vi "TC.vi"() -> ()   [LabVIEW 2013]
uses:
  Lib/Lib.llb/CS mode.ctl
  Lib/Lib.llb/R.ctl
  Lib/Lib.llb/T.ctl
  Lib/Lib.llb/Calibrations.ctl
  Lib/Lib.llb/CS.lvclass
  Lib/Lib.llb/PID Settings.ctl
  Lib/Lib.llb/AVS_exc_n_ranges.ctl
  Lib/Lib.llb/AVS_excitation.ctl
  Lib/Lib.llb/AVS47_range.ctl
  Lib/Lib.llb/Ch descriptions.ctl
  Lib/Lib.llb/Cursor Controls.ctl
  Lib/Lib.llb/DataArray.ctl
  Lib/Lib.llb/Unit.ctl
  Lib/Lib.llb/Control 6.ctl
  Lib/Lib.llb/Control 4.ctl
  Lib/Lib.llb/Control 8.ctl
  Lib/Lib.llb/VI FPO Ref.ctl
  Lib/support/Class ID ENUM.ctl
  Lib/Lib.llb/Type Descriptor Enumeration__ogtk.ctl
  Lib/Lib.llb/Refnum Subtype Enum__ogtk.ctl
  Lib/Lib.llb/Waveform Subtype Enum__ogtk.ctl
  Lib/Lib.llb/LV Data cluster.ctl
  Lib/Lib.llb/Action.ctl
  Write to DSC/TC to DSC/Typedefs/TC-cluster.ctl
  Lib/Lib.llb/TCS.lvclass
  Lib/Lib.llb/QCS.lvclass
  Lib/Lib.llb/CS Emulation.lvclass
  Lib/Lib.llb/PCS.lvclass
  Lib/Lib.llb/Byte Params.ctl
  Lib/Lib.llb/MView.lvlib
panel:
  out "R Array":dbl[](array[numeric])
  out "_SetControl":T1
  out "ControlNames":string[](array[string])
  out "VIRef":T2 {"Array DataType" format="%.0x"; "WaveForm Type" format="%.0x"; "RefNum Type" format="%.0x"; "DataType" format="%.0x"}
  out "VI called?":bool=TRUE
  out "Error code":u8
  out "_zBridgeSetNr":u8 caption="zBridge set nr."
  out "_zBridgeDll":path=path "C:/Users/Sasha/Dropbox/Labview/LC Software/ImpSoft-V5.2.2-multithreaded/ImpBridgeLabview/ImpBridgeDll.dll"
  in  "_String":string="^ Click the Run button to start the program "
  in  "Top Toolbar":enum32{"Page 1", "Page 2"}(tab)
  in  "Load config":bool
  in  "Start":bool
  in  "Load Data":bool
  in  "Pause":bool
  in  "Stop":bool
  in  "Copy to Clipboard":bool
  in  "Save config":bool
  in  "Clear all plots":bool
  in  "ColorBox":enum32{"Page 1", "Page 2"}(tab)
  in  "Colors":picture
  out "Color":u32(colorbox)
  in  "Graph-open popup":bool
  out "_CalibFilesPath":path=path "C:/avs-47/aaaa"
  out "_LogFilesPath":path
  out "_AVS_VISA":refnum<visa-resource-name>="COM3"
  in  "Minimize UI 2":bool
  out "VI Version":string="TC" caption="V"
  in  "Minimize UI 1":bool
  in  "Main Panel":enum32{"AVS"}(tab)
  in  "Graph Controls Bar":enum32{"Page 1"}(tab)
  in  "Mode Buttons":T7
  in  "Erase all":bool
  in  "Plot-Save All":bool
  in  "Plot-save-screen":bool
  in  "Channels Panel":T8(tab)=enum."All"
  out "T0":dbl=nan caption="T" format="%#.2p"
  out "R0":dbl caption="R" format="%.3p"
  out "R-Plot 0":cluster{dbl[], dbl[]}(graph) caption="R-Plot"
  out "T1":dbl=nan caption="T" format="%#.2p"
  out "R1":dbl caption="R" format="%.3p"
  out "R-Plot 1":cluster{dbl[], dbl[]}(graph) caption="R-Plot"
  out "T2":dbl=nan caption="T" format="%#.2p"
  out "R2":dbl caption="R" format="%.3p"
  out "R-Plot 2":cluster{dbl[], dbl[]}(graph) caption="R-Plot"
  out "T3":dbl=nan caption="T" format="%#.2p"
  out "R3":dbl caption="R" format="%.3p"
  out "R-Plot 3":cluster{dbl[], dbl[]}(graph) caption="R-Plot"
  out "T4":dbl=nan caption="T" format="%#.2p"
  out "R4":dbl caption="R" format="%.3p"
  out "R-Plot 4":cluster{dbl[], dbl[]}(graph) caption="R-Plot"
  out "T5":dbl=nan caption="T" format="%#.2p"
  out "R5":dbl caption="R" format="%.3p"
  out "R-Plot 5":cluster{dbl[], dbl[]}(graph) caption="R-Plot"
  out "T6":dbl=nan caption="T" format="%#.2p"
  out "R6":dbl caption="R" format="%.3p"
  out "R-Plot 6":cluster{dbl[], dbl[]}(graph) caption="R-Plot"
  out "T7":dbl=nan caption="T" format="%#.2p"
  out "R7":dbl caption="R" format="%.3p"
  out "R-Plot 7":cluster{dbl[], dbl[]}(graph) caption="R-Plot"
  out "T8":dbl=nan caption="T" format="%#.2p"
  out "R8":dbl caption="R" format="%.3p"
  out "R-Plot 8":cluster{dbl[], dbl[]}(graph) caption="R-Plot"
  out "T9":dbl=nan caption="T" format="%#.2p"
  out "R9":dbl caption="R" format="%.3p"
  out "R-Plot 9":cluster{dbl[], dbl[]}(graph) caption="R-Plot"
  out "T Cluster":T9 {"T9" format="%.2p"; "T8" format="%.2p"; "T7" format="%.2p"; "T6" format="%.2p"; "T5" format="%.2p"; "T4" format="%.2p"; "T3" format="%.2p"; "T2" format="%.2p"; "T1" format="%.2p"; "T0" format="%.2p"}
  in  "Sensor Names":T10={"AVS Name 0"="C_still", "AVS Name 1"="3K", "AVS Name 2"="Still", "AVS Name 3"="50mK", "AVS Name 4"="MC", "AVS Name 5"="MC", "AVS Name 6"="MC", "AVS Name 7"="", "AVS Name 8"="", "AVS Name 9"=""}
  in  "Edit Calibrations":T11
  in  "Sensor Calibrations":T12 {"Sensor 10" items=["No Calibration", "PT100", "PT1000", "RuO2 10k", "RuO2 1k5", "RuO2 2k", "Emulation R", "PT 1000", "RuO2-10K-NEW", "testCMN", "No Calibration"]; "Sensor 9" items=["No Calibration", "PT100", "PT1000", "RuO2 10k", "RuO2 1k5", "RuO2 2k", "Emulation R", "PT 1000", "RuO2-10K-NEW", "testCMN", "No Calibration"]; "Sensor 8" items=["No Calibration", "PT100", "PT1000", "RuO2 10k", "RuO2 1k5", "RuO2 2k", "Emulation R", "PT 1000", "RuO2-10K-NEW", "testCMN", "No Calibration"]; "Sensor 7" items=["No Calibration", "PT100", "PT1000", "RuO2 10k", "RuO2 1k5", "RuO2 2k", "Emulation R", "PT 1000", "RuO2-10K-NEW", "testCMN", "No Calibration"]; "Sensor 6" items=["No Calibration", "PT100", "PT1000", "RuO2 10k", "RuO2 1k5", "RuO2 2k", "Emulation R", "PT 1000", "RuO2-10K-NEW", "testCMN", "No Calibration"]; "Sensor 5" items=["No Calibration", "PT100", "PT1000", "RuO2 10k", "RuO2 1k5", "RuO2 2k", "Emulation R", "PT 1000", "RuO2-10K-NEW", "testCMN", "No Calibration"]; "Sensor 4" items=["No Calibration", "PT100", "PT1000", "RuO2 10k", "RuO2 1k5", "RuO2 2k", "Emulation R", "PT 1000", "RuO2-10K-NEW", "testCMN", "No Calibration"]; "Sensor 3" items=["No Calibration", "PT100", "PT1000", "RuO2 10k", "RuO2 1k5", "RuO2 2k", "Emulation R", "PT 1000", "RuO2-10K-NEW", "testCMN", "No Calibration"]; "Sensor 2" items=["No Calibration", "PT100", "PT1000", "RuO2 10k", "RuO2 1k5", "RuO2 2k", "Emulation R", "PT 1000", "RuO2-10K-NEW", "testCMN", "No Calibration"]; "Sensor 1" items=["No Calibration", "PT100", "PT1000", "RuO2 10k", "RuO2 1k5", "RuO2 2k", "Emulation R", "PT 1000", "RuO2-10K-NEW", "testCMN", "No Calibration"]}
  out "Units":T13
  out "R Cluster":T14={"R0"=0.0, "R1"=0.0, "R2"=-0.0, "R3"=0.0, "R4"=0.0, "R5"=0.0, "R6"=0.0, "R7"=0.0, "R8"=0.0, "R9"=0.0} {"R9" format="%.3p"; "R8" format="%.3p"; "R7" format="%.3p"; "R6" format="%.3p"; "R5" format="%.3p"; "R4" format="%.3p"; "R3" format="%.3p"; "R2" format="%.3p"; "R1" format="%.3p"; "R0" format="%.3p"}
  in  "AVS Scan Parameters":enum32{"Page 1", "Page 2"}(tab)
  in  "AVS Exc&Ranges":T15={"Excitation 0"=4, "Excitation 1"=4, "Excitation 2"=3, "Excitation 3"=3, "Excitation 4"=3, "Excitation 5"=3, "Excitation 6"=3, "Excitation 7"=3, "Range 0"=5, "Range 1"=5, "Range 2"=5, "Range 3"=5, "Range 4"=5, "Range 5"=5, "Range 6"=5, "Range 7"=5} {"Range 7" items=["n.a."=-1, "open"=0, "2 Ohm"=1, "20 Ohm"=2, "200 Ohm"=3, "2k Ohm"=4, "20k Ohm"=5, "200k Ohm"=6, "2M Ohm"=7]; "Range 6" items=["n.a."=-1, "open"=0, "2 Ohm"=1, "20 Ohm"=2, "200 Ohm"=3, "2k Ohm"=4, "20k Ohm"=5, "200k Ohm"=6, "2M Ohm"=7]; "Range 5" items=["n.a."=-1, "open"=0, "2 Ohm"=1, "20 Ohm"=2, "200 Ohm"=3, "2k Ohm"=4, "20k Ohm"=5, "200k Ohm"=6, "2M Ohm"=7]; "Range 4" items=["n.a."=-1, "open"=0, "2 Ohm"=1, "20 Ohm"=2, "200 Ohm"=3, "2k Ohm"=4, "20k Ohm"=5, "200k Ohm"=6, "2M Ohm"=7]; "Range 3" items=["n.a."=-1, "open"=0, "2 Ohm"=1, "20 Ohm"=2, "200 Ohm"=3, "2k Ohm"=4, "20k Ohm"=5, "200k Ohm"=6, "2M Ohm"=7]; "Range 2" items=["n.a."=-1, "open"=0, "2 Ohm"=1, "20 Ohm"=2, "200 Ohm"=3, "2k Ohm"=4, "20k Ohm"=5, "200k Ohm"=6, "2M Ohm"=7]; "Range 1" items=["n.a."=-1, "open"=0, "2 Ohm"=1, "20 Ohm"=2, "200 Ohm"=3, "2k Ohm"=4, "20k Ohm"=5, "200k Ohm"=6, "2M Ohm"=7]; "Range 0" items=["n.a."=-1, "open"=0, "2 Ohm"=1, "20 Ohm"=2, "200 Ohm"=3, "2k Ohm"=4, "20k Ohm"=5, "200k Ohm"=6, "2M Ohm"=7]; "Excitation 7" items=["none", "3 µV", "10 µV", "30 µV", "100 µV", "300 µV", "1 mV", "3 mV"]; "Excitation 6" items=["none", "3 µV", "10 µV", "30 µV", "100 µV", "300 µV", "1 mV", "3 mV"]; "Excitation 5" items=["none", "3 µV", "10 µV", "30 µV", "100 µV", "300 µV", "1 mV", "3 mV"]; "Excitation 4" items=["none", "3 µV", "10 µV", "30 µV", "100 µV", "300 µV", "1 mV", "3 mV"]; "Excitation 3" items=["none", "3 µV", "10 µV", "30 µV", "100 µV", "300 µV", "1 mV", "3 mV"]; "Excitation 2" items=["none", "3 µV", "10 µV", "30 µV", "100 µV", "300 µV", "1 mV", "3 mV"]; "Excitation 1" items=["none", "3 µV", "10 µV", "30 µV", "100 µV", "300 µV", "1 mV", "3 mV"]; "Excitation 0" items=["none", "3 µV", "10 µV", "30 µV", "100 µV", "300 µV", "1 mV", "3 mV"]}
  out "zBridge.Scan Phase":T18
  out "zBridge params":T19
  out "uPlots":T20
  out "zBridge.Active Channels":T21={"active Channel 0"=TRUE, "active Channel 1"=TRUE, "active Channel 2"=TRUE, "active Channel 3"=FALSE, "active Channel 4"=FALSE, "active Channel 5"=FALSE, "active Channel 6"=FALSE, "active Channel 7"=FALSE, "active Channel 8"=FALSE, "active Channel 9"=FALSE}
  out "Waveform Chart":T22(graph)
  in  "_CS_Address":u32
  in  "Edit calibration":bool
  in  "Convert R-T":bool
  out "T7":dbl caption="T=" format="%#.2p"
  in  "QuickR":dbl caption="R=" format="%_6g"
  in  "_QuickConvertCal":u16(ring) items=["No Calibration", "PT100", "PT1000", "RuO2 10k", "RuO2 1k5", "RuO2 2k", "Emulation R", "PT 1000", "RuO2-10K-NEW", "testCMN", "No Calibration"]
  out "_CSMode1List[i]":T23[](array[typedef]) caption="I_list[i]" min=-1.0
  out "CS.Automode Current":T23[](array[typedef]) min=-1.0
  in  "Lower Panel":enum32{"Page 1", "Page 2"}(tab)
  in  "Data History/RT Settings":enum32{"History", "Settings"}(tab)=enum."Settings"
  out "AVS names small":T10={"AVS Name 0"="3K", "AVS Name 1"="Still", "AVS Name 2"="50 mK", "AVS Name 3"="MC", "AVS Name 4"="MC", "AVS Name 5"="", "AVS Name 6"="", "AVS Name 7"="", "AVS Name 8"="", "AVS Name 9"=""}
  out "zBridge.Active channel":T24
  out "Small T Cluster":T25 caption="T" {"T0" format="%#.2p"; "T1" format="%#.2p"; "T2" format="%#.2p"; "T3" format="%#.2p"; "T4" format="%#.2p"; "T5" format="%#.2p"; "T6" format="%#.2p"; "T7" format="%#.2p"; "T8" format="%#.2p"; "T9" format="%#.2p"}
  out "Small R Cluster":T26 caption="R" {"R0" format="%#_5p"; "R1" format="%#_5p"; "R2" format="%#_5p"; "R3" format="%#_5p"; "R4" format="%#_5p"; "R5" format="%#_5p"; "R6" format="%#_5p"; "R7" format="%#_5p"; "R8" format="%#_5p"; "R9" format="%#_5p"}
  out "Time":dbl format="%<%X\n%x>T"
  in  "Runtime Settings":T27={"Read AVS channels from"=0, "Last Channel"=7, "Delay Between Scans"=0, "Stabilisation Delay"=5.0, "Averages"=2, "Data Memory"=25000, "Filter Graphs"=FALSE, "Y_min"=0.0, "Y_max"=2000000.0, "Plot type"=enum."T vs Time", "Allow neg R"=TRUE, "Miniplot Time"=30.0} {"Miniplot Time" min=0.0; "Delay Between Scans" format="%.0f s"; "Averages" min=1 max=1000; "Stabilisation Delay" min=0.5; "Last Channel" min=0 max=7 step=1; "Read AVS channels from" min=0 max=7 step=1; "Y_max" format="%#_6f"; "Y_min" min=0.0 format="%#_6f"; "Data Memory" min=3 max=50000}
  out "CS.Current Value":dbl[](array[numeric])
  in  "Data Array":T28=[{"R"=[], "T"=[], "Time"=[]}, {"R"=[0.0, 2.0], "T"=[], "Time"=[]}]
  out "T Array":dbl[](array[numeric])
  in  "_ScanData":dbl[](array[numeric])
  out "_I3SetPnt":dbl
  out "_CurrentsChanged":bool
  in  "_AVSRanges":T29={"Excitationl 0"=5, "Excitation 1"=5, "Excitation 2"=5, "Excitation 3"=5, "Excitation 4"=5, "Excitation 5"=5, "Excitation 6"=5, "Excitation 7"=5} caption="Ranges" {"Excitation 7" items=["n.a."=-1, "open"=0, "2 Ohm"=1, "20 Ohm"=2, "200 Ohm"=3, "2k Ohm"=4, "20k Ohm"=5, "200k Ohm"=6, "2M Ohm"=7]; "Excitation 6" items=["n.a."=-1, "open"=0, "2 Ohm"=1, "20 Ohm"=2, "200 Ohm"=3, "2k Ohm"=4, "20k Ohm"=5, "200k Ohm"=6, "2M Ohm"=7]; "Excitation 5" items=["n.a."=-1, "open"=0, "2 Ohm"=1, "20 Ohm"=2, "200 Ohm"=3, "2k Ohm"=4, "20k Ohm"=5, "200k Ohm"=6, "2M Ohm"=7]; "Excitation 4" items=["n.a."=-1, "open"=0, "2 Ohm"=1, "20 Ohm"=2, "200 Ohm"=3, "2k Ohm"=4, "20k Ohm"=5, "200k Ohm"=6, "2M Ohm"=7]; "Excitation 3" items=["n.a."=-1, "open"=0, "2 Ohm"=1, "20 Ohm"=2, "200 Ohm"=3, "2k Ohm"=4, "20k Ohm"=5, "200k Ohm"=6, "2M Ohm"=7]; "Excitation 2" items=["n.a."=-1, "open"=0, "2 Ohm"=1, "20 Ohm"=2, "200 Ohm"=3, "2k Ohm"=4, "20k Ohm"=5, "200k Ohm"=6, "2M Ohm"=7]; "Excitation 1" items=["n.a."=-1, "open"=0, "2 Ohm"=1, "20 Ohm"=2, "200 Ohm"=3, "2k Ohm"=4, "20k Ohm"=5, "200k Ohm"=6, "2M Ohm"=7]; "Excitationl 0" items=["n.a."=-1, "open"=0, "2 Ohm"=1, "20 Ohm"=2, "200 Ohm"=3, "2k Ohm"=4, "20k Ohm"=5, "200k Ohm"=6, "2M Ohm"=7]}
  out "_CSClassRef":refnum<class "CS.lvclass">
  in  "CS Indicators Panel":enum32{"Page 1", "Page 2"}(tab)
  out "CS.Automode 0":bool
  out "CS.Automode 1":bool
  out "QCS. I0 Mapping":T30(ring) caption="Output to"
  in  "uA 0":u32
  in  "CS Cannel Names":T31={"CS Name 0"="N.C.", "CS Name 1"="3K", "CS Name 2"="Still", "CS Name 3"="MC"}
  out "I0":T32={"uA"="000", "ON"=FALSE, "Gated"=FALSE, "current flows"=FALSE, "Error"=FALSE} caption="Ch0 -"
  in  "uA 3":u32
  in  "uA 2":u32
  in  "uA 1":u32
  out "CS.Automode 3":bool
  out "CS.Automode 2":bool
  out "I3":T32={"uA"="000", "ON"=FALSE, "Gated"=FALSE, "current flows"=FALSE, "Error"=FALSE} caption="Chn 3"
  out "I2":T32={"uA"="000", "ON"=FALSE, "Gated"=FALSE, "current flows"=FALSE, "Error"=FALSE} caption="Chn 2"
  out "I1":T32={"uA"="000", "ON"=FALSE, "Gated"=FALSE, "current flows"=FALSE, "Error"=FALSE} caption="Chn 1"
  out "_ExtVIReference":refnum<vi>
  out "Small I":cluster{"I1":dbl, "I2":dbl, "I3":dbl, "I4":dbl} caption="I" {"I1" format="%#.2f"; "I2" format="%#.2p"; "I3" format="%#.2p"; "I4" format="%#.2p"}
  out "CS.Actual Current":dbl[](array[numeric])
  in  "Save Data 2":bool
  in  "Show PID graph?":bool
  in  "Set Color":bool
  out "_ZBridgeUnit":string caption="Unit"
  out "_zBridgeParText":string caption="zBridge params/Error"
  out "_CurCalibrations":T33
  out "_LMBDown":bool
  in  "Side Panel":T34(tab)
  in  "Reload Calibrations":bool
  in  "zBridge settings":bool
  out "CS.ID":string
  out "CS status":errorcluster
  out "General Error":errorcluster caption="General status"
  in  "Bridge settings":T35={"Bridge Type"=enum."AVS47A (GPIB interface)", "AVS RS232 Port"="COM5", "AVS GPIB Address"="GPIB0::20::INSTR", "Calibrations Folder"=path "C:/LC Data/Calibrations"}
  in  "CS Settings":T36={"TCS RS232 Port"="COM1", "TCS_Imax"=5, "CS type"=enum."TCS", "CS.QCS Device Nr"=0}
  in  "Data Logging Settings":T37={"Log Files Folder"=path "C:/LC Data/Data", "Log Files Name"="LogAVS", "Automode Files Name"="calibration", "Filenames Suffix"="_%Y-%m-%d-%H-%M-%S", "Delimeter"="\t", "New File Interval"=7, "New File Interval Units"=enum."Days", "Date Format"="%Y-%m-%d %H:%M:%S", "External VI Path"=path "", "Query Description"=FALSE, "Run Description"="\n"}
  out "Bridge status":errorcluster
  in  "CS.QCS I0 Output":T38(ring) caption="Set Channel 0 output to"
  in  "CS.Mode":T39 caption="CS mode"
  out "_TimeOld":dbl format="%#_16g"
  in  "CS Modes Panel":T40(tab)=enum."Automatic 1"
  in  "CS.I3":T41={"Toggle ON/OFF"=FALSE, "Toggle Gated"=FALSE, "I"=0, "Range"=enum."x1 uA"} caption="Chn 3" {"I" max=100000 step=1}
  in  "CS.I2":T41={"Toggle ON/OFF"=FALSE, "Toggle Gated"=FALSE, "I"=0, "Range"=enum."x1 uA"} caption="Chn 2" {"I" max=100000 step=1}
  in  "CS.I1":T41={"Toggle ON/OFF"=FALSE, "Toggle Gated"=FALSE, "I"=0, "Range"=enum."x1 uA"} caption="Chn 1" {"I" max=100000 step=1}
  in  "CS.I0":T41={"Toggle ON/OFF"=FALSE, "Toggle Gated"=FALSE, "I"=0, "Range"=enum."x1 uA"} caption="Chn 0" {"I" max=100000 step=1}
  in  "CS.Mode1.PID Settings":T42={"FB on 2"=enum."3", "Proportional Gain"=3.0, "Integral Gain"=3.0, "Derivative Gain"=1.0, "Deadband"=0.1, "Feed Fwd Gain [uA/mK]"=0.0, "Integral Gain Bandwidth"=10.0, "Integral Gain Background"=1.0, "Current limit, [uA]"=1.0} {"Integral Gain Background" format="%#.6g"; "Integral Gain Bandwidth" format="%#.6g"; "Feed Fwd Gain [uA/mK]" format="%#.5g"; "Deadband" format="%#.5g"; "Derivative Gain" format="%#.6g"; "Integral Gain" format="%#.6g"; "Proportional Gain" format="%#.6g"; "Current limit, [uA]" format="%#.5g"}
  in  "CS.Mode1.Start":bool
  in  "CS.Mode1.List":T23[][](array[typedef]) min=-1.0
  out "CS.Mode1.PID Column":T43[](array[typedef])
  out "CS.Mode1.Row":T44[](array[typedef])=[TRUE, FALSE, FALSE, FALSE, FALSE, FALSE, FALSE, FALSE, FALSE, FALSE]
  out "CS.Mode1.PID Stabilized?":bool caption="SP reached?"
  out "CS.Mode1.PID Error":dbl=10.0 caption="Error" format="%#_6f"
  out "CS.Mode1.Slope":dbl caption="Slope" format="%#_3g %"
  out "CS.Mode1.Timer":dbl caption="Timer" format="%<%H:%M:%S>t"
  out "CS.Mode1.List:Count":i32=10 caption="/"
  out "CS.Mode1.List:Index":i32=10 caption="Point #"
  in  "CS.Mode1.Next":bool
  in  "CS.Mode1.Reset PID":bool
  in  "CS.Mode1.Auto Advance":bool=TRUE caption="Enable automatic sweeping/list iteration"
  in  "CS.Mode1.Settings":T45={"Bridge Channel"=0, "N averages"=10, "Delay Time"=10.0, "T stability"=0.3, "FB on"=enum."Temperature"} {"Delay Time" min=0.0 format="%#_g min"; "Bridge Channel" min=-1 max=9 step=1}
  in  "CS.Mode1.Call VI?":bool caption="Call Ext. VI"
  out "CS.Mode1.VI State":T46(ring) caption="- state"
  in  "CS.Mode1.Trigger all TC":bool caption="Trigger other running TC instances"
  in  "CS.Mode1.List:Prev":bool
  in  "CS.Mode1.List:Next":bool
  in  "CS.Mode1.List:To First":bool
  in  "CS.Mode1.List:Save":bool
  in  "CS.Mode1.List:Load":bool
  in  "CS.Mode1.Write To Log":bool
  in  "CS.Mode1.PID":cluster{"Enabled":bool}
  in  "CS.Mode1.List:Clear":bool
  in  "CS.Mode2.Settings":T47={"FB on"=enum."Temperature", "Bridge Channel"=0, "Hysteresis"=10} {"Hysteresis" max=100 format="%.0f %%"; "Bridge Channel" min=-1 max=9 step=1}
  in  "CS.Mode2.Start":bool
  in  "CS.Mode2.Add Row":bool
  in  "CS.Mode2.New Row":dbl[](array[numeric])=[0.0, 0.0, 0.0, 0.0, 0.0, 0.0] caption="New range" min=-1.0
  in  "CS.Mode2.List":dbl[][](array[numeric])=[[0.0, 0.0, 0.0, 0.0, 0.0, inf]] min=-1.0
  out "CS.Mode2.Row":T44[](array[typedef])=[TRUE, FALSE, FALSE, FALSE, FALSE, FALSE, FALSE, FALSE, FALSE, FALSE]
  in  "T Sweep":T48={"Start value"=200.0, "End value"=250.0, "Step"=10.0, "Current"=0.0, "I_next"=FALSE, "I_prev"=FALSE, "Interrrupt Sweep"=FALSE, "Start"=FALSE, "Boolean"=TRUE} {"Step" min=0.0; "End value" min=0.0; "Start value" min=0.0}
  # "Quick convert R->T:"
  # "Ohm"
  # "mK"
  # "Ch#"
  # "Miniplot"
  # "Channel parameters"
  # "Impedance"
  # "Unit"
  # "Type of sensor"
  # "T [mK]"
  # "Description"
  # "0"
  # "1"
  # "2"
  # "3"
  # "4"
  # "5"
  # "6"
  # "7"
  # "8"
  # "9"
  # "0"
  # "1"
  # "2"
  # "3"
  # "4"
  # "5"
  # "7"
  # "8"
  # "9"
  # "6"
  # "auto"
  # "auto"
  # "auto"
  # "auto"
  # "gated"
  # "gated"
  # "gated"
  # "gated"
  # "Status"
  # "Current source mode"
  # "Current source manual control"
  # "Current source automatic mode #1"
  # "Currents List"
  # "Settings"
  # "I0"
  # "I1"
  # "I2"
  # "I3"
  # "Status"
  # "On temperature stabilized"
  # "Current source automatic mode #2"
  # "Currents List"
  # "Settings"
  # "T0"
  # "T1"
  # "I0"
  # "I1"
  # "I2"
  # "I3"
  # "T0"
  # "T1"
  # "I0"
  # "I1"
  # "I2"
  # "I3"
  # "Ch3"
types:
  T1 = typedef "MView.lvlib/LV Data cluster.ctl" = cluster{"Name":string, "Scalar":string, "Array":string[][]}
  T2 = typedef "MView.lvlib/VI FPO Ref.ctl" = cluster{"Control Ref ID":refnum<vi>[], "Full Name":string[], "ClassID":T3[], "Short Name":string[], "DataType":T4[], "RefNum Type":T5[], "WaveForm Type":T6[], "Parent":i32[], "Array DataType":T4[], "Owning VI":refnum<vi>[], "Active?":bool[]}
  T3 = typedef "Class ID ENUM.ctl" = enum16{"<Null>", "1", "2", "Generic", "Decoration", "Text", "Control", "ColorBox", "Boolean", "RefNum", "Variant", "Path", "ListBox", "Table", "Array", "Picture", "ActiveXContainer", "Numeric", "Digital", "NamedNumeric", "ColorRamp", "Slide", "GraphOrChart", "WaveformChart", "WaveformGraph", "IntensityChart", "IntensityGraph", "String", "IOName", "ComboBox", "Cluster", "Panel", "Knob", "NumWithScale", "Ring", "Enum", "GObject", "Plot", "Cursor", "NumericText", "Scale", "ColorScale", "GraphScale", "ColorGraphScale", "TypedRefNum", "OldKnobScale", "MCListbox", "MeasureData", "BVTag", "DAQName", "VISAName", "IVIName", "SlideScale", "TabControl", "Page", "TabArrayTabControl", "ConPane", "57", "58", "59", "60", "61", "62", "63", "64", "SubPanel", "TreeControl", "67", "68", "69", "70", "71", "72", "73", "74", "75", "SplitterBar"}
  T4 = typedef "Type Descriptor Enumeration__ogtk.ctl" = enum8{"<Null>", "I8", "I16", "I32", "I64", "U8", "U16", "U32", "U64", "SGL", "DBL", "EXT", "CSG", "CDB", "CXT", "0x0F", "0x10", "0x11", "0x12", "0x13", "0x14", "Enum U8", "Enum U16", "Enum U32", "Enum U64", "SGL PQ", "DBL PQ", "EXT PQ", "CSG PQ", "CDB PQ", "CXT PQ", "0x1F", "0x20", "Boolean", "0x22", "0x23", "0x24", "0x25", "0x26", "0x27", "0x28", "0x29", "0x2A", "0x2B", "0x2C", "0x2D", "0x2E", "0x2F", "String", "0x31", "Path", "Pict", "0x34", "0x35", "0x36", "DAQ", "0x38", "0x39", "0x3A", "0x3B", "0x3C", "0x3D", "0x3E", "0x3F", "Array", "0x41", "0x42", "0x43", "0x44", "0x45", "0x46", "0x47", "0x48", "0x49", "0x4A", "0x4B", "0x4C", "0x4D", "0x4E", "0x4F", "Cluster", "0x51", "0x52", "Variant", "Waveform", "0x55", "0x56", "0x57", "0x58", "0x59", "0x5A", "0x5B", "0x5C", "0x5D", "0x5E", "0x5F", "0x60", "0x61", "0x62", "0x63", "0x64", "0x65", "0x66", "0x67", "0x68", "0x69", "0x6A", "0x6B", "0x6C", "0x6D", "0x6E", "0x6F", "Refnum"}
  T5 = typedef "Refnum Subtype Enum__ogtk.ctl" = enum8{"Generic", "Datalog File Refnum", "Byte Stream File Refnum", "Device Refnum", "Occurence Refnum", "TCP Connection Refnum", "VISA Refnum (Obsolete)", "Automation Renum", "VI Server Refnum", "Menu Refnum", "IVI Refnum (Obsolete)", "IMAQ Session", "0x0C", "Datasocket Refnum", "VISA Resource", "IVI Logical Name", "UDP Connection Refnum", "Notifier Refnum", "Queue Refnum", "IrDA Refnum", "Hardware Plugin Refnum", "Hardware Plugin Tag Refnum", "DAQmx Refnum", "Event Registration Refnum", ".NET Refnum", "User Event Refnum", "0x1A", "Event Callback", "0x1C", "0x1D", "Only Used Internal to LabVIEW", "Bluetooth", "Data Value References", "RT FIFO", "TDM Streaming"}
  T6 = typedef "Waveform Subtype Enum__ogtk.ctl" = enum8{"<Not a Waveform Type>", "0x01", "Analog 16-bit signed", "Analog Double-Precision", "0x04", "Analog Single Precision", "Timestamp", "Digital Data", "Digital Waveform", "Dynamic Data", "Analog Extended-Precision", "Analog 8-bit unsigned", "Analog 16-bit unsigned", "Analog 32-bit unsigned", "Analog 8-bit signed", "Analog 32-bit signed", "Analog Complex Single-Precision", "Analog Complex Double-Precision", "Analog Complex Extended Precision", "Analog 64-bit signed", "Analog 64-bit unsigned"}
  T7 = typedef "Cursor Controls.ctl" = enum32{"No Selection", "Cursor mode", "Erase point", "Erase range"}
  T8 = enum32{"0", "1", "2", "3", "4", "5", "6", "7", "8", "9", "All", "PID loop"}
  T9 = typedef "T.ctl" = cluster{"T0":dbl, "T1":dbl, "T2":dbl, "T3":dbl, "T4":dbl, "T5":dbl, "T6":dbl, "T7":dbl, "T8":dbl, "T9":dbl}
  T10 = typedef "Ch descriptions.ctl" = cluster{"AVS Name 0":string, "AVS Name 1":string, "AVS Name 2":string, "AVS Name 3":string, "AVS Name 4":string, "AVS Name 5":string, "AVS Name 6":string, "AVS Name 7":string, "AVS Name 8":string, "AVS Name 9":string}
  T11 = cluster{"Boolean":bool, "Boolean 2":bool, "Boolean 3":bool, "Boolean 4":bool, "Boolean 5":bool, "Boolean 6":bool, "Boolean 7":bool, "Boolean 8":bool, "Boolean 9":bool, "Boolean 10":bool}
  T12 = typedef "Calibrations.ctl" = cluster{"Sensor 1":u16, "Sensor 2":u16, "Sensor 3":u16, "Sensor 4":u16, "Sensor 5":u16, "Sensor 6":u16, "Sensor 7":u16, "Sensor 8":u16, "Sensor 9":u16, "Sensor 10":u16}
  T13 = typedef "Unit.ctl" = cluster{"Value 0":string, "Value 1":string, "Value 2":string, "Value 3":string, "Value 4":string, "Value 5":string, "Value 6":string, "Value 7":string, "Value 8":string, "Value 9":string}
  T14 = typedef "R.ctl" = cluster{"R0":dbl, "R1":dbl, "R2":dbl, "R3":dbl, "R4":dbl, "R5":dbl, "R6":dbl, "R7":dbl, "R8":dbl, "R9":dbl}
  T15 = typedef "AVS_exc_n_ranges.ctl" = cluster{"Excitation 0":T16, "Excitation 1":T16, "Excitation 2":T16, "Excitation 3":T16, "Excitation 4":T16, "Excitation 5":T16, "Excitation 6":T16, "Excitation 7":T16, "Range 0":T17, "Range 1":T17, "Range 2":T17, "Range 3":T17, "Range 4":T17, "Range 5":T17, "Range 6":T17, "Range 7":T17}
  T16 = typedef "AVS_excitation.ctl" = i16
  T17 = typedef "AVS47_range.ctl" = i16
  T18 = cluster{"Value 0":dbl, "Value 1":dbl, "Value 2":dbl, "Value 3":dbl, "Value 4":dbl, "Value 5":dbl, "Value 6":dbl, "Value 7":dbl, "Value 8":dbl, "Value 9":dbl}
  T19 = cluster{"AVS Name 0":string, "AVS Name 1":string, "AVS Name 2":string, "AVS Name 3":string, "AVS Name 4":string, "AVS Name 5":string, "AVS Name 6":string, "AVS Name 7":string, "AVS Name 8":string, "AVS Name 9":string}
  T20 = cluster{"uPlot 0":cluster{dbl[], dbl[]}, "uPlot 1":cluster{dbl[], dbl[]}, "uPlot 2":cluster{dbl[], dbl[]}, "uPlot 3":cluster{dbl[], dbl[]}, "uPlot 4":cluster{dbl[], dbl[]}, "uPlot 5":cluster{dbl[], dbl[]}, "uPlot 6":cluster{dbl[], dbl[]}, "uPlot 7":cluster{dbl[], dbl[]}, "uPlot 8":cluster{dbl[], dbl[]}, "uPlot 9":cluster{dbl[], dbl[]}}
  T21 = cluster{"active Channel 0":bool, "active Channel 1":bool, "active Channel 2":bool, "active Channel 3":bool, "active Channel 4":bool, "active Channel 5":bool, "active Channel 6":bool, "active Channel 7":bool, "active Channel 8":bool, "active Channel 9":bool}
  T22 = cluster{"Ip":dbl, "Ii":dbl, "Id":dbl, "Iff":dbl, "I_tot":dbl}
  T23 = typedef "Control 4.ctl" = dbl
  T24 = cluster{"Boolean 5":bool, "Boolean 5":bool, "Boolean 5":bool, "Boolean 5":bool, "Boolean 5":bool, "Boolean 5":bool, "Boolean 5":bool, "Boolean 5":bool, "Boolean 5":bool, "Boolean 5":bool}
  T25 = cluster{"T0":dbl, "T1":dbl, "T2":dbl, "T3":dbl, "T4":dbl, "T5":dbl, "T6":dbl, "T7":dbl, "T8":dbl, "T9":dbl}
  T26 = cluster{"R0":dbl, "R1":dbl, "R2":dbl, "R3":dbl, "R4":dbl, "R5":dbl, "R6":dbl, "R7":dbl, "R8":dbl, "R9":dbl}
  T27 = cluster{"Read AVS channels from":i8, "Last Channel":i8, "Delay Between Scans":u32, "Stabilisation Delay":dbl, "Averages":u16, "Data Memory":u16, "Filter Graphs":bool, "Y_min":dbl, "Y_max":dbl, "Plot type":enum16{"R vs Time", "T vs Time"}, "Allow neg R":bool, "Miniplot Time":dbl}
  T28 = typedef "DataArray.ctl" = cluster{"R":dbl[], "T":dbl[], "Time":dbl[]}[]
  T29 = cluster{"Excitationl 0":i16, "Excitation 1":i16, "Excitation 2":i16, "Excitation 3":i16, "Excitation 4":i16, "Excitation 5":i16, "Excitation 6":i16, "Excitation 7":i16}
  T30 = enum16{"Chn 0", "Aux 0", "Aux 1", "Aux 2", "Aux 3"}
  T31 = cluster{"CS Name 0":string, "CS Name 1":string, "CS Name 2":string, "CS Name 3":string}
  T32 = cluster{"uA":string, "ON":bool, "Gated":bool, "current flows":bool, "Error":bool}
  T33 = cluster{"[0]":string, "[1]":string, "[2]":string, "[3]":string, "[4]":string, "[5]":string, "[6]":string, "[7]":string, "[8]":string, "[9]":string}
  T34 = enum32{"Devices Settings", "Current source control"}
  T35 = cluster{"Bridge Type":enum16{"AVS47A (GPIB interface)", "AVS47B (RS232 interface)", "AVS48SI (RS232 interface)", "AVS Emulation", "Impedance Bridge", "Disabled"}, "AVS RS232 Port":refnum<visa-resource-name>, "AVS GPIB Address":refnum<visa-resource-name>, "Calibrations Folder":path}
  T36 = cluster{"TCS RS232 Port":refnum<visa-resource-name>, "TCS_Imax":i32, "CS type":enum16{"TCS", "QCS v1", "PCS (n.a.)", "CS Emulation", "Disabled"}, "CS.QCS Device Nr":u16}
  T37 = cluster{"Log Files Folder":path, "Log Files Name":string, "Automode Files Name":string, "Filenames Suffix":string, "Delimeter":string, "New File Interval":u32, "New File Interval Units":enum16{"Minutes", "Hours", "Days"}, "Date Format":string, "External VI Path":path, "Query Description":bool, "Run Description":string}
  T38 = enum16{"Channel 0", "Aux 0", "Aux 1", "Aux 2", "Aux 3"}
  T39 = typedef "CS mode.ctl" = enum16{"Manual", "Mode 1", "Mode2"}
  T40 = enum32{"Manual", "Automatic 1", "Automatic 2", "Automatic 3"}
  T41 = cluster{"Toggle ON/OFF":bool, "Toggle Gated":bool, "I":u32, "Range":enum8{"Auto", "x1 uA", "x10 uA", "x100 uA", "x1 mA"}}
  T42 = typedef "PID Settings.ctl" = cluster{"FB on 2":enum16{"0", "1", "2", "3"}, "Proportional Gain":dbl, "Integral Gain":dbl, "Derivative Gain":dbl, "Deadband":dbl, "Feed Fwd Gain [uA/mK]":dbl, "Integral Gain Bandwidth":dbl, "Integral Gain Background":dbl, "Current limit, [uA]":dbl}
  T43 = typedef "Control 8.ctl" = bool
  T44 = typedef "Control 6.ctl" = bool
  T45 = cluster{"Bridge Channel":i32, "N averages":i32, "Delay Time":dbl, "T stability":dbl, "FB on":enum16{"Resistance", "Temperature"}}
  T46 = enum32{"Bad", "Idle", "Run top level", "Running"}
  T47 = cluster{"FB on":enum16{"Resistance", "Temperature"}, "Bridge Channel":i32, "Hysteresis":u8}
  T48 = cluster{"Start value":dbl, "End value":dbl, "Step":dbl, "Current":dbl, "I_next":bool, "I_prev":bool, "Interrrupt Sweep":bool, "Start":bool, "Boolean":bool}
  T49 = cluster{"UpdateChannelInfo":refnum<user-event>, "UpdateValuesAVS":refnum<user-event>, "UpdateCalibrations":refnum<user-event>, "UpdateLogFilePath":refnum<user-event>, "TempStabilized":refnum<user-event>, "Reset PID loop":refnum<user-event>, "UpdateValuesZBridge":refnum<user-event>, "CS Automode":refnum<user-event>, "CallExtVI":refnum<user-event>, "Data Array":refnum<user-event>}
  T50 = cluster{"Config folder":path, "Config File":path, "Calibrations Folder":path, "zBridge dll":path, "Variables Library":path}
  T51 = enum32{"Page Enabled", "Page Disabled", "Page Disabled & Grayed"}
  T52 = cluster{"error":bool, "code":i32, "source":string}
  T53 = typedef "Action.ctl" = enum16{"Init", "Write", "Read"}
  T54 = enum16{"AVS47A (GPIB interface)", "AVS47B (RS232 interface)", "AVS48", "AVS Emulation", "Impedance Bridge", "Disabled"}
  T55 = typedef "TC-cluster.ctl" = cluster{"R":dbl[], "T":dbl[], "I":dbl[], "AVS type":enum16{"AVS47A (GPIB interface)", "AVS47B (RS232 interface)", "AVS48", "AVS Emulation", "Impedance Bridge", "Disabled"}, "AVS names":cluster{"AVS Name 0":string, "AVS Name 1":string, "AVS Name 2":string, "AVS Name 3":string, "AVS Name 4":string, "AVS Name 5":string, "AVS Name 6":string, "AVS Name 7":string, "AVS Name 8":string, "AVS Name 9":string}, "Calibration":refnum<vi>[]}
  T56 = enum32{"No Selection", "Cursor mode", "Erase point", "Erase range"}
  T57 = enum16{"TCS", "QCS v1", "PCS (n.a.)", "CS Emulation", "Disabled"}
  T58 = enum8{"Auto", "x1 uA", "x10 uA", "x100 uA", "x1 mA"}
  T59 = cluster{"Cluster":cluster{"Time":dbl[], "T":dbl[]}, "Cluster":cluster{"Time":dbl[], "T":dbl[]}, "Cluster":cluster{"Time":dbl[], "T":dbl[]}, "Cluster":cluster{"Time":dbl[], "T":dbl[]}, "Cluster":cluster{"Time":dbl[], "T":dbl[]}, "Cluster":cluster{"Time":dbl[], "T":dbl[]}, "Cluster":cluster{"Time":dbl[], "T":dbl[]}, "Cluster":cluster{"Time":dbl[], "T":dbl[]}, "Cluster":cluster{"Time":dbl[], "T":dbl[]}, "Cluster":cluster{"Time":dbl[], "T":dbl[]}}
  T60 = enum32{"invalid app kind", "Development System", "Run Time System", "Student Edition", "Embedded LabVIEW", "Evaluation", "Custom"}
  T61 = enum16{"AVS47A (GPIB interface)", "AVS47B (RS232 interface)", "AVS48SI (RS232 interface)", "AVS Emulation", "Impedance Bridge", "Disabled"}
  T62 = cluster{"[0]":dbl, "[1]":dbl, "[2]":dbl, "[3]":dbl, "[4]":dbl, "[5]":dbl, "[6]":dbl, "[7]":dbl, "[8]":dbl, "[9]":dbl}
  T63 = cluster{"Temperature[0]":dbl, "Temperature[1]":dbl, "Temperature[2]":dbl, "Temperature[3]":dbl, "Temperature[4]":dbl, "Temperature[5]":dbl, "Temperature[6]":dbl, "Temperature[7]":dbl, "Temperature[8]":dbl, "Temperature[9]":dbl}
  T64 = cluster{"Current Time (double)":dbl, "R":dbl[], "T":dbl[]}
  T65 = typedef "File Info Record__ogtk.ctl" = cluster{"type":string, "creator":string, "permissions":i32, "data size":i32, "res size":i32, "creation date":u32, "modification date":u32, "bFolder":bool, "bInvisible":bool, "location":cluster{"vertical":i16, "horizontal":i16}, "owner":string, "group":string}
  T66 = cluster{"Units[0]":string, "Units[1]":string, "Units[2]":string, "Units[3]":string, "Units[4]":string, "Units[5]":string, "Units[6]":string, "Units[7]":string, "Units[8]":string, "Units[9]":string}
  T67 = cluster{"zBridge params[0]":string, "zBridge params[1]":string, "zBridge params[2]":string, "zBridge params[3]":string, "zBridge params[4]":string, "zBridge params[5]":string, "zBridge params[6]":string, "zBridge params[7]":string, "zBridge params[8]":string, "zBridge params[9]":string}
  T68 = cluster{"date/time string":string, "Value":dbl[], "Value":dbl[], "Value":dbl[]}
  T69 = typedef "imagedata.ctl" = cluster{"image type":i32, "image depth":i32, "image":u8[], "mask":u8[], "colors":u32[], "Rectangle":cluster{"left":i16, "top":i16, "right":i16, "bottom":i16}}
  T70 = typedef "LVPoint32TypeDef.ctl" = cluster{"Horizontal":i32, "Vertical":i32}
  T71 = cluster{"Shift":bool, "Ctrl":bool, "Alt":bool, "Cmd":bool, "Opt":bool}
  T72 = cluster{"Output Array":dbl[], "array w/ subset deleted":dbl[], "array w/ subset deleted":dbl[]}
  T73 = typedef "LVRectTypeDef.ctl" = cluster{"Left":i16, "Top":i16, "Right":i16, "Bottom":i16}
  T74 = typedef "Exc_n_Ranges.ctl" = cluster{"Excitationl 0":i16, "Excitation 1":i16, "Excitation 2":i16, "Excitation 3":i16, "Excitation 4":i16, "Excitation 5":i16, "Excitation 6":i16, "Excitation 7":i16, "Range 0":i16, "Range 1":i16, "Range 2":i16, "Range 3":i16, "Range 4":i16, "Range 5":i16, "Range 6":i16, "Range 7":i16}
  T75 = enum32{"HKEY_CLASSES_ROOT", "HKEY_CURRENT_USER", "HKEY_LOCAL_MACHINE", "HKEY_USERS", "HKEY_PERFORMANCE_DATA", "HKEY_CURRENT_CONFIG", "HKEY_DYN_DATA"}
  T76 = typedef "Byte Params.ctl" = enum8{"Active", "Channel Type", "Channel No", "Reference No", "RLC select", "Save Data", "L Inverted", "Menu Active"}
  T77 = typedef "LVPositionTypeDef.ctl" = cluster{"Left":i32, "Top":i32}
  T78 = cluster{"Range 0":i16, "Range 1":i16, "Range 2":i16, "Range 3":i16, "Range 4":i16, "Range 7":i16, "Range 5":i16, "Range 6":i16}
  T79 = cluster{"Range 0":i16, "Range 1":i16, "Range 2":i16, "Range 3":i16, "Range 4":i16, "Range 5":i16, "Range 6":i16, "Range 7":i16}
  T80 = cluster{"RANGE 0":u16, "RANGE 1":u16, "RANGE 2":u16, "RANGE 3":u16, "RANGE 4":u16, "RANGE 5":u16, "RANGE 6":u16, "RANGE 7":u16}
  T81 = typedef "LCR Channel parameters.ctl" = cluster{"Set_number":u8, "Set_char":u16, "Ch_number":u8, "Ch_type":u8, "Freq":dbl, "T_int":dbl, "I_exc":dbl, "V_exc":dbl, "SNR":dbl, "Vnoise":dbl, "P_diss":dbl}
  T82 = typedef "CS Data.ctl" = cluster{"Range":u8, "Current":dbl, "Current (string)":string, "On?":bool, "G?":bool, "I?":bool, "Err?":bool}
  T83 = typedef "TCS indicator.ctl" = cluster{"uA":string, " ON":bool, "Gated":bool, "current flows":bool, "Error":bool}
  T84 = cluster{"Toggle ON/OFF":bool, "Toggle Gated":bool}
  T85 = cluster{"Current":u32, "Range":enum16{"Auto", "x1 uA", "x10 uA", "x100 uA", "x1 mA"}}
  T86 = typedef "TCS manual control.ctl" = cluster{"Toggle ON/OFF":bool, "Toggle Gated":bool, "Current":u32, "Range":enum8{"Auto", "x1 uA", "x10 uA", "x100 uA", "x1 mA"}}
  T87 = cluster{"Status[0]":i32, "Status[1]":i32, "Status[2]":i32, "Status[3]":i32, "Status[4]":i32, "Status[5]":i32, "Status[6]":i32, "Status[7]":i32, "Status[8]":i32, "Status[9]":i32}
  T88 = cluster{"Active":bool, "Active":bool, "Active":bool, "Active":bool, "Active":bool, "Active":bool, "Active":bool, "Active":bool, "Active":bool, "Active":bool}
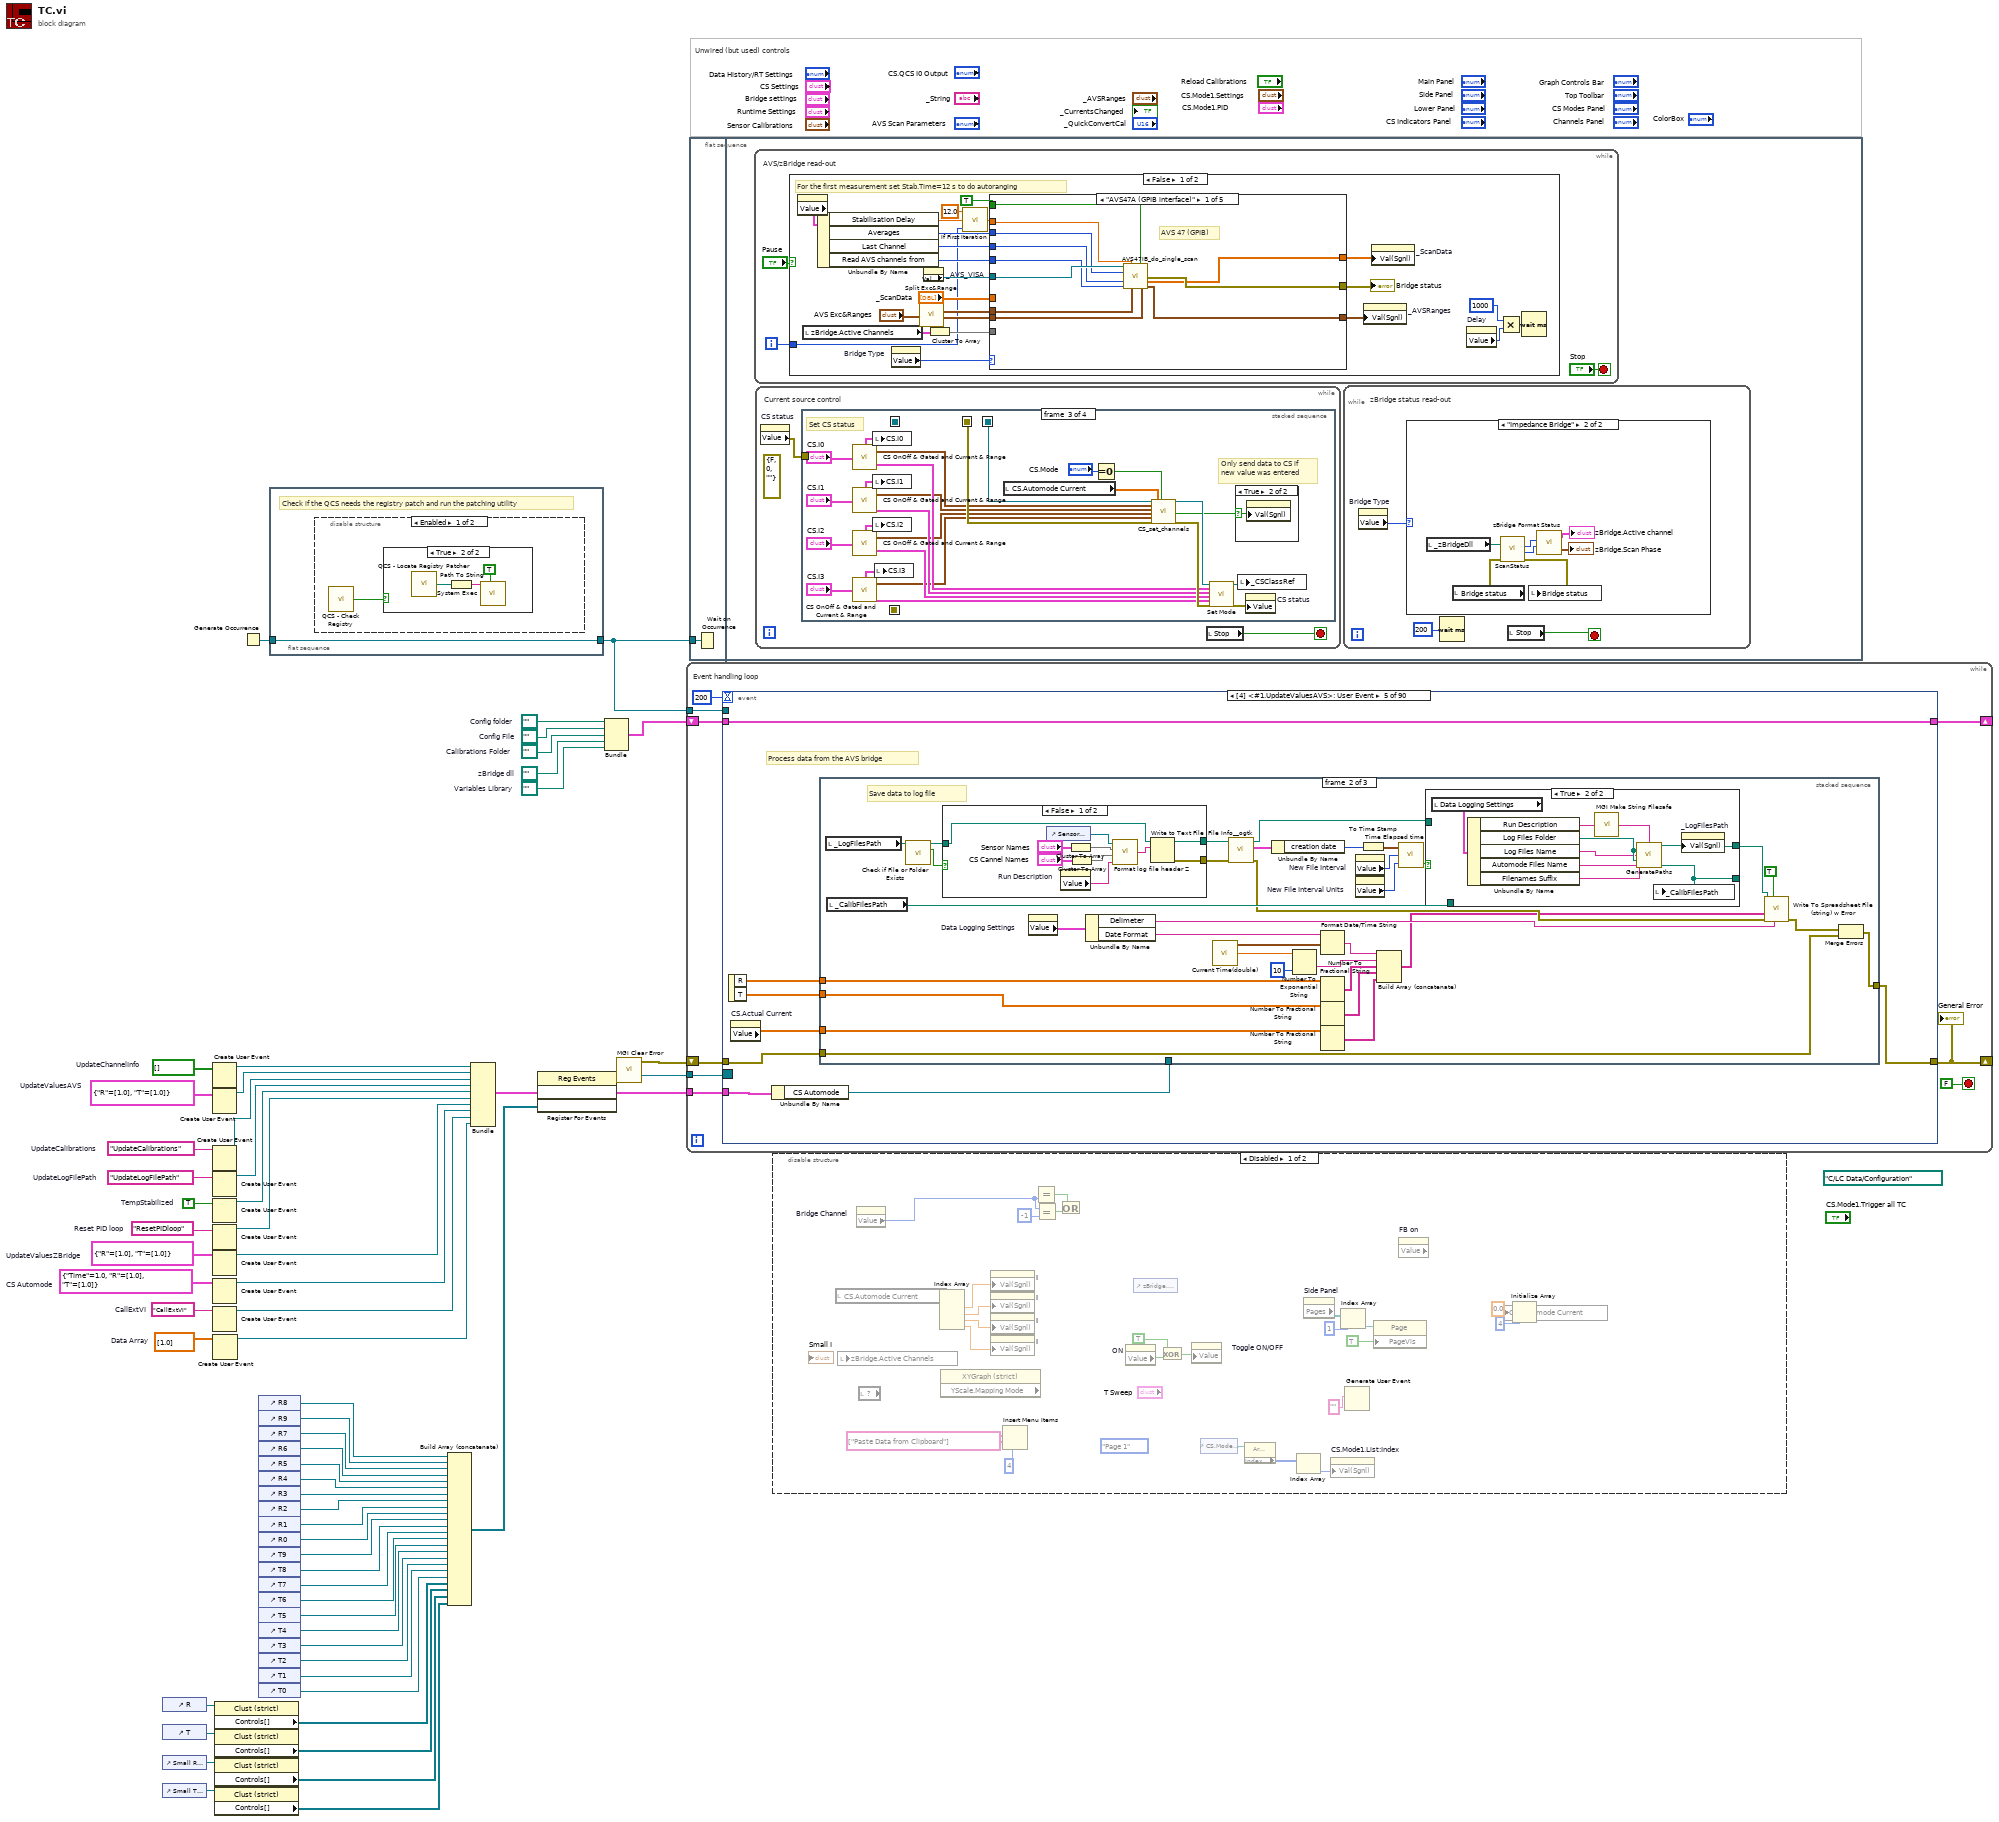
[diagram p0: block diagram]
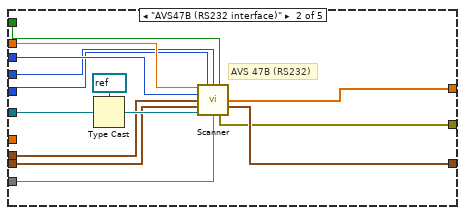
[diagram p5: hidden frame]
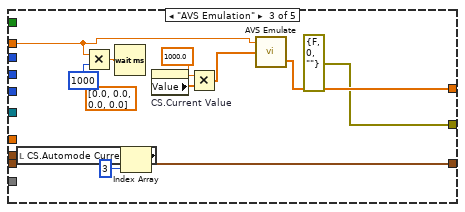
[diagram p6: hidden frame]
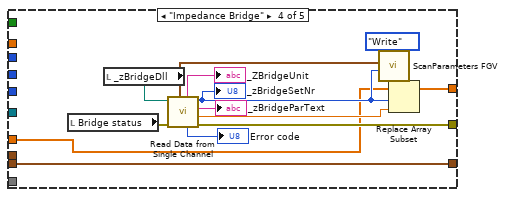
[diagram p7: hidden frame]
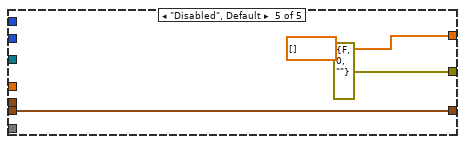
[diagram p8: hidden frame]
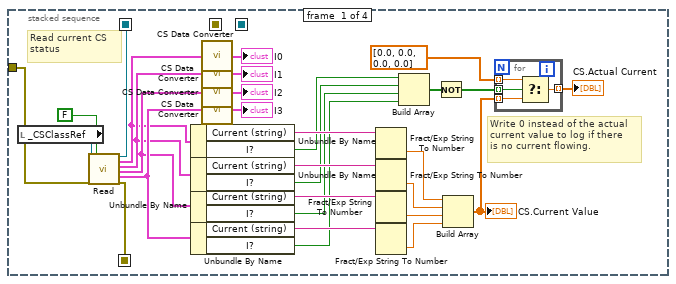
[diagram p10: hidden frame]
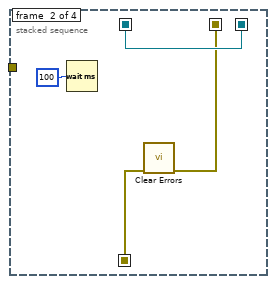
[diagram p11: hidden frame]
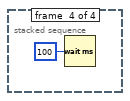
[diagram p13: hidden frame]
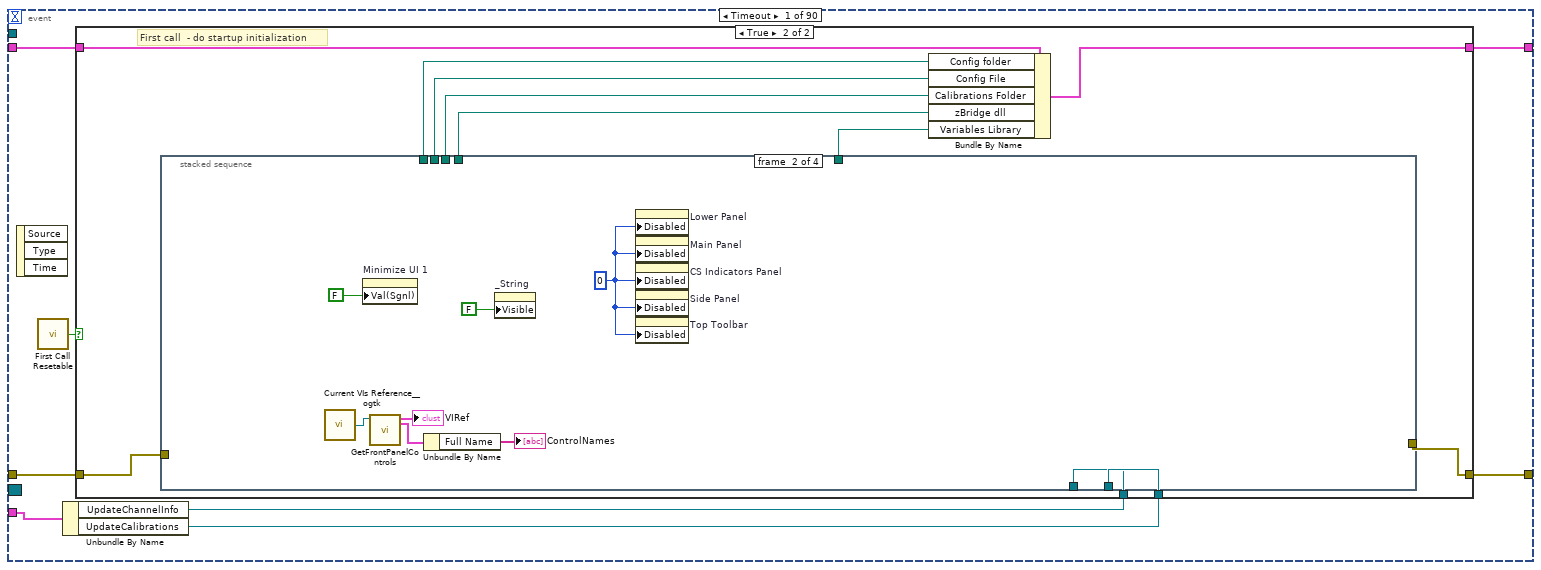
[diagram p15: hidden frame]
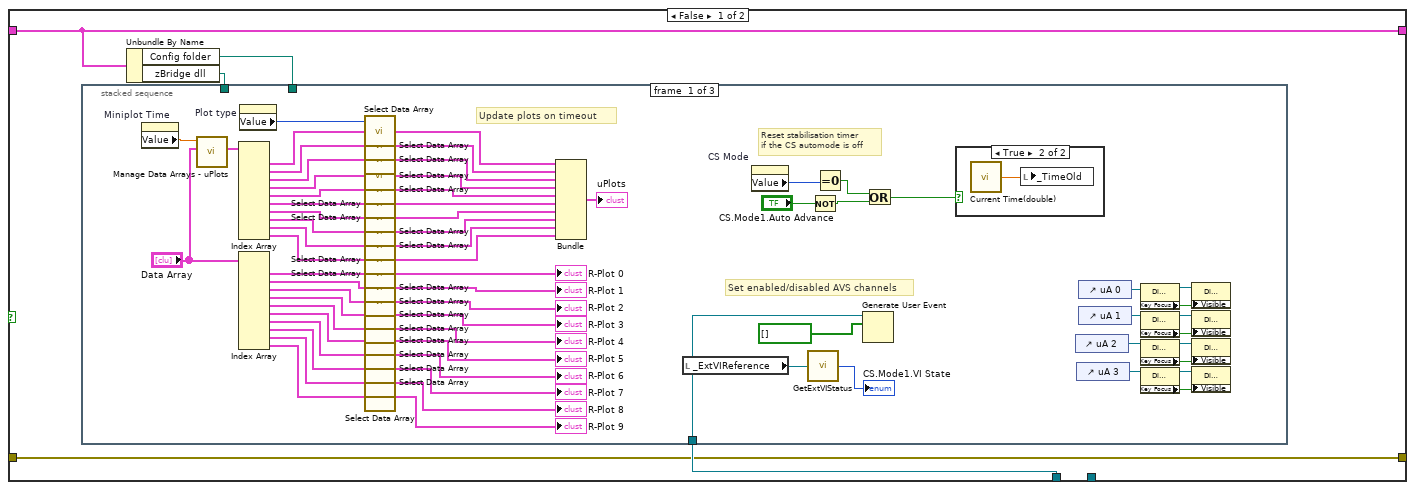
[diagram p16: hidden frame]
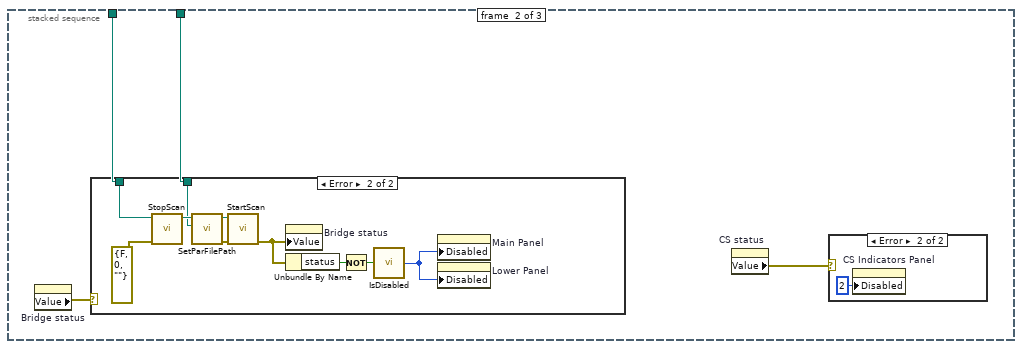
[diagram p18: hidden frame]
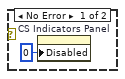
[diagram p19: hidden frame]
diagram:
  w30 = path ""  # Variables Library
  w31 = path ""  # zBridge dll
  w32 = path ""  # Calibrations Folder
  w33 = path ""  # Config File
  w35 = path ""  # Config folder
  (unwired) path "C:/LC Data/Configuration" ("Relative path (.)")
  w38 = dbl[] [1.0]  # Data Array
  w52 = "CallExtVI"  # CallExtVI
  w53 = bool[] []  # UpdateChannelInfo
  w54 = cluster{"Time":dbl, "R":dbl[], "T":dbl[]} {"Time"=1.0, "R"=[1.0], "T"=[1.0]}  # CS Automode
  w55 = cluster{"R":dbl[], "T":dbl[]} {"R"=[1.0], "T"=[1.0]}  # UpdateValuesAVS
  w56 = cluster{"R":dbl[], "T":dbl[]} {"R"=[1.0], "T"=[1.0]}  # UpdateValuesZBridge
  w57 = "ResetPIDloop"  # Reset PID loop
  w58 = TRUE  # TempStabilized
  w59 = "UpdateLogFilePath"  # UpdateLogFilePath
  w60 = "UpdateCalibrations"  # UpdateCalibrations
  # "Unwired (but used) controls"
  n1 = control-ref of="R"() -> (w29:refnum<vi>)
  n2 = control-ref of="T"() -> (w28:refnum<vi>)
  n3 = control-ref of="Small R Cluster"() -> (w4:refnum<vi>)
  n4 = control-ref of="Small T Cluster"() -> (w3:refnum<vi>)
  n5 = Create User Event(user event datatype=w53) -> (user event=w50:refnum<user-event>)  [unwired: 1 in, 1 out]
  n6 = Create User Event(user event datatype=w55) -> (user event=w49:refnum<user-event>)  [unwired: 1 in, 1 out]
  n7 = Create User Event(user event datatype=w60) -> (user event=w48:refnum<user-event>)  [unwired: 1 in, 1 out]
  n8 = Create User Event(user event datatype=w59) -> (user event=w47:refnum<user-event>)  [unwired: 1 in, 1 out]
  n9 = Create User Event ("TempStabilized")(user event datatype=w58) -> (user event=w46:refnum<user-event>)  [unwired: 1 in, 1 out]
  n10 = Create User Event(user event datatype=w57) -> (user event=w45:refnum<user-event>)  [unwired: 1 in, 1 out]
  n11 = Create User Event(user event datatype=w56) -> (user event=w44:refnum<user-event>)  [unwired: 1 in, 1 out]
  n12 = Create User Event(user event datatype=w54) -> (user event=w43:refnum<user-event>)  [unwired: 1 in, 1 out]
  n13 = Create User Event(user event datatype=w52) -> (user event=w42:refnum<user-event>)  [unwired: 1 in, 1 out]
  n14 = Create User Event(user event datatype=w38) -> (user event=w39:refnum<user-event>)  [unwired: 1 in, 1 out]
  n15 = property class="Clust (strict)"(reference=w29) -> ("Controls[]"=w7:refnum<vi>[])  [unwired: 1 in, 2 out]
  n16 = property class="Clust (strict)"(reference=w28) -> ("Controls[]"=w6:refnum<vi>[])  [unwired: 1 in, 2 out]
  n17 = property class="Clust (strict)"(reference=w4) -> ("Controls[]"=w2:refnum<vi>[])  [unwired: 1 in, 2 out]
  n18 = property class="Clust (strict)"(reference=w3) -> ("Controls[]"=w1:refnum<vi>[])  [unwired: 1 in, 2 out]
  n19 = Generate Occurrence() -> (w37:refnum<k4>)
  n20 = control-ref of="R8"() -> (w27:refnum<vi>)
  n21 = control-ref of="R9"() -> (w26:refnum<vi>)
  n22 = control-ref of="R7"() -> (w25:refnum<vi>)
  n23 = control-ref of="R6"() -> (w24:refnum<vi>)
  n24 = control-ref of="R5"() -> (w23:refnum<vi>)
  n25 = control-ref of="R4"() -> (w22:refnum<vi>)
  n26 = control-ref of="R3"() -> (w21:refnum<vi>)
  n27 = control-ref of="R2"() -> (w20:refnum<vi>)
  n28 = control-ref of="R1"() -> (w19:refnum<vi>)
  n29 = control-ref of="R0"() -> (w18:refnum<vi>)
  n30 = control-ref of="T9"() -> (w17:refnum<vi>)
  n31 = control-ref of="T8"() -> (w16:refnum<vi>)
  n32 = control-ref of="T7"() -> (w15:refnum<vi>)
  n33 = control-ref of="T6"() -> (w14:refnum<vi>)
  n34 = control-ref of="T5"() -> (w13:refnum<vi>)
  n35 = control-ref of="T4"() -> (w12:refnum<vi>)
  n36 = control-ref of="T3"() -> (w11:refnum<vi>)
  n37 = control-ref of="T2"() -> (w10:refnum<vi>)
  n38 = control-ref of="T1"() -> (w9:refnum<vi>)
  n39 = control-ref of="T0"() -> (w8:refnum<vi>)
  n40 = flat-sequence {
    tunnel: w37 -> [w61]
    tunnel: [w61] -> w36
    frame #0 {
      # "Check if the QCS needs the registry patch and run the patching utility"
      n41 = disable-structure shown="Enabled" {
        frame Enabled {
          n42 = call "QCS - Check Registry.vi"() -> ("QCS needs reset?"=w62:bool)  [unwired: 5 in]
          n43 = case shown="True" w62 {
            frame False {
            }
            frame True {
              n44 = call "QCS - Locate Registry Patcher.vi"() -> ("dup path"=w64:path)  [unwired: 5 in]
              n45 = Path To String(path=w64) -> (string=w65:string)
              n46 = call <vilib>:"System Exec.vi"("wait until completion? (T)"=TRUE, "command line"=w65) -> ()  [unwired: 6 in, 4 out]
            }
          }
        }
        frame Disabled {
        }
      }
    }
  }
  n47 = Build Array (concatenate)(w27, w26, w25, w24, w23, w22, w21, w20, w19, w18, w17, w16, w15, w14, w13, w12, w11, w10, w9, w8, w7, w6, w2, w1) -> (w5:refnum<vi>[])
  n48 = Bundle("UpdateChannelInfo"=w50, "UpdateValuesAVS"=w49, "UpdateCalibrations"=w48, "UpdateLogFilePath"=w47, "TempStabilized"=w46, "Reset PID loop"=w45, "UpdateValuesZBridge"=w44, "CS Automode"=w43, "CallExtVI"=w42, "Data Array"=w39) -> (w41:T49)  [unwired: 1 in]
  n49 = register-events(w41, w5) -> (reference out=w51:refnum<event-registration>)  [unwired: 2 in, 1 out]
  n50 = Bundle("Config folder"=w35, "Config File"=w33, "Calibrations Folder"=w32, "zBridge dll"=w31, "Variables Library"=w30) -> (w34:T50)  [unwired: 1 in]
  n51 = call "MGI Clear Error.vi"() -> ("Error Out"=w40:errorcluster)  [unwired: 7 in]
  n52 = while {
    tunnel: w51 -> [w73]
    shift-right: [w70] -> _
    shift-left: w40 -> [w71]
    tunnel: w41 -> [w69]
    tunnel: w36 -> [w68]
    shift-right: [w66] -> _
    shift-left: w34 -> [w67]
    stop <- FALSE stop-if-true
    # "Event handling loop"
    n53 = event shown="[4] <#1.UpdateValuesAVS>: User Event" {
      selector: w73 -> [_ _ _ _ _ _ _ _ _ _ _ _ _ _ _ _ _ _ _ _ _ _ _ _ _ _ _ _ _ _ _ _ _ _ _ _ _ _ _ _ _ _ _ _ _ _ _ _ _ _ _ _ _ _ _ _ _ _ _ _ _ _ _ _ _ _ _ _ _ _ _ _ _ _ _ _ _ _ _ _ _ _ _ _ _ _ _ _ _ _]
      dyn-events: _ -> [_ _ _ _ _ _ _ _ _ _ _ _ _ _ _ _ _ _ _ _ _ _ _ _ _ _ _ _ _ _ _ _ _ _ _ _ _ _ _ _ _ _ _ _ _ _ _ _ _ _ _ _ _ _ _ _ _ _ _ _ _ _ _ _ _ _ _ _ _ _ _ _ _ _ _ _ _ _ _ _ _ _ _ _ _ _ _ _ _ _]
      timeout: 200 -> [_ _ _ _ _ _ _ _ _ _ _ _ _ _ _ _ _ _ _ _ _ _ _ _ _ _ _ _ _ _ _ _ _ _ _ _ _ _ _ _ _ _ _ _ _ _ _ _ _ _ _ _ _ _ _ _ _ _ _ _ _ _ _ _ _ _ _ _ _ _ _ _ _ _ _ _ _ _ _ _ _ _ _ _ _ _ _ _ _ _]
      tunnel: w71 -> [w82 _ _ w525 w573 w666 _ _ w886 _ _ _ w1015 w1024 _ _ _ _ _ _ _ _ _ w1273 _ w1282 _ _ _ _ _ _ _ _ w1387 _ _ _ _ _ _ _ _ _ _ _ _ _ _ _ _ _ _ _ _ _ _ w1813 w1833 _ _ _ _ _ w1978 _ _ _ _ _ _ _ _ _ _ _ _ _ _ _ _ _ _ _ _ _ _ _ _ _]
      tunnel: [w81 _ _ w528 w572 w661 _ _ w884 _ _ _ w1014 w1024 _ _ _ _ _ _ _ _ _ w1273 _ w1282 _ _ _ _ _ _ w1369 _ w1387 _ _ _ _ _ _ _ _ _ _ _ _ _ _ _ _ _ _ _ _ _ _ w1812 w1832 _ _ _ _ _ w1978 _ _ _ _ _ _ _ _ _ _ _ _ _ _ _ _ _ _ _ _ _ _ _ _ _] -> w70
      tunnel: w69 -> [w79 _ _ w510 w568 w663 w776 w865 _ _ _ _ _ _ _ _ _ _ _ _ _ _ _ _ _ _ w1313 w1335 _ _ _ _ _ w1377 w1385 _ _ _ _ _ _ _ _ _ _ _ _ _ _ _ _ _ _ _ _ _ _ _ w1827 _ w1908 w1922 _ _ _ _ _ w1984 _ _ w2006 w2023 w2027 _ _ _ _ _ _ _ _ _ _ w2107 _ _ _ _ _ _]
      tunnel: w68 -> [_ w343 _ _ _ _ _ _ _ _ _ _ _ _ _ _ _ _ _ _ _ _ _ _ _ _ _ _ _ _ _ _ _ _ _ _ _ _ _ _ _ _ _ _ _ _ _ _ _ _ _ _ _ _ _ _ _ _ _ _ _ _ _ _ _ _ _ _ _ _ _ _ _ _ _ _ _ _ _ _ _ _ _ _ _ _ _ _ _ _]
      tunnel: w67 -> [w75 w342 w474 w506 w566 w660 w772 w863 w883 w920 w977 w1005 w1012 w1020 w1063 w1080 w1146 w1159 w1199 w1201 w1204 w1217 w1260 w1268 w1276 w1280 w1311 w1333 w1337 w1340 w1348 w1357 w1367 w1375 w1380 w1407 w1411 w1486 w1493 w1500 w1542 w1570 w1604 w1631 w1637 w1645 w1653 w1662 w1671 w1673 w1718 w1726 w1731 w1754 w1771 w1796 w1800 w1804 w1825 w1896 w1906 w1920 w1930 w1955 w1977 w1979 w1980 w1982 w1988 w1992 w2003 w2021 w2025 w2038 w2045 w2046 w2054 w2057 w2061 w2065 w2068 w2094 w2100 w2105 w2109 w2113 w2134 w2146 w2156 w2158]
      tunnel: [w76 w342 w474 w506 w566 w660 w772 w863 w883 w920 w977 w1005 w1011 w1020 w1063 w1080 w1146 w1159 w1199 w1201 w1204 w1217 w1260 w1268 w1276 w1280 w1311 w1333 w1337 w1340 w1348 w1357 w1367 w1375 w1380 w1407 w1411 w1486 w1493 w1500 w1542 w1570 w1604 w1631 w1637 w1645 w1653 w1662 w1671 w1673 w1718 w1726 w1731 w1754 w1771 w1796 w1800 w1804 w1825 w1896 w1906 w1920 w1930 w1955 w1977 w1979 w1980 w1982 w1988 w1992 w2003 w2021 w2025 w2038 w2045 w2046 w2054 w2057 w2061 w2065 w2068 w2094 w2100 w2105 w2109 w2113 w2134 w2146 w2156 w2158] -> w66
      event Timeout {
        n54 = event-data() -> ()  [unwired: 1 in, 3 out]
        n55 = call "First Call Resetable.vi"() -> ("First Call?"=w80:bool)
        n56 = Unbundle By Name(w79) -> ("UpdateChannelInfo"=w77:refnum<user-event>, "UpdateCalibrations"=w78:refnum<user-event>)
        n57 = case shown="True" w80 {
          tunnel: w82 -> [w86 w211]
          tunnel: [w86 w209] -> w81
          tunnel: w78 -> [_ w210]
          tunnel: w77 -> [w87 w208]
          tunnel: w75 -> [w85 w207]
          tunnel: [w85 w206] -> w76
          frame False {
            n58 = Unbundle By Name(w85) -> ("Config folder"=w84:path, "zBridge dll"=w83:path)
            n59 = stacked-sequence {
              tunnel: w87 -> [w88 _ _]
              tunnel: w84 -> [_ w156 _]
              tunnel: w83 -> [_ w155 _]
              frame #0 {
                # "Update plots on timeout"
                # "Set enabled/disabled AVS channels"
                # "Reset stabilisation timer\nif the CS automode is off"
                n60 = property on="Miniplot Time" class="DigNum (strict)"() -> ("Value"=w149:dbl)  [unwired: 2 in, 2 out]
                n61 = call "Manage Data Arrays - uPlots.vi"("Data In"="Data Array", "Data Memory"=w149) -> ("Data Out"=w104:T28)  [unwired: 7 in]
                n62 = Index Array(array=w104) -> (element #1=w119:cluster{"R":dbl[], "T":dbl[], "Time":dbl[]}, element #2=w120:cluster{"R":dbl[], "T":dbl[], "Time":dbl[]}, element #3=w121:cluster{"R":dbl[], "T":dbl[], "Time":dbl[]}, element #4=w122:cluster{"R":dbl[], "T":dbl[], "Time":dbl[]}, element #5=w123:cluster{"R":dbl[], "T":dbl[], "Time":dbl[]}, element #6=w124:cluster{"R":dbl[], "T":dbl[], "Time":dbl[]}, element #7=w125:cluster{"R":dbl[], "T":dbl[], "Time":dbl[]}, element #8=w126:cluster{"R":dbl[], "T":dbl[], "Time":dbl[]}, element #9=w127:cluster{"R":dbl[], "T":dbl[], "Time":dbl[]}, element #10=w128:cluster{"R":dbl[], "T":dbl[], "Time":dbl[]})  [unwired: 10 in]
                n63 = Index Array(array="Data Array") -> (element #1=w148:cluster{"R":dbl[], "T":dbl[], "Time":dbl[]}, element #2=w147:cluster{"R":dbl[], "T":dbl[], "Time":dbl[]}, element #3=w146:cluster{"R":dbl[], "T":dbl[], "Time":dbl[]}, element #4=w145:cluster{"R":dbl[], "T":dbl[], "Time":dbl[]}, element #5=w144:cluster{"R":dbl[], "T":dbl[], "Time":dbl[]}, element #6=w143:cluster{"R":dbl[], "T":dbl[], "Time":dbl[]}, element #7=w142:cluster{"R":dbl[], "T":dbl[], "Time":dbl[]}, element #8=w141:cluster{"R":dbl[], "T":dbl[], "Time":dbl[]}, element #9=w140:cluster{"R":dbl[], "T":dbl[], "Time":dbl[]}, element #10=w139:cluster{"R":dbl[], "T":dbl[], "Time":dbl[]})  [unwired: 10 in]
                n64 = property on="Plot type" class="Enum (strict)"() -> ("Value"=w107:enum16{"R vs Time", "T vs Time"})  [unwired: 2 in, 2 out]
                n65 = call "Select Data Array.vi"("Cluster 2"=w119, "Value"=w107) -> ("Cluster"=w129:cluster{"Time":dbl[], "T":dbl[]})
                n66 = call "Select Data Array.vi"("Cluster 2"=w120, "Value"=w107) -> ("Cluster"=w130:cluster{"Time":dbl[], "T":dbl[]})
                n67 = call "Select Data Array.vi"("Cluster 2"=w121, "Value"=w107) -> ("Cluster"=w131:cluster{"Time":dbl[], "T":dbl[]})
                n68 = call "Select Data Array.vi"("Cluster 2"=w122, "Value"=w107) -> ("Cluster"=w132:cluster{"Time":dbl[], "T":dbl[]})
                n69 = call "Select Data Array.vi"("Cluster 2"=w123, "Value"=w107) -> ("Cluster"=w138:cluster{"Time":dbl[], "T":dbl[]})
                n70 = call "Select Data Array.vi"("Cluster 2"=w124, "Value"=w107) -> ("Cluster"=w133:cluster{"Time":dbl[], "T":dbl[]})
                n71 = call "Select Data Array.vi"("Cluster 2"=w125, "Value"=w107) -> ("Cluster"=w134:cluster{"Time":dbl[], "T":dbl[]})
                n72 = call "Select Data Array.vi"("Cluster 2"=w126, "Value"=w107) -> ("Cluster"=w135:cluster{"Time":dbl[], "T":dbl[]})
                n73 = call "Select Data Array.vi"("Cluster 2"=w127, "Value"=w107) -> ("Cluster"=w136:cluster{"Time":dbl[], "T":dbl[]})
                n74 = call "Select Data Array.vi"("Cluster 2"=w128, "Value"=w107) -> ("Cluster"=w137:cluster{"Time":dbl[], "T":dbl[]})
                n75 = call "Select Data Array.vi"("Cluster 2"=w148, "Value"=w107) -> ("Cluster"=→"R-Plot 0":cluster{"Time":dbl[], "T":dbl[]})
                n76 = call "Select Data Array.vi"("Cluster 2"=w147, "Value"=w107) -> ("Cluster"=→"R-Plot 1":cluster{"Time":dbl[], "T":dbl[]})
                n77 = call "Select Data Array.vi"("Cluster 2"=w146, "Value"=w107) -> ("Cluster"=→"R-Plot 2":cluster{"Time":dbl[], "T":dbl[]})
                n78 = call "Select Data Array.vi"("Cluster 2"=w145, "Value"=w107) -> ("Cluster"=→"R-Plot 3":cluster{"Time":dbl[], "T":dbl[]})
                n79 = call "Select Data Array.vi"("Cluster 2"=w144, "Value"=w107) -> ("Cluster"=→"R-Plot 4":cluster{"Time":dbl[], "T":dbl[]})
                n80 = call "Select Data Array.vi"("Cluster 2"=w143, "Value"=w107) -> ("Cluster"=→"R-Plot 5":cluster{"Time":dbl[], "T":dbl[]})
                n81 = call "Select Data Array.vi"("Cluster 2"=w142, "Value"=w107) -> ("Cluster"=→"R-Plot 6":cluster{"Time":dbl[], "T":dbl[]})
                n82 = call "Select Data Array.vi"("Cluster 2"=w141, "Value"=w107) -> ("Cluster"=→"R-Plot 7":cluster{"Time":dbl[], "T":dbl[]})
                n83 = call "Select Data Array.vi"("Cluster 2"=w140, "Value"=w107) -> ("Cluster"=→"R-Plot 8":cluster{"Time":dbl[], "T":dbl[]})
                n84 = call "Select Data Array.vi"("Cluster 2"=w139, "Value"=w107) -> ("Cluster"=→"R-Plot 9":cluster{"Time":dbl[], "T":dbl[]})
                n85 = Bundle("Cluster"=w129, "Cluster"=w130, "Cluster"=w131, "Cluster"=w132, "Cluster"=w138, "Cluster"=w133, "Cluster"=w134, "Cluster"=w135, "Cluster"=w136, "Cluster"=w137) -> (→"uPlots":T59)  [unwired: 1 in]
                n86 = local read "_ExtVIReference"() -> (w103:refnum<vi>)
                n87 = property on="CS Mode" class="Enum (strict)"() -> ("Value"=w152:T39)  [unwired: 2 in, 2 out]
                n88 = call "GetExtVIStatus.vi"("vi reference in"=w103) -> ("Exec.State"=→"CS.Mode1.VI State":T46)  [unwired: 2 out]
                n89 = Not(x="CS.Mode1.Auto Advance") -> (.not. x?=w151:bool)
                n90 = Equal To 0?(x=w152) -> (x = 0?=w101:bool)
                n91 = Generate User Event(user event=w88, event data cluster=bool[] [] ("event data")) -> ()  [unwired: 2 in, 2 out]
                n92 = Or(x=w101, y=w151) -> (x .or. y?=w150:bool)
                n93 = case shown="True" w150 {
                  frame False {
                  }
                  frame True {
                    n94 = call "Current Time(double).vi"() -> ("Current Time (double)"=w154:dbl)  [unwired: 6 in, 1 out]
                    n95 = local write "_TimeOld"(w154) -> ()
                  }
                }
                n96 = control-ref of="uA 2"() -> (w89:refnum<vi>)
                n97 = control-ref of="uA 3"() -> (w90:refnum<vi>)
                n98 = control-ref of="uA 0"() -> (w100:refnum<vi>)
                n99 = control-ref of="uA 1"() -> (w96:refnum<vi>)
                n100 = property class="DigNum (strict)"(reference=w100) -> (reference out=w99:refnum<vi>, "Key Focus"=w98:bool)  [unwired: 1 in, 1 out]
                n101 = property class="DigNum (strict)"(reference=w96) -> (reference out=w97:refnum<vi>, "Key Focus"=w95:bool)  [unwired: 1 in, 1 out]
                n102 = property class="DigNum (strict)"(reference=w89) -> (reference out=w91:refnum<vi>, "Key Focus"=w92:bool)  [unwired: 1 in, 1 out]
                n103 = property class="DigNum (strict)"(reference=w90) -> (reference out=w93:refnum<vi>, "Key Focus"=w94:bool)  [unwired: 1 in, 1 out]
                n104 = property class="DigNum (strict)"(reference=w99, "Visible"=w98) -> ()  [unwired: 1 in, 2 out]
                n105 = property class="DigNum (strict)"(reference=w97, "Visible"=w95) -> ()  [unwired: 1 in, 2 out]
                n106 = property class="DigNum (strict)"(reference=w91, "Visible"=w92) -> ()  [unwired: 1 in, 2 out]
                n107 = property class="DigNum (strict)"(reference=w93, "Visible"=w94) -> ()  [unwired: 1 in, 2 out]
              }
              frame #1 {
                n108 = property on="Bridge status" class="Clust (strict)"() -> ("Value"=w158:errorcluster)  [unwired: 2 in, 2 out]
                n109 = case shown="Error" w158 {
                  tunnel: w156 -> [_ w162]
                  tunnel: w155 -> [_ w161]
                  frame No Error {
                  }
                  frame Error {
                    n110 = call "StopScan.vi"("error in (no error)"=errorcluster {"status"=FALSE, "code"=0, "source"=""}, "path in"=w161) -> ("path out"=w168:path)  [unwired: 8 in, 1 out]
                    n111 = call "SetParFilePath.vi"("path"=w162, "zDll"=w168) -> ("error out"=w170:errorcluster, "zDll out"=w169:path)  [unwired: 8 in]
                    n112 = call "StartScan.vi"("error in (no error)"=w170, "path in"=w169) -> ("error out"=w166:errorcluster)  [unwired: 8 in, 1 out]
                    n113 = property on="Bridge status" class="Clust (strict)"("Value"=w166) -> ()  [unwired: 2 in, 2 out]
                    n114 = Unbundle By Name(w166) -> ("status"=w164:bool)
                    n115 = Not(x=w164) -> (.not. x?=w165:bool)
                    n116 = call "IsDisabled.vi"("Enabled?"=w165) -> ("Numeric"=w163:i16)
                    n117 = property on="Main Panel" class="TabCtl (strict)"("Disabled"=w163) -> ()  [unwired: 2 in, 2 out]
                    n118 = property on="Lower Panel" class="TabCtl (strict)"("Disabled"=w163) -> ()  [unwired: 2 in, 2 out]
                  }
                }
                n119 = property on="CS status" class="Clust (strict)"() -> ("Value"=w157:errorcluster)  [unwired: 2 in, 2 out]
                n120 = case shown="Error" w157 {
                  frame No Error {
                    n121 = property on="CS Indicators Panel" class="TabCtl (strict)"("Disabled"=u8 0) -> ()  [unwired: 2 in, 2 out]
                  }
                  frame Error {
                    n122 = property on="CS Indicators Panel" class="TabCtl (strict)"("Disabled"=u8 2) -> ()  [unwired: 2 in, 2 out]
                  }
                }
              }
              frame #2 {
                # "Check if the structure is \nnot empty and only one\nof Scalar or Array is set"
                # "Set FP control value from external script/program"
                n123 = local read "_SetControl"() -> (w171:T1)
                n124 = Unbundle By Name(w171) -> ("Name"=w173:string, "Scalar"=w172:string, "Array"=w181:string[][])
                n125 = call "Empty 2D Array (String)__ogtk.vi"("Array"=w181) -> ("Empty Array?"=w178:bool)  [unwired: 8 in]
                n126 = Empty String/Path?(string/path=w173) -> (empty?=w177:bool)
                n127 = Empty String/Path?(string/path=w172) -> (empty?=w176:bool)
                n128 = Not(x=w177) -> (.not. x?=w175:bool)
                n129 = Not(x=w176) -> (.not. x?=w179:bool)
                n130 = Not(x=w178) -> (.not. x?=w182:bool)
                n131 = Exclusive Or(1:w182, 2:w179) -> (0:w180:bool)
                n132 = And(x=w175, y=w180) -> (x .and. y?=w174:bool)
                n133 = case shown="True" w174 {
                  tunnel: w173 -> [_ w186]
                  tunnel: w172 -> [_ w185]
                  tunnel: w181 -> [_ w184]
                  tunnel: w182 -> [_ w183]
                  frame False {
                  }
                  frame True {
                    n134 = flat-sequence {
                      tunnel: w186 -> [w190]
                      tunnel: w185 -> [w189]
                      tunnel: w184 -> [w187]
                      tunnel: w183 -> [w188]
                      frame #0 {
                        n135 = local read "VIRef"() -> (w191:T2)
                        n136 = case shown="False" w188 {
                          tunnel: w191 -> [w194 w197]
                          tunnel: w190 -> [w193 w196]
                          tunnel: w189 -> [w192 _]
                          tunnel: w187 -> [_ w195]
                          frame False {
                            n137 = call "Push2VI.vi"("New Value"=w192, "element"=w193, "VIRef"=w194) -> ()  [unwired: 8 in, 1 out]
                          }
                          frame True {
                            n138 = call "PushArray2VI.vi"("Str"=w195, "element"=w196, "VIRef"=w197) -> ()  [unwired: 8 in, 1 out]
                          }
                        }
                      }
                      frame #1 {
                        w199 = ""
                        n139 = Bundle(w199, w199, "Array"=string[][] []) -> (→"_SetControl":cluster{string, string, "Array":string[][]})  [unwired: 1 in]
                      }
                    }
                  }
                }
              }
            }
          }
          frame True {
            # "First call  - do startup initialization"
            n140 = stacked-sequence {
              tunnel: w211 -> [_ _ w256 _]
              tunnel: [_ _ w250 _] -> w209
              tunnel: w210 -> [_ _ w252 _]
              tunnel: w208 -> [_ _ _ w310]
              tunnel: [_ _ w248 _] -> w205
              tunnel: [_ _ w249 _] -> w204
              tunnel: [_ _ w247 _] -> w203
              tunnel: [_ _ w245 _] -> w202
              tunnel: [w212 _ _ _] -> w201
              frame #0 {
                # "Set control bindings"
                # "\\\\localhost\\DR TempControl\\Currents(In)"
                # "\\\\localhost\\DR TempControl\\Temperatures"
                # "\\\\localhost\\DR TempControl\\Resistances"
                # "\\\\localhost\\DR TempControl\\Currents(Out)"
                n141 = disable-structure shown="RUN_TIME_ENGINE==True" {
                  disable-tunnel: [w225 "\\\\localhost\\DR TempControl\\"] -> w213
                  disable-tunnel: [w222 w235] -> w212
                  frame condition #0 {
                    w232 = u16 0 items=["overwrite", "ask first", "don't overwrite"] ("overwrite")
                    # "Deploy the shared variable library. If there are few copies of the program\nrunning - generate unique name for every copy."
                    n142 = call "Enum Variables.vi"("regular expression"="DR TempControl.*") -> ("Containers"=w230:string[])  [unwired: 15 in, 3 out]
                    n143 = call "Generate New Name.vi"("Existing names"=w230, "Base Name"="DR TempControl") -> ("New Name (path)"=w227:path, "New Name"=w226:string)  [unwired: 16 in]
                    n144 = call "Temporary Directory__ogtk.vi"("Relative path (.)"=w227) -> ("Temporary Directory (+ Relative)"=w231:path)
                    n145 = call "Current VIs Parent Directory__ogtk.vi"("Relative path (.)"=path "DR TempControl.lvlib" ("Library Path")) -> ("Parent Directory (+ Relative)"=w233:path)  [unwired: 4 in]
                    n146 = call <vilib>:"Librarian Copy.vi"("source"=w233, "overwrite"=w232, "destination"=w231) -> ("dup destination"=w222:path)  [unwired: 7 in, 1 out]
                    n147 = invoke class="App" method="Library.Deploy Library"("libPath"=w222) -> ()  [unwired: 4 in, 5 out]
                    n148 = Concatenate Strings("\\\\localhost\\" ("string"), w226, "\\" ("string")) -> (w225:string)
                  }
                  frame condition #1 (active) {
                    # "Default library is deployed automatically in development environment"
                    n149 = call "Current VIs Parent Directory__ogtk.vi"("Relative path (.)"=path "DR TempControl.lvlib" ("Library Path")) -> ("Parent Directory (+ Relative)"=w235:path)  [unwired: 4 in]
                  }
                }
                n150 = Concatenate Strings(w213, "Resistances" ("string")) -> (w219:string)
                n151 = Concatenate Strings(w213, "Temperatures" ("string")) -> (w216:string)
                n152 = Concatenate Strings(w213, "Currents(Out)" ("string")) -> (w215:string)
                n153 = Concatenate Strings(w213, "Currents(In)" ("string")) -> (w214:string)
                n154 = property on="R Array" class="Arr (strict)"("FPB.URL"=w219) -> ()  [unwired: 2 in, 2 out]
                n155 = property on="T Array" class="Arr (strict)"("FPB.URL"=w216) -> ()  [unwired: 2 in, 2 out]
                n156 = property on="CS.Actual Current" class="Arr (strict)"("FPB.URL"=w215) -> ()  [unwired: 2 in, 2 out]
                n157 = property on="CS.Automode Current" class="Arr (strict)"("FPB.URL"=w214) -> ()  [unwired: 2 in, 2 out]
              }
              frame #1 {
                w243 = u8 0 ("Disabled")
                n158 = call "Current VIs Reference__ogtk.vi"() -> ("Current VI's reference"=w241:refnum<vi>)  [unwired: 5 in]
                n159 = property on="Minimize UI 1" class="Bool (strict)"("Val(Sgnl)"=FALSE ("Value (Signaling)")) -> ()  [unwired: 2 in, 2 out]
                n160 = call "GetFrontPanelControls.vi"("Ref to VI"=w241) -> ("VIRef"=w240:T2)  [unwired: 9 in, 1 out]
                "VIRef" <- w240
                n161 = Unbundle By Name(w240) -> ("Full Name"=→"ControlNames":string[])
                n162 = property on="_String" class="Str"("Visible"=FALSE) -> ()  [unwired: 2 in, 2 out]
                n163 = property on="Lower Panel" class="TabCtl (strict)"("Disabled"=w243) -> ()  [unwired: 2 in, 2 out]
                n164 = property on="Main Panel" class="TabCtl (strict)"("Disabled"=w243) -> ()  [unwired: 2 in, 2 out]
                n165 = property on="CS Indicators Panel" class="TabCtl (strict)"("Disabled"=w243) -> ()  [unwired: 2 in, 2 out]
                n166 = property on="Side Panel" class="TabCtl (strict)"("Disabled"=w243) -> ()  [unwired: 2 in, 2 out]
                n167 = property on="Top Toolbar" class="TabCtl (strict)"("Disabled"=w243) -> ()  [unwired: 2 in, 2 out]
              }
              frame #2 {
                # "Read settings from the config file"
                n168 = flat-sequence {
                  tunnel: w256 -> [w257]
                  tunnel: [w257] -> w251
                  tunnel: [w260] -> w249
                  tunnel: [w261] -> w248
                  tunnel: [w262] -> w247
                  tunnel: [w261] -> w246
                  tunnel: [w258] -> w245
                  tunnel: [w277] -> w255
                  tunnel: w251 -> [w276]
                  tunnel: w246 -> [w278]
                  tunnel: w255 -> [w288]
                  tunnel: [w288] -> w254
                  tunnel: [w292] -> w253
                  tunnel: w254 -> [w289]
                  tunnel: w253 -> [w297]
                  tunnel: [w297] -> w244
                  tunnel: [w301] -> w250
                  tunnel: w252 -> [w298]
                  tunnel: w244 -> [w299]
                  frame #0 {
                    w263 = path "C:/LC Data" ("LC Data")
                    n169 = call "Generate config file path.vi"("LC data path"=w263) -> ("Config folder"=w262:path)  [unwired: 18 in]
                    n170 = call "Build Path - Traditional__ogtk.vi"("name or relative path"="config.ini", "base path"=w262) -> ("appended path"=w261:path)
                    n171 = call "Build Path - Traditional__ogtk.vi"("name or relative path"="Calibrations", "base path"=w263) -> ("appended path"=w260:path)
                    n172 = property on="Calibrations Folder" class="Path"("Value"=w260) -> ()  [unwired: 2 in, 2 out]
                    n173 = call "Current VIs Parent Directory__ogtk.vi"("Relative path (.)"=path "data/ImpBridgeDll.dll" ("Library Path")) -> ("Parent Directory (+ Relative)"=w258:path)  [unwired: 4 in]
                    "_zBridgeDll" <- w258
                  }
                  frame #1 {
                    n174 = control-ref of="zBridge.Active Channels"() -> (w275:refnum<vi>)
                    n175 = control-ref of="CS Settings"() -> (w274:refnum<vi>)
                    n176 = control-ref of="Bridge settings"() -> (w273:refnum<vi>)
                    n177 = control-ref of="Runtime Settings"() -> (w272:refnum<vi>)
                    n178 = control-ref of="Data Logging Settings"() -> (w271:refnum<vi>)
                    n179 = control-ref of="PID setup"() -> (w270:refnum<vi>)
                    n180 = control-ref of="CS Cannel Names"() -> (w284:refnum<vi>)
                    n181 = control-ref of="AVS names"() -> (w266:refnum<vi>)
                    n182 = control-ref of="_CurCalibrations"() -> (w267:refnum<vi>)
                    n183 = control-ref of="CS.Mode1.PID"() -> (w268:refnum<vi>)
                    n184 = control-ref of="CS.Mode1.Settings"() -> (w269:refnum<vi>)
                    n185 = call "Current VIs Parent Directory__ogtk.vi"("Relative path (.)"=path "data/config.ini") -> ("Parent Directory (+ Relative)"=w281:path)  [unwired: 4 in]
                    n186 = Build Array(w275, w274, w273, w272, w271, w270, w284, w266, w267, w268, w269) -> (w280:refnum<vi>[])
                    n187 = call "Save Load Settings to File by Ref with path.vi"("Array of Cluster References"=w280, "Action"=enum8{"Load", "Save"}."Load", "error in (no error)"=w276, "Configuration file"=w281) -> ("error out"=w283:errorcluster)  [unwired: 5 in]
                    n188 = call "MGI Clear Error.vi"("Error In"=w283) -> ("Error Out"=w282:errorcluster)  [unwired: 6 in]
                    n189 = call "Save Load Settings to File by Ref with path.vi"("Array of Cluster References"=w280, "Action"=enum8{"Load", "Save"}."Load", "error in (no error)"=w282, "Configuration file"=w278) -> ("error out"=w277:errorcluster)  [unwired: 5 in]
                  }
                  frame #2 {
                    n190 = Wait (ms)(milliseconds to wait=250) -> ()  [unwired: 1 out]
                  }
                  frame #3 {
                    n191 = control-ref of="Sensor Calibrations"() -> (w291:refnum<vi>)
                    n192 = control-ref of="_CurCalibrations"() -> (w290:refnum<vi>)
                    n193 = control-ref of="Calibrations Folder"() -> (w294:refnum<vi>)
                    n194 = control-ref of="_QuickConvertCal"() -> (w293:refnum<vi>)
                    n195 = control-ref of="Sensor 1"() -> (w295:refnum<vi>)
                    n196 = call "ReloadCalibrations.vi"("error in (no error)"=w289, "Quick convert sensors"=w293, "CurCalibrations"=w290, "Calibration files path"=w294, "Channel1 sensors"=w295, "Channels list"=w291) -> ("error out"=w292:errorcluster)  [unwired: 1 in]
                  }
                  frame #4 {
                    n197 = Wait (ms)(milliseconds to wait=250) -> ()  [unwired: 1 out]
                  }
                  frame #5 {
                    n198 = Generate User Event(user event=w298, event data cluster="" ("event data"), error in=w299) -> (error out=w301:errorcluster)  [unwired: 1 in, 1 out]
                  }
                }
              }
              frame #3 {
                w302 = FALSE ("Mode1 ON")
                w320 = u8 0 ("Disabled")
                # "Set enabled/disabled AVS channels"
                # "Reset pid parameters"
                # "Print VI version in the low left corner"
                # "Reset Current lists\nto first element"
                # "Hardware settings"
                # "Reset currents lists"
                # "Set initial controls state"
                n199 = call "Currents-Temp list - check ranges.vi"() -> ("I_list out"=w313:dbl[][])  [unwired: 5 in]
                n200 = property on="Start" class="Bool (strict)"("Visible"=TRUE, "Disabled"=u8 0, "Value"=FALSE ("start")) -> ()  [unwired: 2 in, 2 out]
                n201 = property on="CS.Mode1.List:Index" class="DigNum (strict)"("Val(Sgnl)"=1 ("Value (Signaling)")) -> ()  [unwired: 2 in, 2 out]
                n202 = property on="CS Mode" class="Enum (strict)"("Val(Sgnl)"=CS_mode."Manual" ("CS Mode")) -> ()  [unwired: 2 in, 2 out]
                n203 = local write "CS.Mode2.List"(w313) -> ()
                n204 = property on="CS.Mode1.List:To First" class="Bool (strict)"("Val(Sgnl)"=TRUE ("Value (Signaling)")) -> ()  [unwired: 2 in, 2 out]
                n205 = property on="CS.Mode1.Start" class="Bool (strict)"("Value"=w302) -> ()  [unwired: 2 in, 2 out]
                n206 = property on="CS.Mode2.Start" class="Bool (strict)"("Value"=w302) -> ()  [unwired: 2 in, 2 out]
                n207 = property on="CS.QCS I0 Output" class="Enum (strict)"("Disabled"=u8 2, "Val(Sgnl)"=T38."Channel 0" ("Map Channel 0 to")) -> ()  [unwired: 2 in, 2 out]
                n208 = property on="Bridge Type" class="Enum (strict)"("Disabled"=w320) -> ()  [unwired: 2 in, 2 out]
                n209 = property on="AVS GPIB Address" class="VISAName"("Disabled"=w320) -> ()  [unwired: 2 in, 2 out]
                n210 = property on="TCS RS232 Port" class="VISAName"("Disabled"=w320) -> ()  [unwired: 2 in, 2 out]
                n211 = property on="CS type" class="Enum (strict)"("Disabled"=w320) -> ()  [unwired: 2 in, 2 out]
                n212 = property on="CS.QCS Device Nr" class="DigNum (strict)"("Disabled"=w320) -> ()  [unwired: 2 in, 2 out]
                n213 = property on="Side Panel" class="TabCtl (strict)"("Value"=T34."Devices Settings" ("Tab Control 2")) -> ("Pages"=w307:refnum<vi>[])  [unwired: 2 in, 2 out]
                n214 = Index Array(array=w307, index=1) -> (element=w304:refnum<vi>)
                n215 = property class="App"() -> ("App.Kind"=w316:T60)  [unwired: 2 in, 2 out]
                n216 = property class="Page"(reference=w304, "PageEnb"=T51."Page Disabled & Grayed" ("Page Enabled State")) -> ()  [unwired: 1 in, 2 out]
                n217 = case shown="\"Run Time System\"" w316 {
                  tunnel: [w325 w336] -> w317
                  frame "invalid app kind", Default {
                    n218 = control-ref of="This VI"() -> (w332:refnum<vi>)
                    n219 = property class="VI"(reference=w332) -> ("Hist.Revision"=w331:u32)  [unwired: 1 in, 2 out]
                    n220 = Divide(x=w331, y=1000.0 ("x")) -> (x/y=w327:dbl)
                    n221 = Number To Fractional String(use system decimal point (T)=FALSE, number=w327, precision (6)=i16 2) -> (F-format string=w326:string)  [unwired: 1 in]
                    n222 = Concatenate Strings("" ("string"), w326) -> (w325:string)
                  }
                  frame "Run Time System" {
                    n223 = Current VI's Path() -> (path=w338:path)
                    n224 = Strip Path(path=w338) -> (stripped path=w337:path)  [unwired: 1 out]
                    n225 = Path To String(path=w337) -> (string=w335:string)
                    n226 = invoke class="FileVersionInfo" method="GetVersionInfo"(reference=refnum<k24> refnum (".NET object"), "fileName"=w335) -> ("GetVersionInfo"=w334:refnum<k24>)  [unwired: 2 in, 3 out]
                    n227 = property class="FileVersionInfo"(reference=w334) -> ("FileVersion"=w336:string)  [unwired: 1 in, 2 out]
                  }
                }
                "VI Version" <- w317
                n228 = property on="Channels Panel" class="TabCtl (strict)"("Val(Sgnl)"=T8."All" ("Value (Signaling)")) -> ()  [unwired: 2 in, 2 out]
                n229 = local write "CS.Mode1.PID Error"(0.0 ("T_error")) -> ()
                n230 = Generate User Event(user event=w310, event data cluster=bool[] [] ("event data")) -> ()  [unwired: 2 in, 2 out]
              }
            }
            n231 = Bundle By Name(cluster=w207, "Config folder"=w203, "Config File"=w205, "Calibrations Folder"=w204, "zBridge dll"=w202, "Variables Library"=w201) -> (w206:T50)
          }
        }
      }
      event "Start": Value Change {
        # "\"Start\" button clicked -> start measuring"
        n232 = event-data() -> ()  [unwired: 1 in, 6 out]
        n233 = Unbundle By Name(w342) -> ("Config File"=w339:path, "zBridge dll"=w340:path, "Config folder"=w341:path)
        n234 = stacked-sequence {
          tunnel: w343 -> [_ _ _ _ _ _ w470]
          tunnel: w341 -> [_ _ _ _ w412 _ _]
          tunnel: w340 -> [_ _ _ _ w411 _ _]
          tunnel: w339 -> [_ w353 _ _ _ _ _]
          frame #0 {
            n235 = property on="Run Description" class="Str"() -> ("Value"=w346:string)  [unwired: 2 in, 2 out]
            n236 = property on="Query Description" class="Bool (strict)"() -> ("Value"=w345:bool)  [unwired: 2 in, 2 out]
            n237 = Not(x=w345) -> (.not. x?=w344:bool)
            n238 = call "Run Reference DLG.vi"("Enable"=w345, "Run Reference"=w346, "Dont' ask again"=w344) -> ("Dont' ask again"=w348:bool, "Run Reference"=w349:string, "OK"=w350:bool)  [unwired: 13 in, 1 out]
            n239 = Not(x=w348) -> (.not. x?=w347:bool)
            n240 = case shown="True" w350 {
              tunnel: w349 -> [_ w352]
              tunnel: w347 -> [_ w351]
              frame False {
              }
              frame True {
                n241 = property on="Run Description" class="Str"("Val(Sgnl)"=w352) -> ()  [unwired: 2 in, 2 out]
                n242 = property on="Query Description" class="Bool (strict)"("Val(Sgnl)"=w351) -> ()  [unwired: 2 in, 2 out]
              }
            }
          }
          frame #1 {
            # "Save new settings to config file"
            n243 = control-ref of="zBridge.Active Channels"() -> (w357:refnum<vi>)
            n244 = control-ref of="CS.Mode1.PID"() -> (w356:refnum<vi>)
            n245 = control-ref of="CS.Mode1.Settings"() -> (w355:refnum<vi>)
            n246 = control-ref of="CS.Mode1.Settings"() -> (w354:refnum<vi>)
            n247 = control-ref of="CS Cannel Names"() -> (w360:refnum<vi>)
            n248 = control-ref of="AVS names"() -> (w359:refnum<vi>)
            n249 = control-ref of="_CurCalibrations"() -> (w358:refnum<vi>)
            n250 = control-ref of="Bridge settings"() -> (w365:refnum<vi>)
            n251 = control-ref of="Runtime Settings"() -> (w366:refnum<vi>)
            n252 = control-ref of="CS Settings"() -> (w364:refnum<vi>)
            n253 = control-ref of="Sensor Calibrations"() -> (w367:refnum<vi>)
            n254 = control-ref of="PID setup"() -> (w368:refnum<vi>)
            n255 = control-ref of="Data Logging Settings"() -> (w363:refnum<vi>)
            n256 = Build Array(w357, w365, w366, w364, w363, w367, w368, w360, w359, w358, w356, w355, w354) -> (w361:refnum<vi>[])
            n257 = call "Save Load Settings to File by Ref with path.vi"("Array of Cluster References"=w361, "Action"=enum8{"Load", "Save"}."Save", "Configuration file"=w353) -> ()  [unwired: 6 in, 1 out]
          }
          frame #2 {
            w384 = u8 2 ("Disabled")
            # "Reset stop button"
            # "Hide Disable Start button"
            # "Load external calibration VI"
            # "Set controls\nInitialize data for run"
            # "Lock hardware settings"
            n258 = property on="Bridge Type" class="Enum (strict)"("Disabled"=w384) -> ()  [unwired: 2 in, 2 out]
            n259 = property on="AVS GPIB Address" class="VISAName"("Disabled"=w384) -> ()  [unwired: 2 in, 2 out]
            n260 = property on="AVS RS232 Port" class="VISAName"("Disabled"=w384) -> ()  [unwired: 2 in, 2 out]
            n261 = property on="TCS RS232 Port" class="VISAName"("Disabled"=w384) -> ()  [unwired: 2 in, 2 out]
            n262 = property on="CS type" class="Enum (strict)"("Disabled"=w384) -> ()  [unwired: 2 in, 2 out]
            n263 = property on="CS.QCS Device Nr" class="DigNum (strict)"("Disabled"=w384) -> ()  [unwired: 2 in, 2 out]
            n264 = property on="CS.QCS I0 Output" class="Enum (strict)"("Disabled"=u8 0) -> ()  [unwired: 2 in, 2 out]
            n265 = call "Current Time(double).vi"() -> ("Current Time (double)"=w373:dbl)  [unwired: 6 in, 1 out]
            n266 = local write "_TimeOld"(w373) -> ()
            n267 = property on="External VI Path" class="Path"() -> ("Value"=w383:path)  [unwired: 2 in, 2 out]
            n268 = vi-ref "OnTempStabilizedRef.vi"() -> (w382:refnum<vi>)
            n269 = local write "VI called?"(FALSE ("VI called?")) -> ()
            n270 = Open VI Reference(type specifier VI Refnum (for type only)=w382, vi path=w383) -> (vi reference=→"_ExtVIReference":refnum<vi>)  [unwired: 4 in, 1 out]
            n271 = property on="Start" class="Bool (strict)"("Visible"=TRUE, "Disabled"=u8 2) -> ()  [unwired: 2 in, 2 out]
            n272 = Initialize Array(cluster{"R":dbl[], "T":dbl[], "Time":dbl[]} {"R"=[], "T"=[], "Time"=[]}, 10 ("dimension size")) -> (w377:cluster{"R":dbl[], "T":dbl[], "Time":dbl[]}[])
            n273 = local write "Data Array"(w377) -> ()
            n274 = disable-structure shown="Enabled" {
              frame Enabled {
                n275 = property on="Stop" class="Bool (strict)"("Value"=FALSE ("MainStopButton")) -> ()  [unwired: 2 in, 2 out]
              }
              frame Disabled {
              }
            }
            n276 = property on="Side Panel" class="TabCtl (strict)"() -> ("Pages"=w372:refnum<vi>[])  [unwired: 2 in, 2 out]
            n277 = Index Array(array=w372, index=1) -> (element=w370:refnum<vi>)
            n278 = property class="Page"(reference=w370, "PageEnb"=T51."Page Enabled" ("Page Enabled State")) -> ()  [unwired: 1 in, 2 out]
          }
          frame #3 {
            # "Initialize CS"
            n279 = local read "_CSClassRef"() -> (w396:refnum<class "CS.lvclass">)
            n280 = call-dynamic "Initialize.vi"("CS in"=w396, "HW Address"="_CS_Address", "error in (no error)"=T52 {"error"=FALSE, "code"=0, "source"=""} ("error in")) -> ("CS out"=w389:refnum<class "CS.lvclass">, "Instrument ID"=→"CS.ID":string, "error out"=w388:errorcluster)  [unwired: 10 in]
            n281 = call-dynamic "Get Currents & Ranges.vi"("CS.lvclass in"=w389, "error in (no error)"=w388) -> ("CS.lvclass out"=w397:refnum<class "CS.lvclass">, "I0"=w398:cluster{"Value":dbl, "Range":dbl}, "I1"=w390:cluster{"Value":dbl, "Range":dbl}, "I2"=w391:cluster{"Value":dbl, "Range":dbl}, "I3"=w392:cluster{"Value":dbl, "Range":dbl}, "error out"=w394:errorcluster)  [unwired: 12 in]
            "CS status" <- w394
            n282 = local write "_CSClassRef"(w397) -> ()
            n283 = Unbundle By Name(w394) -> ("status"=w386:bool)
            n284 = case shown="False" w386 {
              tunnel: w390 -> [w410 _]
              tunnel: w391 -> [w409 _]
              tunnel: w392 -> [w408 _]
              tunnel: w398 -> [w402 _]
              frame False {
                n285 = Unbundle By Name(w402) -> ("Value"=w401:dbl, "Range"=w400:dbl)
                n286 = Unbundle By Name(w410) -> ("Value"=w407:dbl, "Range"=w406:dbl)
                n287 = Unbundle By Name(w409) -> ("Value"=w405:dbl, "Range"=w404:dbl)
                n288 = Unbundle By Name(w408) -> ("Value"=w399:dbl, "Range"=w403:dbl)
                n289 = property on="I" class="DigNum (strict)"("Value"=w401) -> ()  [unwired: 2 in, 2 out]
                n290 = property on="I" class="DigNum (strict)"("Value"=w407) -> ()  [unwired: 2 in, 2 out]
                n291 = property on="I" class="DigNum (strict)"("Value"=w405) -> ()  [unwired: 2 in, 2 out]
                n292 = property on="I" class="DigNum (strict)"("Value"=w399) -> ()  [unwired: 2 in, 2 out]
                n293 = property on="Range" class="Enum (strict)"("Value"=w400) -> ()  [unwired: 2 in, 2 out]
                n294 = property on="Range" class="Enum (strict)"("Value"=w406) -> ()  [unwired: 2 in, 2 out]
                n295 = property on="Range" class="Enum (strict)"("Value"=w404) -> ()  [unwired: 2 in, 2 out]
                n296 = property on="Range" class="Enum (strict)"("Value"=w403) -> ()  [unwired: 2 in, 2 out]
              }
              frame True {
              }
            }
          }
          frame #4 {
            # "Initialize AVS/zBridge"
            n297 = property on="Bridge Type" class="Enum (strict)"() -> ("Value"=w417:T61)  [unwired: 2 in, 2 out]
            n298 = case shown="\"AVS47A (GPIB interface)\"" w417 {
              tunnel: [w423 w432 w448 refnum<visa-resource-name> refnum ("dup VISA session") refnum<visa-resource-name> refnum ("dup VISA session")] -> w416
              tunnel: [w422 w435 _ w456 errorcluster {"status"=FALSE, "code"=0, "source"=""} ("error out")] -> w415
              tunnel: [_ _ w447 _ _] -> _
              tunnel: w412 -> [_ _ _ w453 _]
              tunnel: w411 -> [_ _ _ w452 _]
              frame "AVS47A (GPIB interface)" {
                # "Set default Parameters,\n enable Autoranging"
                n299 = property on="AVS GPIB Address" class="VISAName"() -> ("Value"=w418:refnum<visa-resource-name>)  [unwired: 2 in, 2 out]
                n300 = call "AVS47IB Initialize.vi"("Instr. Descriptor (GPIB::)"=w418) -> ("VISA session"=w431:refnum<visa-resource-name>, "error out"=w419:errorcluster)  [unwired: 13 in]
                n301 = call "AVS47IB Stop.vi"("VISA session"=w431, "error in (no error)"=w419) -> ("dup VISA session"=w429:refnum<visa-resource-name>, "error out"=w421:errorcluster)  [unwired: 12 in]
                n302 = call "AVS47IB Go Remote.vi"("VISA session"=w429, "error in (no error)"=w421) -> ("dup VISA session"=w430:refnum<visa-resource-name>, "error out"=w420:errorcluster)  [unwired: 12 in]
                n303 = call "AVS47IB Configure 47IB.vi"("VISA session"=w430, "Printer Enabled (-1:no change)"=i8 0, "Buffer Enabled (-1:no change)"=i8 0, "Message Headers Included  (-1:no change)"=i8 0, "Autoranging Enabled (-1:no change)"=i8 1, "Stabilisation Delay (-1:no change)"=i8 15, "error in (no error)"=w420) -> ("dup VISA session"=w423:refnum<visa-resource-name>, "error out"=w422:errorcluster)  [unwired: 7 in]
              }
              frame "AVS47B (RS232 interface)" {
                n304 = property on="Bridge settings" class="Clust (strict)"() -> ("Value"=w439:T35)  [unwired: 2 in, 2 out]
                n305 = Unbundle By Name(w439) -> ("AVS RS232 Port"=w438:refnum<visa-resource-name>)
                n306 = call "InitPort_b.vi"("VISA resource"=w438) -> ("error out"=w434:errorcluster, "dup VISA resource"=w437:refnum<visa-resource-name>)  [unwired: 5 in]
                n307 = Type Cast(type=refnum<visa-resource-name> refnum ("dup VISA session"), x=w437) -> (*(type *) &x=w433:refnum<visa-resource-name>)
                n308 = case shown="Error" w434 {
                  selector: w434 -> [w440 w443]
                  tunnel: w433 -> [w441 w445]
                  tunnel: [w440 w444] -> w435
                  tunnel: [w441 refnum<visa-resource-name> refnum ("dup VISA session")] -> w432
                  frame No Error {
                  }
                  frame Error {
                    n309 = VISA Close(VISA resource name=w445, error in (no error)=w443) -> (error out=w444:errorcluster)
                  }
                }
              }
              frame "AVS48SI (RS232 interface)" {
                n310 = property on="Bridge settings" class="Clust (strict)"() -> ("Value"=w451:T35)  [unwired: 2 in, 2 out]
                n311 = Unbundle By Name(w451) -> ("AVS RS232 Port"=w449:refnum<visa-resource-name>)
                n312 = call "Configure Hardware.vi"("VISA RESOURCE NAME"=w449) -> ("THREAD OUT"=w446:string)  [unwired: 14 in]
                n313 = call "Configure Sensor Wiring of CHs.vi"("THREAD IN"=w446) -> ("THREAD OUT"=w447:string)  [unwired: 10 in]
                n314 = Type Cast(type=refnum<visa-resource-name> refnum ("dup VISA session"), x=w449) -> (*(type *) &x=w448:refnum<visa-resource-name>)
              }
              frame "Impedance Bridge" {
                n315 = call "SetParFilePath.vi"("path"=w453, "zDll"=w452) -> ("error out"=w455:errorcluster, "zDll out"=w454:path)  [unwired: 8 in]
                n316 = call "StartScan.vi"("error in (no error)"=w455, "path in"=w454) -> ("error out"=w456:errorcluster)  [unwired: 8 in, 1 out]
              }
              frame "Disabled", Default {
              }
            }
            "_AVS_VISA" <- w416
            n317 = property on="Bridge status" class="Clust (strict)"("Value"=w415) -> ()  [unwired: 2 in, 2 out]
            n318 = property on="_ScanData" class="Arr (strict)"("Value"=dbl[] [0.0, 0.0, 0.0, 0.0, 0.0, 0.0, 0.0, 0.0, 0.0, 0.0] ("R_array")) -> ()  [unwired: 2 in, 2 out]
            n319 = call "ScanParameters FGV.vi"("Action"=Action."Init") -> ()  [unwired: 10 in, 1 out]
          }
          frame #5 {
            # "Generate paths for log files"
            n320 = Unbundle By Name("Data Logging Settings") -> ("Run Description"=w463:string, "Filenames Suffix"=w464:string, "Log Files Folder"=w461:path, "Log Files Name"=w467:string, "Automode Files Name"=w466:string)
            n321 = call "Create Dir if Non-Existant__ogtk.vi"("Directory Path"=w461) -> ("dup Directory Path"=w460:path)  [unwired: 8 in, 2 out]
            n322 = call "MGI Make String Filesafe.vi"("String In"=w463) -> ("Filesafe String Out"=w462:string)
            n323 = call "GeneratePaths.vi"("Filename Suffix"=w464, "Run description"=w462, "AVS_Path"=w460, "AVS_FName"=w467, "CAL_Path"=w460, "CAL_FName"=w466) -> ("Generated Log path"=w465:path, "Generated Calib path"=→"_CalibFilesPath":path)  [unwired: 8 in]
            n324 = property on="_LogFilesPath" class="Path"("Val(Sgnl)"=w465) -> ()  [unwired: 2 in, 2 out]
          }
          frame #6 {
            # "Start measurements"
            n325 = Set Occurrence(w470) -> ()
          }
        }
      }
      event "Stop": Value Change; Application Instance Close {
        # "\"Stop\" button pressed -> Stop measuring."
        n326 = event-data() -> ()  [unwired: 1 in, 1 out]
        n327 = flat-sequence {
          tunnel: w472 -> [w475]
          tunnel: w473 -> [w490]
          tunnel: w471 -> [w504]
          frame #0 {
            # "Save settings to config file"
            n328 = control-ref of="zBridge.Active Channels"() -> (w478:refnum<vi>)
            n329 = control-ref of="Bridge settings"() -> (w485:refnum<vi>)
            n330 = control-ref of="Runtime Settings"() -> (w484:refnum<vi>)
            n331 = control-ref of="CS Settings"() -> (w486:refnum<vi>)
            n332 = control-ref of="Data Logging Settings"() -> (w487:refnum<vi>)
            n333 = control-ref of="Sensor Calibrations"() -> (w483:refnum<vi>)
            n334 = control-ref of="PID Settings"() -> (w482:refnum<vi>)
            n335 = control-ref of="CS Cannel Names"() -> (w481:refnum<vi>)
            n336 = control-ref of="Channel names"() -> (w480:refnum<vi>)
            n337 = control-ref of="Curent Calibrations"() -> (w479:refnum<vi>)
            n338 = control-ref of="CS.Mode1.PID"() -> (w477:refnum<vi>)
            n339 = control-ref of="CS.Mode1.Settings"() -> (w476:refnum<vi>)
            n340 = Build Array(w478, w485, w484, w486, w487, w483, w482, w481, w480, w479, w477, w476) -> (w489:refnum<vi>[])
            n341 = call "Save Load Settings to File by Ref with path.vi"("Array of Cluster References"=w489, "Action"=enum8{"Load", "Save"}."Save", "Configuration file"=w475) -> ()  [unwired: 6 in, 1 out]
          }
          frame #1 {
            # "Free serial ports"
            n342 = control-ref of="_AVS_VISA"() -> (w491:refnum<vi>)
            n343 = control-ref of="TCS RS232 Port"() -> (w496:refnum<vi>)
            n344 = call "StopScan.vi"("path in"=w490) -> ()  [unwired: 9 in, 2 out]
            n345 = property class="VISAName"(reference=w491) -> (error out=w493:errorcluster, "Value"=w492:refnum<visa-resource-name>)  [unwired: 1 in, 1 out]
            n346 = property class="VISAName"(reference=w496) -> (error out=w494:errorcluster, "Value"=w495:refnum<visa-resource-name>)  [unwired: 1 in, 1 out]
            n347 = VISA Close(VISA resource name=w492, error in (no error)=w493) -> ()  [unwired: 1 out]
            n348 = VISA Close(VISA resource name=w495, error in (no error)=w494) -> ()  [unwired: 1 out]
          }
          frame #2 {
            w498 = u8 0 ("Disabled")
            # "Reset controls state"
            n349 = property on="Bridge Type" class="Enum (strict)"("Disabled"=w498) -> ()  [unwired: 2 in, 2 out]
            n350 = property on="AVS GPIB Address" class="VISAName"("Disabled"=w498) -> ()  [unwired: 2 in, 2 out]
            n351 = property on="AVS RS232 Port" class="VISAName"("Disabled"=w498) -> ()  [unwired: 2 in, 2 out]
            n352 = property on="TCS RS232 Port" class="VISAName"("Disabled"=w498) -> ()  [unwired: 2 in, 2 out]
            n353 = property on="CS type" class="Enum (strict)"("Disabled"=w498) -> ()  [unwired: 2 in, 2 out]
            n354 = property on="CS.QCS Device Nr" class="DigNum (strict)"("Disabled"=w498) -> ()  [unwired: 2 in, 2 out]
            n355 = property on="Start" class="Bool (strict)"("Visible"=TRUE, "Disabled"=u8 0, "Value"=FALSE ("start")) -> ()  [unwired: 2 in, 2 out]
            n356 = property on="Stop" class="Bool (strict)"("Value"=FALSE ("MainStopButton")) -> ()  [unwired: 2 in, 2 out]
          }
          frame #3 {
            w502 = u8 2 ("Disabled")
            # "Disable UI"
            n357 = property on="Top Toolbar" class="TabCtl (strict)"("Disabled"=w502) -> ()  [unwired: 2 in, 2 out]
            n358 = property on="Main Panel" class="TabCtl (strict)"("Disabled"=w502) -> ()  [unwired: 2 in, 2 out]
            n359 = property on="CS Indicators Panel" class="TabCtl (strict)"("Disabled"=w502) -> ()  [unwired: 2 in, 2 out]
            n360 = property on="Side Panel" class="TabCtl (strict)"("Disabled"=w502) -> ()  [unwired: 2 in, 2 out]
            n361 = property on="Lower Panel" class="TabCtl (strict)"("Disabled"=w502) -> ()  [unwired: 2 in, 2 out]
            n362 = property on="_String" class="Str"("Visible"=TRUE) -> ()  [unwired: 2 in, 2 out]
          }
          frame #4 {
            n363 = invoke class="App" method="Library.UndeployLibrary"("libPath"=w504) -> ()  [unwired: 4 in, 5 out]
          }
          frame #5 {
            # "Stop \nexecution"
            n364 = Stop(stop? (T)=TRUE) -> ()
          }
        }
        n365 = Unbundle By Name(w474) -> ("Variables Library"=w471:path, "zBridge dll"=w473:path, "Config File"=w472:path)
      }
      event "_ScanData": Value Change {
        # "Convert 8 elements AVS\narray to 10 elements"
        # "Received new data from AVS/zBridge. Do general tasks - update indicators, calculate temperature and pass the data further to AVS/zBridge specific processing"
        n366 = event-data() -> ("NewVal"=w522:dbl[])  [unwired: 1 in]
        n367 = Unbundle By Name(w510) -> ("UpdateValuesAVS"=w508:refnum<user-event>, "UpdateValuesZBridge"=w509:refnum<user-event>)
        n368 = Unbundle By Name(w506) -> ("Calibrations Folder"=w507:path)
        n369 = for {
          tunnel: w522 -> [w551] mode=indexing
          tunnel: [w549] -> w518 mode=indexing
          n370 = Less?(x=w551, y=1e+25) -> (x < y?=w552:bool)
          n371 = Select(t=w551, s=w552, f=inf) -> (s? t:f=w549:dbl)
        }
        n372 = Index Array(array=w518) -> (element #1=→"R0":dbl, element #2=→"R1":dbl, element #3=→"R2":dbl, element #4=→"R3":dbl, element #5=→"R4":dbl, element #6=→"R5":dbl, element #7=→"R6":dbl, element #8=→"R7":dbl, element #9=→"R8":dbl, element #10=→"R9":dbl)  [unwired: 10 in]
        n373 = Array To Cluster(array=w518) -> (cluster=w512:T62)
        "R Cluster" <- w512
        n374 = Cluster To Array(cluster=w512) -> (array=w511:dbl[])
        n375 = Absolute Value(x=w511) -> (abs(x)=w519:dbl[])
        n376 = property on="Allow neg R" class="Bool (strict)"() -> ("Value"=w517:bool)  [unwired: 2 in, 2 out]
        n377 = Select(t=w511, s=w517, f=w519) -> (s? t:f=w516:dbl[])
        "R Array" <- w516
        n378 = local read "_CurCalibrations"() -> (w524:T33)
        n379 = Cluster To Array(cluster=w524) -> (array=w523:string[])
        n380 = call "Resistance to Temp no Ext.vi"("error in"=w525, "Path"=w507, "CurCalibrations"=w523, "Resistance"=w516) -> ("Temperature"=w514:dbl[])  [unwired: 1 in, 3 out]
        "T Array" <- w514
        n381 = Array To Cluster(array=w514) -> (cluster=w530:T63)
        "T Cluster" <- w530
        n382 = Unbundle(w530) -> ("Temperature[0]"=→"T0":dbl, "Temperature[1]"=→"T1":dbl, "Temperature[2]"=→"T2":dbl, "Temperature[3]"=→"T3":dbl, "Temperature[4]"=→"T4":dbl, "Temperature[5]"=→"T5":dbl, "Temperature[6]"=→"T6":dbl, "Temperature[7]"=→"T7":dbl, "Temperature[8]"=→"T8":dbl, "Temperature[9]"=→"T9":dbl)
        n383 = property on="Mode Buttons" class="RadioBtnsControl (strict)"() -> ("Value"=w529:T7)  [unwired: 2 in, 2 out]
        n384 = Array To Cluster(array=w516) -> (cluster=w515:T62)
        n385 = Array To Cluster(array=w514) -> (cluster=w513:T63)
        n386 = case shown="\"No Selection\", Default" w529 {
          tunnel: w513 -> [w564 _]
          tunnel: w515 -> [w565 _]
          frame "No Selection", Default {
            n387 = call "Current Time(double).vi"() -> ("Current Time (double)"=→"Time":dbl)  [unwired: 6 in, 1 out]
            "Small R Cluster" <- w565
            "Small T Cluster" <- w564
          }
          frame "Cursor mode" {
          }
        }
        n388 = Bundle(w516, "Temperature"=w514) -> (w527:cluster{dbl[], "Temperature":dbl[]})  [unwired: 1 in]
        n389 = property on="Bridge Type" class="Enum (strict)"() -> ("Value"=w526:T61)  [unwired: 2 in, 2 out]
        n390 = case shown="\"AVS47B (RS232 interface)\", Default" w526 {
          tunnel: [w557 w558 w561] -> w528
          tunnel: w525 -> [w556 w558 w562]
          tunnel: w527 -> [w555 _ w560]
          tunnel: w509 -> [_ _ w559]
          tunnel: w508 -> [w554 _ _]
          frame "AVS47B (RS232 interface)", Default {
            n391 = Generate User Event(user event=w554, event data cluster=w555, error in=w556) -> (error out=w557:errorcluster)  [unwired: 1 in, 1 out]
          }
          frame "Disabled" {
          }
          frame "Impedance Bridge" {
            n392 = Generate User Event(user event=w559, event data cluster=w560, error in=w562) -> (error out=w561:errorcluster)  [unwired: 1 in, 1 out]
          }
        }
      }
      event User Event {
        # "Process data from the AVS bridge"
        n393 = event-data() -> ("R"=w570:dbl[], "T"=w569:dbl[])  [unwired: 1 in]
        n394 = property on="CS.Actual Current" class="Arr (strict)"() -> ("Value"=w571:dbl[])  [unwired: 2 in, 2 out]
        n395 = Unbundle By Name(w568) -> ("CS Automode"=w567:refnum<user-event>)
        n396 = stacked-sequence {
          tunnel: w573 -> [_ w591 w651]
          tunnel: [_ w615 _] -> w572
          tunnel: w571 -> [_ w592 w649]
          tunnel: w570 -> [w581 w594 w647]
          tunnel: w569 -> [w580 w593 w648]
          tunnel: w567 -> [w578 _ _]
          frame #0 {
            # "Filter data and add it to the data array. \nDo PID"
            n397 = property on="Runtime Settings" class="Clust (strict)"() -> ("Value"=w584:T27)  [unwired: 2 in, 2 out]
            n398 = Unbundle By Name(w584) -> ("Y_max"=w587:dbl, "Y_min"=w586:dbl, "Filter Graphs"=w585:bool)
            n399 = local read "Data Array"() -> (w582:T28)
            n400 = property on="Data Memory" class="DigNum (strict)"() -> ("Value"=w589:u16)  [unwired: 2 in, 2 out]
            n401 = call "Current Time(double).vi"() -> ("Current Time (double)"=w579:dbl)  [unwired: 6 in, 1 out]
            n402 = call "Manage Data Arrays - AVS.vi"("Y_max"=w587, "Y_min"=w586, "Filter Graph Results"=w585, "Append New Data"=TRUE, "Data In"=w582, "Curr R"=w581, "Curr T"=w580, "Curr Time"=w579, "Data Memory"=w589) -> ("Data Out"=w583:T28)  [unwired: 10 in]
            n403 = Bundle("Current Time (double)"=w579, "R"=w581, "T"=w580) -> (w590:T64)  [unwired: 1 in]
            n404 = local write "Data Array"(w583) -> ()
            n405 = Generate User Event(user event=w578, event data cluster=w590) -> ()  [unwired: 2 in, 2 out]
            n406 = Initialize Array("Ohm" ("AVS Name 0"), 10 ("dimension size")) -> (w577:string[])
            n407 = Array To Cluster(array=w577) -> (cluster=w574:T33)
            n408 = local write "Units"(w574) -> ()
          }
          frame #1 {
            # "Save data to log file"
            n409 = local read "_LogFilesPath"() -> (w613:path)
            n410 = local read "_CalibFilesPath"() -> (w614:path)
            n411 = call <vilib>:"Check if File or Folder Exists.vi"("path"=w613) -> ("file or folder exists?"=w605:bool, "dup path"=w606:path)  [unwired: 8 in, 1 out]
            n412 = case shown="False" w605 {
              tunnel: w606 -> [w638 w645]
              tunnel: [w638 w645] -> w607
              tunnel: [w636 _] -> w599
              frame False {
                n413 = control-ref of="Sensor Calibrations"() -> (w641:refnum<vi>)
                n414 = property on="Run Description" class="Str"() -> ("Value"=w637:string)  [unwired: 2 in, 2 out]
                n415 = Cluster To Array(cluster="Sensor Names") -> (array=w643:string[])
                n416 = Cluster To Array(cluster="CS Cannel Names") -> (array=w644:string[])
                n417 = call "Format log file header Z.vi"("Thermometer"=w641, "AVS names"=w643, "CS Names"=w644, "Run description"=w637) -> ("String"=w639:string)  [unwired: 1 in]
                n418 = Write to Text File(file (use dialog)=w638, text=w639) -> (error out=w636:errorcluster)  [unwired: 2 in, 2 out]
              }
              frame True {
              }
            }
            n419 = property on="Data Logging Settings" class="Clust (strict)"() -> ("Value"=w624:T37)  [unwired: 2 in, 2 out]
            n420 = Unbundle By Name(w624) -> ("Delimeter"=w597:string, "Date Format"=w623:string)
            n421 = call "Current Time(double).vi"() -> ("Current Time"=w600:timestamp, "Current Time (double)"=w601:dbl)  [unwired: 6 in]
            n422 = call "File Info__ogtk.vi"("error in (no error)"=w599, "file"=w607) -> ("error out"=w598:errorcluster, "file info"=w603:T65, "file out"=w612:path)  [unwired: 4 in]
            n423 = Unbundle By Name(w603) -> ("creation date"=w604:u32)
            n424 = Number To Exponential String(number=w601, precision (6)=i16 10) -> (E-format string=w595:string)  [unwired: 2 in]
            n425 = Format Date/Time String(time format string (%c)=w623, seconds (now)=w600) -> (date/time string=w620:string)  [unwired: 1 in]
            n426 = Number To Fractional String(number=w594) -> (F-format string=w622:string[])  [unwired: 3 in]
            n427 = Number To Fractional String(number=w593) -> (F-format string=w621:string[])  [unwired: 3 in]
            n428 = Number To Fractional String(number=w592) -> (F-format string=w619:string[])  [unwired: 3 in]
            n429 = property on="New File Interval" class="DigNum (strict)"() -> ("Value"=w608:u32)  [unwired: 2 in, 2 out]
            n430 = property on="New File Interval Units" class="Enum (strict)"() -> ("Value"=w609:enum16{"Minutes", "Hours", "Days"})  [unwired: 2 in, 2 out]
            n431 = To Time Stamp(1:w604) -> (0:w610:timestamp)
            n432 = Build Array (concatenate)(w620, w595, w622, w621, w619) -> (w596:string[])
            n433 = call "Time Elapsed time.vi"("Time Units"=w609, "Delay Time"=w608, "Time Old In"=w610) -> ("T>dT?"=w611:bool)  [unwired: 2 out]
            n434 = case shown="True" w611 {
              tunnel: [w626 w629] -> w602
              tunnel: [w625 w630] -> _
              tunnel: w612 -> [w626 _]
              tunnel: w614 -> [w625 _]
              frame False {
              }
              frame True {
                n435 = local read "Data Logging Settings"() -> (w631:T37)
                n436 = Unbundle By Name(w631) -> ("Run Description"=w627:string, "Log Files Folder"=w635:path, "Log Files Name"=w633:string, "Automode Files Name"=w634:string, "Filenames Suffix"=w632:string)
                n437 = call "MGI Make String Filesafe.vi"("String In"=w627) -> ("Filesafe String Out"=w628:string)
                n438 = call "GeneratePaths.vi"("Filename Suffix"=w632, "Run description"=w628, "AVS_Path"=w635, "AVS_FName"=w633, "CAL_Path"=w635, "CAL_FName"=w634) -> ("Generated Log path"=w629:path, "Generated Calib path"=w630:path)  [unwired: 8 in]
                n439 = local write "_CalibFilesPath"(w630) -> ()
                n440 = property on="_LogFilesPath" class="Path"("Val(Sgnl)"=w629) -> ()  [unwired: 2 in, 2 out]
              }
            }
            n441 = call "Write To Spreadsheet File (string) w Error.vi"("delimiter (\\t)"=w597, "append to file? (new file:F)"=TRUE, "error in"=w598, "1D data"=w596, "file path (dialog if empty)"=w602) -> ("error out"=w616:errorcluster)  [unwired: 5 in, 1 out]
            n442 = Merge Errors(w616, w591) -> (w615:errorcluster)
          }
          frame #2 {
            # "Add frame with code for writing to DSC"
            n443 = local read "Bridge settings"() -> (w654:T35)
            n444 = local read "Sensor Names"() -> (w652:T10)
            n445 = Unbundle By Name(w654) -> ("Bridge Type"=w656:T61)
            n446 = property on="Sensor Calibrations" class="Clust (strict)"() -> ("Controls[]"=w653:refnum<vi>[])  [unwired: 2 in, 2 out]
            n447 = To Unsigned Long Integer(number=w656) -> (unsigned 32bit integer=w657:u32)
            n448 = Variant To Data(error in=w651, type=T54."AVS47A (GPIB interface)" ("AVS type"), Variant=w657) -> (data=w655:T54, error out=w650:errorcluster)
            n449 = Bundle By Name(cluster=T55 {"R"=[], "T"=[], "I"=[], "AVS type"=enum."AVS47A (GPIB interface)", "AVS names"={"AVS Name 0"="", "AVS Name 1"="", "AVS Name 2"="", "AVS Name 3"="", "AVS Name 4"="", "AVS Name 5"="", "AVS Name 6"="", "AVS Name 7"="", "AVS Name 8"="", "AVS Name 9"=""}, "Calibration"=[]} ("TC Cluster"), "Calibration"=w653, "AVS names"=w652, "R"=w647, "T"=w648, "I"=w649, "AVS type"=w655) -> (w659:T55)
            n450 = call "TC_to_DSC.vi"("error in (no error)"=w650, "TC Cluster"=w659) -> ()  [unwired: 9 in, 1 out]
          }
        }
      }
      event User Event {
        # "Process data from the zBridge bridge"
        n451 = event-data() -> ("R"=w669:dbl[], "T"=w668:dbl[])  [unwired: 1 in]
        n452 = property on="CS.Actual Current" class="Arr (strict)"() -> ("Value"=w667:dbl[])  [unwired: 2 in, 2 out]
        n453 = local read "_zBridgeParText"() -> (w664:string)
        n454 = local read "_zBridgeSetNr"() -> (w670:u8)
        n455 = local read "_ZBridgeUnit"() -> (w665:string)
        n456 = Unbundle By Name(w663) -> ("CS Automode"=w662:refnum<user-event>)
        n457 = stacked-sequence {
          tunnel: w664 -> [w691 _ _]
          tunnel: w670 -> [w676 _ w713]
          tunnel: w669 -> [w674 w698 w739]
          tunnel: w668 -> [w673 w697 w738]
          tunnel: w667 -> [_ w696 w737]
          tunnel: w666 -> [_ w702 w736]
          tunnel: [_ _ w735] -> w661
          tunnel: w665 -> [w678 _ _]
          tunnel: w662 -> [w675 _ _]
          frame #0 {
            # "Only do PID after measuring\non selected channel( or any \nchannel if -1 is selected)"
            n458 = local read "zBridge params"() -> (w677:T19)
            n459 = local read "Units"() -> (w679:T13)
            n460 = Cluster To Array(cluster=w679) -> (array=w682:string[])
            n461 = Cluster To Array(cluster=w677) -> (array=w692:string[])
            n462 = Replace Array Subset(array=w682, new element=w678, index=w676) -> (w681:string[])
            n463 = Replace Array Subset(array=w692, new element=w691, index=w676) -> (w693:string[])
            n464 = Array To Cluster(array=w681) -> (cluster=→"Units":T66)
            n465 = Array To Cluster(array=w693) -> (cluster=→"zBridge params":T67)
            n466 = property on="Runtime Settings" class="Clust (strict)"() -> ("Value"=w685:T27)  [unwired: 2 in, 2 out]
            n467 = Unbundle By Name(w685) -> ("Y_max"=w688:dbl, "Y_min"=w687:dbl, "Filter Graphs"=w686:bool)
            n468 = local read "Data Array"() -> (w683:T28)
            n469 = property on="Data Memory" class="DigNum (strict)"() -> ("Value"=w690:u16)  [unwired: 2 in, 2 out]
            n470 = call "Current Time(double).vi"() -> ("Current Time (double)"=w671:dbl)  [unwired: 6 in, 1 out]
            n471 = call "Manage Data Arrays - zBridge.vi"("Y_max"=w688, "Y_min"=w687, "Filter Graph Results"=w686, "Append New Data"=TRUE, "Data In"=w683, "Curr R"=w674, "Curr T"=w673, "Curr Time"=w671, "Channel"=w676, "Data Memory"=w690) -> ("Data Out"=w684:T28)  [unwired: 9 in]
            n472 = local write "Data Array"(w684) -> ()
            n473 = Bundle("Current Time (double)"=w671, "R"=w674, "T"=w673) -> (w672:T64)  [unwired: 1 in]
            n474 = Generate User Event(user event=w675, event data cluster=w672) -> ()  [unwired: 2 in, 2 out]
          }
          frame #1 {
            # "New frame with code for writing to DSC"
            n475 = local read "Bridge settings"() -> (w705:T35)
            n476 = local read "Sensor Names"() -> (w703:T10)
            n477 = Unbundle By Name(w705) -> ("Bridge Type"=w707:T61)
            n478 = property on="Sensor Calibrations" class="Clust (strict)"() -> ("Controls[]"=w704:refnum<vi>[])  [unwired: 2 in, 2 out]
            n479 = To Unsigned Long Integer(number=w707) -> (unsigned 32bit integer=w708:u32)
            n480 = Variant To Data(error in=w702, type=T54."AVS47A (GPIB interface)" ("AVS type"), Variant=w708) -> (data=w706:T54, error out=w701:errorcluster)
            n481 = Bundle By Name(cluster=T55 {"R"=[], "T"=[], "I"=[], "AVS type"=enum."AVS47A (GPIB interface)", "AVS names"={"AVS Name 0"="", "AVS Name 1"="", "AVS Name 2"="", "AVS Name 3"="", "AVS Name 4"="", "AVS Name 5"="", "AVS Name 6"="", "AVS Name 7"="", "AVS Name 8"="", "AVS Name 9"=""}, "Calibration"=[]} ("TC Cluster"), "Calibration"=w704, "AVS names"=w703, "R"=w698, "T"=w697, "I"=w696, "AVS type"=w706) -> (w700:T55)
            n482 = call "TC_to_DSC.vi"("error in (no error)"=w701, "TC Cluster"=w700) -> ()  [unwired: 9 in, 1 out]
          }
          frame #2 {
            n483 = local read "_LogFilesPath"() -> (w716:path)
            n484 = local read "Data Logging Settings"() -> (w734:T37)
            n485 = call "Strip Path Extension - Path__ogtk.vi"("path"=w716) -> ("root"=w717:string, "extension"=w720:string)
            n486 = Format Into String(format string="_%d", initial string=w717, w713) -> (resulting string=w718:string)  [unwired: 1 in, 1 out]
            n487 = Concatenate Strings(w718, "." ("string"), w720) -> (w715:string)
            n488 = Unbundle By Name(w734) -> ("Delimeter"=w750:string, "Date Format"=w749:string)
            n489 = String To Path(string=w715) -> (path=w714:path)
            n490 = call <vilib>:"Check if File or Folder Exists.vi"("path"=w714) -> ("file or folder exists?"=w725:bool, "dup path"=w726:path)  [unwired: 8 in, 1 out]
            n491 = case shown="False" w725 {
              tunnel: w726 -> [w768 w771]
              tunnel: [w768 w771] -> w727
              tunnel: [w762 _] -> w710
              frame False {
                n492 = local read "CS Cannel Names"() -> (w766:T31)
                n493 = local read "Sensor Names"() -> (w767:T10)
                n494 = control-ref of="Sensor Calibrations"() -> (w770:refnum<vi>)
                n495 = property on="Run Description" class="Str"() -> ("Value"=w763:string)  [unwired: 2 in, 2 out]
                n496 = Cluster To Array(cluster=w767) -> (array=w764:string[])
                n497 = Cluster To Array(cluster=w766) -> (array=w765:string[])
                n498 = call "Format log file header Z.vi"("Thermometer"=w770, "AVS names"=w764, "CS Names"=w765, "Run description"=w763) -> ("String"=w769:string)  [unwired: 1 in]
                n499 = Write to Text File(file (use dialog)=w768, text=w769) -> (error out=w762:errorcluster)  [unwired: 2 in, 2 out]
              }
              frame True {
              }
            }
            n500 = call "Current Time(double).vi"() -> ("Current Time"=w711:timestamp, "Current Time (double)"=w712:dbl)  [unwired: 6 in]
            n501 = Number To Exponential String(number=w712, precision (6)=i16 10) -> (E-format string=w742:string)  [unwired: 2 in]
            n502 = Format Date/Time String(time format string (%c)=w749, seconds (now)=w711) -> (date/time string=w746:string)  [unwired: 1 in]
            n503 = Number To Exponential String(number=w739) -> (E-format string=w748:string[])  [unwired: 3 in]
            n504 = Number To Engineering String(4:w738) -> (0:w747:string[])  [unwired: 3 in]
            n505 = Number To Fractional String(number=w737) -> (F-format string=w745:string[])  [unwired: 3 in]
            n506 = call "File Info__ogtk.vi"("error in (no error)"=w710, "file"=w727) -> ("error out"=w709:errorcluster, "file info"=w723:T65, "file out"=w732:path)  [unwired: 4 in]
            n507 = Unbundle By Name(w723) -> ("creation date"=w724:u32)
            n508 = Build Array (concatenate)(w746, w742, w748, w747, w745) -> (w744:string[])
            n509 = local read "_CalibFilesPath"() -> (w733:path)
            n510 = property on="New File Interval" class="DigNum (strict)"() -> ("Value"=w728:u32)  [unwired: 2 in, 2 out]
            n511 = property on="New File Interval Units" class="Enum (strict)"() -> ("Value"=w729:enum16{"Minutes", "Hours", "Days"})  [unwired: 2 in, 2 out]
            n512 = To Time Stamp(1:w724) -> (0:w730:timestamp)
            n513 = call "Time Elapsed time.vi"("Time Units"=w729, "Delay Time"=w728, "Time Old In"=w730) -> ("T>dT?"=w731:bool)  [unwired: 2 out]
            n514 = case shown="True" w731 {
              tunnel: [w752 w755] -> w722
              tunnel: [w751 w757] -> _
              tunnel: w732 -> [w752 _]
              tunnel: w733 -> [w751 _]
              frame False {
              }
              frame True {
                n515 = local read "Data Logging Settings"() -> (w758:T37)
                n516 = Unbundle By Name(w758) -> ("Run Description"=w754:string, "Filenames Suffix"=w756:string, "Log Files Folder"=w761:path, "Log Files Name"=w759:string, "Automode Files Name"=w760:string)
                n517 = call "MGI Make String Filesafe.vi"("String In"=w754) -> ("Filesafe String Out"=w753:string)
                n518 = call "GeneratePaths.vi"("Filename Suffix"=w756, "Run description"=w753, "AVS_Path"=w761, "AVS_FName"=w759, "CAL_Path"=w761, "CAL_FName"=w760) -> ("Generated Log path"=w755:path, "Generated Calib path"=w757:path)  [unwired: 8 in]
                n519 = local write "_CalibFilesPath"(w757) -> ()
                n520 = property on="_LogFilesPath" class="Path"("Val(Sgnl)"=w755) -> ()  [unwired: 2 in, 2 out]
              }
            }
            n521 = call "Write To Spreadsheet File (string) w Error.vi"("delimiter (\\t)"=w750, "append to file? (new file:F)"=TRUE, "error in"=w709, "1D data"=w744, "file path (dialog if empty)"=w722) -> ("error out"=w740:errorcluster)  [unwired: 5 in, 1 out]
            n522 = Merge Errors(w740, w736) -> (w735:errorcluster)
          }
        }
      }
      event User Event {
        # "Current source automatic mode"
        n523 = event-data() -> ("R"=w778:dbl[], "T"=w779:dbl[], "Time"=w773:dbl)  [unwired: 1 in, 4 out]
        n524 = local read "CS.Mode"() -> (w777:T39)
        n525 = Unbundle By Name(w776) -> ("CallExtVI"=w775:refnum<user-event>, "TempStabilized"=w774:refnum<user-event>)
        n526 = case shown="\"Mode2\"" w777 {
          tunnel: w779 -> [_ w783 w858]
          tunnel: w778 -> [_ w784 w859]
          tunnel: w775 -> [_ w786 _]
          tunnel: w774 -> [_ w785 _]
          tunnel: w773 -> [_ w782 _]
          frame "Manual", Default {
          }
          frame "Mode 1" {
            n527 = call "MGI Change Detector (T).vi"("Value"="CS.Mode1.Start") -> ("Changed?"=w780:bool)
            n528 = case shown="True" "CS.Mode1.Start" {
              tunnel: w786 -> [_ w799]
              tunnel: w785 -> [_ w798]
              tunnel: w784 -> [_ w797]
              tunnel: w783 -> [_ w796]
              tunnel: w782 -> [_ w793]
              tunnel: w780 -> [_ w787]
              frame False {
              }
              frame True {
                # "Check if PID error (SP-PV)==0"
                # "Check if temperature\nis stabilized"
                # "T sabilized?"
                # "If TCS auto mode enabled and temperature is not changing => fire TempStabilized event to save log and set new CS point. Otherwise do PID (if enabled)."
                # "Check if stabilization delay time \nis elapsed"
                n529 = property on="R/T?" class="Enum (strict)"() -> ("Value"=w795:enum16{"Resistance", "Temperature"})  [unwired: 2 in, 2 out]
                n530 = case shown="\"Temperature\"" w795 {
                  tunnel: [w814 w815] -> w792
                  tunnel: w797 -> [w814 _]
                  tunnel: w796 -> [_ w815]
                  frame "Resistance", Default {
                  }
                  frame "Temperature" {
                  }
                }
                n531 = property on="Bridge Channel" class="DigNum (strict)"() -> ("Value"=w791:i32)  [unwired: 2 in, 2 out]
                n532 = Index Array(array=w792, index=w791) -> (element=w790:dbl)
                n533 = local read "CS.Mode1.PID Error"() -> (w806:dbl)
                n534 = property on="FB on 2" class="Enum (strict)"() -> ("Value"=w788:enum16{"0", "1", "2", "3"})  [unwired: 2 in, 2 out]
                n535 = local read "_CSMode1List[i]"() -> (w800:T23[])
                n536 = local read "_TimeOld"() -> (w812:dbl)
                n537 = property on="Delay Time" class="DigNum (strict)"() -> ("Value"=w802:dbl)  [unwired: 2 in, 2 out]
                n538 = property on="N averages" class="DigNum (strict)"() -> ("Value"=w789:i32)  [unwired: 2 in, 2 out]
                n539 = property on="T stability" class="DigNum (strict)"() -> ("Value"=w801:dbl)  [unwired: 2 in, 2 out]
                n540 = Equal To 0?(x=w806) -> (x = 0?=w804:bool)
                n541 = call "Derivatives Pt by Pt.vi"("initialize"=w787, "accuracy (%)"=w801, "Time"=w793, "Data"=w790, "Points to avg"=w789) -> ("Stable?"=w805:bool, "Stability (%)"=→"CS.Mode1.Slope":dbl, "dt (s)"=w809:dbl)  [unwired: 2 in]
                n542 = Index Array(array=w800, index=w788) -> (element=w813:T23)
                n543 = call "Time Elapsed dbl.vi"("Delay Time"=w802, "Time Old In"=w812) -> ("T>dT?"=w794:bool, "Delta T"=→"CS.Mode1.Timer":dbl, "Time New Out"=w811:dbl)  [unwired: 1 in]
                n544 = Compound Arithmetic op=AND(w794, w804, w805) -> (w807:bool)
                "CS.Mode1.PID Stabilized?" <- w807
                n545 = property on="Enable PID" class="Bool (strict)"() -> ("Value"=w803:bool)  [unwired: 2 in, 2 out]
                n546 = case shown="False" w807 {
                  tunnel: w811 -> [_ w835]
                  tunnel: w809 -> [w831 _]
                  tunnel: w803 -> [w821 _]
                  tunnel: w813 -> [w829 _]
                  tunnel: w800 -> [w826 _]
                  tunnel: w788 -> [w819 _]
                  tunnel: w799 -> [_ w833]
                  tunnel: w798 -> [_ w832]
                  tunnel: w790 -> [w818 _]
                  tunnel: w787 -> [w816 _]
                  frame False {
                    # "Temperature is not stable. If enabled, do PID regulation"
                    n547 = local read "CS.Current Value"() -> (w823:dbl[])
                    n548 = Index Array(array=w823, index=w819) -> (element=w824:dbl)
                    n549 = Multiply(x=1000.0, y=w824) -> (x*y=w822:dbl)
                    n550 = call "PID control incremental.vi"("Process Variable"=w818, "dt"=w831, "Setpoint"=w829, "PID Settings"="CS.Mode1.PID Settings", "I in"=w822, "PID Enabled"=w821, "Reset"=w816) -> ("PID output I"=→"Waveform Chart":T22, "err out"=→"CS.Mode1.PID Error":dbl, "I out"=w828:dbl)  [unwired: 9 in, 1 out]
                    n551 = Replace Array Subset(array=w826, new element=w828, index=w819) -> (→"CS.Automode Current":T23[])
                  }
                  frame True {
                    # "Temperature is stable & automode is on"
                    n552 = case shown="False" "CS.Mode1.Call VI?" {
                      tunnel: w835 -> [w838 _]
                      tunnel: w833 -> [_ w839]
                      tunnel: w832 -> [w836 _]
                      frame False {
                        # "External VI call disabled -> proceed\nwith automode"
                        n553 = local write "_TimeOld"(w838) -> ()
                        n554 = Generate User Event(user event=w836, event data cluster=TRUE ("event data")) -> ()  [unwired: 2 in, 2 out]
                      }
                      frame True {
                        # "Call external VI"
                        n555 = Generate User Event(user event=w839, event data cluster="" ("event data")) -> ()  [unwired: 2 in, 2 out]
                      }
                    }
                  }
                }
              }
            }
          }
          frame "Mode2" {
            n556 = Unbundle By Name("CS.Mode2.Settings") -> ("Hysteresis"=w841:u8, "Bridge Channel"=w842:i32, "FB on"=w843:enum16{"Resistance", "Temperature"})
            n557 = case shown="\"Resistance\", Default" w843 {
              tunnel: [w861 w862] -> w857
              tunnel: w859 -> [w861 _]
              tunnel: w858 -> [_ w862]
              frame "Resistance", Default {
              }
              frame "Temperature" {
              }
            }
            n558 = Index Array(array=w857, index=w842) -> (element=w856:dbl)
            n559 = local read "CS.Mode2.List"() -> (w855:dbl[][])
            n560 = call "Currents-Temp list  - T in range-.vi"("List in"=w855, "T"=w856, "T1 index"=1, "T0 index"=0, "Hysteresis"=w841) -> ("List index"=w849:i32, "I_out"=w848:dbl[])  [unwired: 1 out]
            n561 = case shown="True" "CS.Mode2.Start" {
              tunnel: w848 -> [_ w860]
              frame False {
              }
              frame True {
                n562 = local write "CS.Automode Current"(w860) -> ()
              }
            }
            n563 = Initialize Array(FALSE, 16 ("dimension size")) -> (w852:bool[])
            n564 = Replace Array Subset(array=w852, new element=TRUE ("new element/subarray"), index=w849) -> (→"CS.Mode2.Row":bool[])
          }
        }
      }
      event User Event {
        n565 = event-data() -> ()  [unwired: 1 in, 5 out]
        n566 = Unbundle By Name(w865) -> ("TempStabilized"=w864:refnum<user-event>)
        n567 = local read "_ExtVIReference"() -> (w869:refnum<vi>)
        n568 = call "GetExtVIStatus.vi"("vi reference in"=w869) -> ("vi reference out"=w866:refnum<vi>, "Exec.State"=w868:T46, "Finished?"=w867:bool)
        n569 = case shown="\"Idle\"" w868 {
          tunnel: w867 -> [_ _]
          tunnel: w866 -> [_ w871]
          tunnel: w864 -> [_ w870]
          frame "Bad", Default {
          }
          frame "Idle" {
            n570 = local read "VI called?"() -> (w872:bool)
            n571 = case shown="False" w872 {
              tunnel: w871 -> [w874 _]
              tunnel: w870 -> [_ w881]
              frame False {
                n572 = property on="_ScanData" class="Arr (strict)"() -> ("Value"=w877:dbl[])  [unwired: 2 in, 2 out]
                n573 = property on="T Array" class="Arr (strict)"() -> ("Value"=w878:dbl[])  [unwired: 2 in, 2 out]
                n574 = property on="CS.Current Value" class="Arr (strict)"() -> ("Value"=w879:dbl[])  [unwired: 2 in, 2 out]
                n575 = Format Date/Time String() -> (date/time string=w876:string)  [unwired: 3 in]
                n576 = Bundle("date/time string"=w876, "Value"=w877, "Value"=w878, "Value"=w879) -> (w875:T68)  [unwired: 1 in]
                n577 = call "CallExtVI.vi"("vi reference in"=w874, "Cluster"=w875) -> ()  [unwired: 1 out]
                "VI called?" <- TRUE ("VI called?")
              }
              frame True {
                n578 = call "Current Time(double).vi"() -> ("Current Time (double)"=w880:dbl)  [unwired: 6 in, 1 out]
                n579 = Generate User Event(user event=w881, event data cluster=TRUE ("event data")) -> ()  [unwired: 2 in, 2 out]
                n580 = local write "_TimeOld"(w880) -> ()
              }
            }
          }
        }
      }
      event User Event {
        # "CS automode\nT is stabilized"
        n581 = event-data() -> ("TempStabilized"=w885:bool)  [unwired: 1 in, 4 out]
        n582 = stacked-sequence {
          tunnel: w886 -> [w892 _]
          tunnel: [w893 _] -> w884
          tunnel: w885 -> [_ w913]
          frame #0 {
            # "Step1: Save R,T,I values to calibration file. Make screenshot when creating the calibration file."
            n583 = property on="_CalibFilesPath" class="Path"() -> ("Value"=w888:path)  [unwired: 2 in, 2 out]
            n584 = call "File Exists - Scalar__ogtk.vi"("file path"=w888) -> ("exists"=w889:bool)  [unwired: 6 in, 1 out]
            n585 = case shown="False" w889 {
              tunnel: w888 -> [w902 w912]
              tunnel: [w902 w912] -> w887
              frame False {
                n586 = local read "CS Cannel Names"() -> (w908:T31)
                n587 = local read "Sensor Names"() -> (w909:T10)
                n588 = property on="Run Description" class="Str"() -> ("Value"=w905:string)  [unwired: 2 in, 2 out]
                n589 = control-ref of="Sensor Calibrations"() -> (w911:refnum<vi>)
                n590 = Cluster To Array(cluster=w909) -> (array=w906:string[])
                n591 = Cluster To Array(cluster=w908) -> (array=w907:string[])
                n592 = call "Format log file header Z.vi"("Thermometer"=w911, "AVS names"=w906, "CS Names"=w907, "Run description"=w905) -> ("String"=w910:string)  [unwired: 1 in]
                n593 = control-ref of="This VI"() -> (w904:refnum<vi>)
                n594 = Write to Text File(file (use dialog)=w902, text=w910) -> ()  [unwired: 2 in, 3 out]
                n595 = invoke class="VI" method="FP.Get Image"(reference=w904) -> ("image data"=w903:T69)  [unwired: 5 in, 5 out]
                n596 = call "Convert File Extension (Path)__ogtk.vi"("new ending (none)"="png" ("name or relative path"), "file name"=w902) -> ("new filename"=w901:path)  [unwired: 1 out]
                n597 = call <vilib>:"Write PNG File.vi"("image data"=w903, "path to PNG file"=w901) -> ()  [unwired: 8 in, 2 out]
              }
              frame True {
              }
            }
            n598 = local write "VI called?"(FALSE ("VI called?")) -> ()
            n599 = property on="Data Logging Settings" class="Clust (strict)"() -> ("Value"=w896:T37)  [unwired: 2 in, 2 out]
            n600 = Unbundle By Name(w896) -> ("Date Format"=w897:string, "Delimeter"=w894:string)
            n601 = property on="R" class="Clust (strict)"() -> ("Value"=w895:T14)  [unwired: 2 in, 2 out]
            n602 = property on="T" class="Clust (strict)"() -> ("Value"=w899:T9)  [unwired: 2 in, 2 out]
            n603 = property on="CS.Current Value" class="Arr (strict)"() -> ("Value"=w898:dbl[])  [unwired: 2 in, 2 out]
            n604 = call "Write to cal log file.vi"("Value 2"=w898, "Date/Time Format"=w897, "Value 3"=w899, "Value"=w895, "Delimeter"=w894, "Value 4"=w887) -> ("error out"=w891:errorcluster)  [unwired: 1 out]
            n605 = Merge Errors(w891, w892) -> (w893:errorcluster)
          }
          frame #1 {
            # "Step 2: Sweep through the currents list"
            n606 = case shown="True" w913 {
              frame False {
              }
              frame True {
                n607 = local read "CS.Mode1.List:Count"() -> (w915:i32)
                n608 = local read "CS.Mode1.List:Index"() -> (w916:i32)
                n609 = Less?(x=w916, y=w915) -> (x < y?=w914:bool)
                n610 = case shown="False" w914 {
                  frame False {
                    n611 = property on="CS Mode" class="Enum (strict)"("Val(Sgnl)"=CS_mode."Manual" ("CS Mode")) -> ()  [unwired: 2 in, 2 out]
                  }
                  frame True {
                    n612 = property on="CS.Mode1.List:Next" class="Bool (strict)"("Val(Sgnl)"=TRUE) -> ()  [unwired: 2 in, 2 out]
                  }
                }
              }
            }
          }
        }
      }
      event User Event {
        # "Disable controls for disabled channels"
        n613 = event-data() -> ()  [unwired: 1 in, 5 out]
        n614 = Unbundle By Name(w920) -> ("zBridge dll"=w919:path)
        n615 = property on="Bridge Type" class="Enum (strict)"() -> ("Value"=w928:T61)  [unwired: 2 in, 2 out]
        n616 = case shown="Default" w928 {
          tunnel: [w938 w950 w958] -> w927
          tunnel: w919 -> [_ w949 _]
          frame Default {
            n617 = property on="Runtime Settings" class="Clust (strict)"() -> ("Value"=w942:T27)  [unwired: 2 in, 2 out]
            n618 = Unbundle By Name(w942) -> ("Read AVS channels from"=w940:i8, "Last Channel"=w941:i8)
            n619 = for {
              N: 10 -> [_]
              tunnel: w941 -> [w944]
              tunnel: w940 -> [w945]
              tunnel: [w943] -> w938 mode=indexing
              i -> [w946]
              n620 = Less Or Equal?(x=w945, y=w946) -> (x <= y?=w948:bool)
              n621 = Less Or Equal?(x=w946, y=w944) -> (x <= y?=w947:bool)
              n622 = And(x=w948, y=w947) -> (x .and. y?=w943:bool)
            }
          }
          frame "Impedance Bridge" {
            n623 = for {
              N: 10 -> [_]
              tunnel: [w953] -> w951 mode=indexing
              tunnel: w949 -> [w954]
              i -> [w956]
              n624 = call "GetByteParam.vi"("ParNo"=u8 0, "SetNo"=w956, "zDll"=w954) -> ("return type"=w953:u8)  [unwired: 6 in, 2 out]
            }
            n625 = Greater Than 0?(x=w951) -> (x > 0?=w950:bool[])
          }
          frame "AVS47B (RS232 interface)" {
            n626 = local read "zBridge.Active Channels"() -> (w957:T21)
            n627 = Cluster To Array(cluster=w957) -> (array=w958:bool[])
          }
        }
        n628 = control-ref of="zBridge.Active Channels"() -> (w934:refnum<vi>)
        n629 = control-ref of="AVS Exc&Ranges"() -> (w930:refnum<vi>)
        n630 = control-ref of="R"() -> (w935:refnum<vi>)
        n631 = control-ref of="Sensor Calibrations"() -> (w936:refnum<vi>)
        n632 = control-ref of="T"() -> (w937:refnum<vi>)
        n633 = control-ref of="uPlots"() -> (w931:refnum<vi>)
        n634 = control-ref of="AVS names"() -> (w929:refnum<vi>)
        n635 = control-ref of="zBridge params"() -> (w926:refnum<vi>)
        n636 = control-ref of="zBridge.Scan Phase"() -> (w925:refnum<vi>)
        n637 = control-ref of="Units"() -> (w924:refnum<vi>)
        n638 = control-ref of="AVS names small"() -> (w923:refnum<vi>)
        n639 = control-ref of="Small R Cluster"() -> (w922:refnum<vi>)
        n640 = control-ref of="Small T Cluster"() -> (w921:refnum<vi>)
        n641 = Build Array(w934, w930, w935, w936, w937, w931, w929, w926, w925, w924, w923, w922, w921) -> (w932:refnum<vi>[])
        n642 = Array Size(array=w932) -> (size(s)=w933:i32)
        n643 = for {
          N: w933 -> [_]
          tunnel: w932 -> [w962] mode=indexing
          tunnel: w927 -> [w959]
          n644 = property class="Clust"(reference=w962) -> ("Controls[]"=w960:refnum<vi>[])  [unwired: 1 in, 2 out]
          n645 = Array Size(array=w960) -> (size(s)=w961:i32)
          n646 = for {
            N: w961 -> [_]
            tunnel: w960 -> [w964] mode=indexing
            tunnel: w959 -> [w963] mode=indexing
            n647 = case shown="True" w963 {
              tunnel: w964 -> [w965 w970]
              frame False {
                n648 = property class="Ctl"(reference=w965, "Disabled"=u8 2) -> ("ClassName"=w966:string)  [unwired: 1 in, 2 out]
                n649 = case shown="\"Boolean\"" w966 {
                  tunnel: w965 -> [_ w969 _]
                  frame "False", Default {
                  }
                  frame "Boolean" {
                    n650 = property class="Ctl"(reference=w969, "Value"=FALSE) -> ()  [unwired: 1 in, 2 out]
                  }
                  frame "Ring" {
                  }
                }
              }
              frame True {
                n651 = property class="Ctl"(reference=w970, "Disabled"=u8 0) -> ("ClassName"=w971:string)  [unwired: 1 in, 2 out]
                n652 = case shown="\"False\", Default" w971 {
                  tunnel: w970 -> [_ w974]
                  frame "False", Default {
                  }
                  frame "Boolean" {
                    n653 = property class="Ctl"(reference=w974, "Value"=TRUE) -> ()  [unwired: 1 in, 2 out]
                  }
                }
              }
            }
          }
        }
      }
      event Mouse Down? {
        n654 = event-data() -> ("CtlRef"=w976:refnum<vi>, "Mods.Double Click"=w975:bool)  [unwired: 1 in]
        n655 = disable-structure shown="Enabled" {
          disable-tunnel: w975 -> [w979 _]
          disable-tunnel: w976 -> [w978 _]
          frame Enabled {
            n656 = case shown="True" w979 {
              tunnel: w978 -> [_ w998]
              frame False {
              }
              frame True {
                w994 = 128  # call and forget
                n657 = property class="Ctl"(reference=w998) -> ("Label.Text"=w997:string)  [unwired: 1 in, 2 out]
                n658 = local read "Sensor Names"() -> (w985:T10)
                n659 = call "Slice String 1__ogtk.vi"("Subset (i:j)"="-1", "String"=w997) -> ("Substring (String[i:j])"=w995:string)  [unwired: 7 in]
                n660 = Decimal String To Number(string=w995) -> (number=w980:i32)  [unwired: 2 in, 1 out]
                n661 = Cluster To Array(cluster=w985) -> (array=w984:string[])
                n662 = Index Array(array=w984, index=w980) -> (element=w983:string)
                n663 = vi-ref "Text Popup.vi"() -> (w991:refnum<vi>)
                n664 = property class="VI"(reference=w991) -> (error out=w992:errorcluster, "Name"=w993:string)  [unwired: 1 in, 1 out]
                n665 = Open VI Reference(type specifier VI Refnum (for type only)=refnum<vi> refnum, vi path=w993, options=w994, error in (no error)=w992) -> (vi reference=w990:refnum<vi>, error out=w987:errorcluster)  [unwired: 2 in]
                n666 = control-ref of="T Array"() -> (w981:refnum<vi>)
                n667 = control-ref of="R Array"() -> (w982:refnum<vi>)
                n668 = call-by-ref "Start Asynchronous Call"(reference=w990, error in=w987, "Title"=w983, "R_array"=w982, "T_array"=w981, "Index"=w980) -> (reference out=w988:refnum<vi>, error out=w986:errorcluster)  [unwired: 16 in]
                n669 = Close Reference(reference=w988, error in (no error)=w986) -> ()  [unwired: 1 out]
              }
            }
          }
          frame Disabled {
          }
        }
        n670 = event-data() -> ()  [unwired: 2 in, 1 out]
      }
      event "_LogFilesPath": Value Change {
        # "Modify window title to show measurement information"
        n671 = event-data() -> ("NewVal"=w1008:path)  [unwired: 1 in, 5 out]
        n672 = property class="App"() -> ("App.Dir"=w1000:path)  [unwired: 2 in, 2 out]
        n673 = property on="Run Description" class="Str"() -> ("Value"=w1001:string)  [unwired: 2 in, 2 out]
        n674 = property on="Bridge Type" class="Enum (strict)"() -> ("RingText.Text"=w1002:string)  [unwired: 2 in, 2 out]
        n675 = property on="CS type" class="Enum (strict)"() -> ("RingText.Text"=w1003:string)  [unwired: 2 in, 2 out]
        n676 = Path To String(path=w1008) -> (string=w1004:string)
        n677 = Strip Path(path=w1000) -> (name=w999:string)  [unwired: 1 out]
        n678 = Format Into String(format string="%s - %s - %s - %s   (%s)", w999, w1001, w1002, w1003, w1004) -> (resulting string=w1006:string)  [unwired: 2 in, 1 out]
        n679 = control-ref of="This VI"() -> (w1009:refnum<vi>)
        n680 = property class="VI"(reference=w1009, "Front Panel.Title"=w1006) -> ()  [unwired: 1 in, 2 out]
      }
      event "Reload Calibrations", "Bridge settings.Calibrations Folder": Value Change {
        # "Refresh the list of calibration files"
        n681 = event-data() -> ()  [unwired: 1 in, 1 out]
        n682 = property on="Calibrations Folder" class="Path"() -> ("Value"=w1010:path)  [unwired: 2 in, 2 out]
        n683 = control-ref of="Sensor Calibrations"() -> (w1019:refnum<vi>)
        n684 = control-ref of="_CurCalibrations"() -> (w1013:refnum<vi>)
        n685 = control-ref of="Calibrations Folder"() -> (w1017:refnum<vi>)
        n686 = control-ref of="_QuickConvertCal"() -> (w1016:refnum<vi>)
        n687 = control-ref of="Sensor 1"() -> (w1018:refnum<vi>)
        n688 = Bundle By Name(cluster=w1012, "Calibrations Folder"=w1010) -> (w1011:T50)
        n689 = call "ReloadCalibrations.vi"("error in (no error)"=w1015, "Quick convert sensors"=w1016, "CurCalibrations"=w1013, "Calibration files path"=w1017, "Channel1 sensors"=w1018, "Channels list"=w1019) -> ("error out"=w1014:errorcluster)  [unwired: 1 in]
      }
      event Value Change {
        w1026 = refnum<vi> refnum  # XYGraph
        # "Show cursor on plot is \"Cursor\" or \"Delete points\" mode is enabled"
        # "!!NOTE:This routine assumes that XY graph is control #0 on tab page!!"
        n690 = event-data() -> ("NewVal"=w1022:T7)  [unwired: 1 in, 5 out]
        n691 = property on="Channels Panel" class="TabCtl (strict)"() -> ("Pages"=w1030:refnum<vi>[], "Value"=w1029:T8)  [unwired: 2 in, 2 out]
        n692 = Index Array(array=w1030, index=w1029) -> (element=w1028:refnum<vi>)
        n693 = property class="Page"(reference=w1028) -> ("ControlsOnPage"=w1023:refnum<vi>[])  [unwired: 1 in, 2 out]
        n694 = Index Array(array=w1023, index=0) -> (element=w1027:refnum<vi>)
        n695 = Type Cast(type=w1026, x=w1027) -> (*(type *) &x=w1021:refnum<vi>)
        n696 = case shown="\"Erase range\"" w1022 {
          tunnel: w1021 -> [w1031 w1040 w1048 w1056]
          frame "No Selection", Default {
            n697 = property class="XYGraph"(reference=w1031, "Active Cursor"=u32 0, "Cursor.Visible"=FALSE) -> (reference out=w1034:refnum<vi>)  [unwired: 1 in, 1 out]
            n698 = property class="XYGraph"(reference=w1034, "Active Cursor"=u32 1, "Cursor.Visible"=FALSE) -> ()  [unwired: 1 in, 2 out]
          }
          frame "Erase range" {
            n699 = property class="XYGraph"(reference=w1040, "Active Cursor"=u32 0, "Cursor.Visible"=TRUE, "Cursor.Cursor Color"=u32 16777062, "Cursor.Cursor Index"=0, "ActPaletteTool"=0 ("Palette:Active Tool")) -> (reference out=w1043:refnum<vi>)  [unwired: 1 in, 1 out]
            n700 = property class="XYGraph"(reference=w1043, "Active Cursor"=u32 1, "Cursor.Visible"=TRUE, "Cursor.Cursor Color"=u32 6618880) -> ()  [unwired: 1 in, 2 out]
          }
          frame "Cursor mode" {
            n701 = property class="XYGraph"(reference=w1048, "Active Cursor"=u32 0, "Cursor.Visible"=TRUE, "Cursor.Cursor Color"=u32 6618880, "ActPaletteTool"=0 ("Palette:Active Tool")) -> (reference out=w1051:refnum<vi>)  [unwired: 1 in, 1 out]
            n702 = property class="XYGraph"(reference=w1051, "Active Cursor"=u32 1, "Cursor.Visible"=FALSE) -> ()  [unwired: 1 in, 2 out]
          }
          frame "Erase point" {
            n703 = property class="XYGraph"(reference=w1056, "Active Cursor"=u32 0, "Cursor.Visible"=TRUE, "Cursor.Cursor Color"=u32 16777062, "ActPaletteTool"=0 ("Palette:Active Tool")) -> (reference out=w1059:refnum<vi>)  [unwired: 1 in, 1 out]
            n704 = property class="XYGraph"(reference=w1059, "Active Cursor"=u32 1, "Cursor.Visible"=FALSE) -> ()  [unwired: 1 in, 2 out]
          }
        }
      }
      event "R-Plot 0", "R-Plot 1", "R-Plot 2", "R-Plot 3", "R-Plot 4", "R-Plot 5", "R-Plot 6", "R-Plot 7", "R-Plot 8", "R-Plot 9": Mouse Down? {
        # "Disabled"
        n705 = event-data() -> ("CtlRef"=w1065:refnum<vi>, "Button"=w1070:u16, "Mods.Double Click"=w1067:bool)  [unwired: 1 in, 5 out]
        n706 = Equal?(x=u16 1, y=w1070) -> (x = y?=w1068:bool)
        n707 = And(x=w1068, y=w1067) -> (x .and. y?=w1066:bool)
        n708 = disable-structure shown="Disabled" {
          disable-tunnel: w1066 -> [w1073 _]
          disable-tunnel: w1065 -> [w1072 _]
          disable-tunnel: "Mode Buttons" -> [w1071 _]
          frame Disabled {
            n709 = case shown="True" w1073 {
              tunnel: w1071 -> [_ w1075]
              tunnel: w1072 -> [_ w1074]
              frame False {
              }
              frame True {
                n710 = case shown="\"Erase range\"" w1075 {
                  tunnel: w1074 -> [_ w1076]
                  frame "No Selection", Default {
                  }
                  frame "Erase range" {
                    n711 = property class="XYGraph (strict)"(reference=w1076, "ActPaletteTool"=0 ("Palette:Active Tool"), "Active Cursor"=u32 0, "Cursor.Visible"=TRUE) -> ()  [unwired: 1 in, 2 out]
                  }
                }
              }
            }
          }
          frame Enabled {
          }
        }
        n712 = event-data() -> ()  [unwired: 5 in, 1 out]
      }
      event "R-Plot 0", "R-Plot 1", "R-Plot 2", "R-Plot 3", "R-Plot 4", "R-Plot 5", "R-Plot 6", "R-Plot 7", "R-Plot 8", "R-Plot 9": Mouse Down {
        # "Process (double) click on plots in special modes (\"Cursor\", \"Erase\")"
        n713 = event-data() -> ("CtlRef"=w1083:refnum<vi>, "Coords"=w1086:T70, "Button"=w1082:u16, "Mods.Double Click"=w1085:bool, "PlatMods"=w1081:T71)  [unwired: 1 in, 3 out]
        n714 = property on="Mode Buttons" class="RadioBtnsControl (strict)"() -> ("Value"=w1084:T7)  [unwired: 2 in, 2 out]
        n715 = case shown="1" w1082 {
          tunnel: w1086 -> [_ _ w1091]
          tunnel: w1085 -> [_ _ w1090]
          tunnel: w1084 -> [_ _ w1089]
          tunnel: w1083 -> [_ _ w1088]
          tunnel: w1081 -> [_ _ _]
          frame 2 {
          }
          frame Default {
          }
          frame 1 {
            n716 = case shown="\"Cursor mode\"" w1089 {
              tunnel: w1088 -> [_ w1094 w1115 w1123]
              tunnel: w1091 -> [_ w1093 w1114 w1125]
              tunnel: w1090 -> [_ w1092 w1116 w1124]
              frame "No Selection", Default {
              }
              frame "Cursor mode" {
                n717 = case shown="True" w1092 {
                  tunnel: w1094 -> [_ w1104]
                  tunnel: w1093 -> [_ w1102]
                  frame False {
                  }
                  frame True {
                    n718 = invoke class="XYGraph (strict)" method="Map Coords To XY"(reference=w1104, "Coords"=w1102) -> (reference out=w1103:refnum<vi>, "XY"=w1101:cluster{"X":dbl, "Y":dbl})  [unwired: 5 in, 5 out]
                    n719 = Unbundle By Name(w1101) -> ("X"=w1099:dbl)
                    n720 = local read "Data Array"() -> (w1100:T28)
                    n721 = property class="XYGraph (strict)"(reference=w1103, "Active Cursor"=u32 0, "Cursor.Cursor Position"=w1101) -> ()  [unwired: 1 in, 2 out]
                    n722 = for {
                      tunnel: w1100 -> [w1113] mode=indexing
                      tunnel: w1099 -> [w1111]
                      tunnel: [w1107] -> w1098 mode=indexing
                      tunnel: [w1106] -> w1097 mode=indexing
                      n723 = Unbundle By Name(w1113) -> ("R"=w1110:dbl[], "T"=w1109:dbl[], "Time"=w1112:dbl[])
                      n724 = Threshold 1D Array(2:w1111, 3:w1112) -> (0:w1108:dbl)  [unwired: 1 in]
                      n725 = Index Array(array=w1110, index=w1108) -> (element=w1107:dbl)
                      n726 = Index Array(array=w1109, index=w1108) -> (element=w1106:dbl)
                    }
                    n727 = Array To Cluster(array=w1097) -> (cluster=w1095:T62)
                    n728 = Array To Cluster(array=w1098) -> (cluster=w1096:T62)
                    n729 = property on="Time" class="DigNum (strict)"("Value"=w1099) -> ()  [unwired: 2 in, 2 out]
                    n730 = property on="Small R Cluster" class="Clust (strict)"("Value"=w1096) -> ()  [unwired: 2 in, 2 out]
                    n731 = property on="Small T Cluster" class="Clust (strict)"("Value"=w1095) -> ()  [unwired: 2 in, 2 out]
                  }
                }
              }
              frame "Erase range" {
                n732 = case shown="False" w1116 {
                  tunnel: w1115 -> [w1120 _]
                  tunnel: w1114 -> [w1119 _]
                  frame False {
                    n733 = invoke class="XYGraph (strict)" method="Map Coords To XY"(reference=w1120, "Coords"=w1119) -> (reference out=w1122:refnum<vi>, "XY"=w1117:cluster{"X":dbl, "Y":dbl})  [unwired: 5 in, 5 out]
                    n734 = property class="XYGraph (strict)"(reference=w1122, "Active Cursor"=u32 0, "Cursor.Cursor Position"=w1117, "Active Cursor"=u32 1, "Cursor.Cursor Position"=w1117) -> ()  [unwired: 1 in, 2 out]
                  }
                  frame True {
                  }
                }
              }
              frame "Erase point" {
                n735 = case shown="True" w1124 {
                  tunnel: w1123 -> [w1130 w1145]
                  tunnel: w1125 -> [w1129 _]
                  frame False {
                    n736 = invoke class="XYGraph (strict)" method="Map Coords To XY"(reference=w1130, "Coords"=w1129) -> (reference out=w1128:refnum<vi>, "XY"=w1127:cluster{"X":dbl, "Y":dbl})  [unwired: 5 in, 5 out]
                    n737 = property class="XYGraph (strict)"(reference=w1128, "Active Cursor"=u32 0, "Cursor.Cursor Position"=w1127) -> ()  [unwired: 1 in, 2 out]
                  }
                  frame True {
                    n738 = property class="XYGraph (strict)"(reference=w1145, "Active Cursor"=u32 0) -> ("Cursor.Cursor X"=w1133:dbl)  [unwired: 1 in, 2 out]
                    n739 = local read "Channels Panel"() -> (w1132:T8)
                    n740 = local read "Data Array"() -> (w1131:T28)
                    n741 = Index Array(array=w1131, index=w1132) -> (element=w1138:cluster{"R":dbl[], "T":dbl[], "Time":dbl[]})
                    n742 = Unbundle By Name(w1138) -> ("R"=w1134:dbl[], "T"=w1135:dbl[], "Time"=w1136:dbl[])
                    n743 = Threshold 1D Array(2:w1133, 3:w1136) -> (0:w1137:dbl)  [unwired: 1 in]
                    n744 = Delete From Array(array=w1134, index=w1137) -> (array with subset deleted=w1141:dbl[])  [unwired: 1 in, 1 out]
                    n745 = Delete From Array(array=w1135, index=w1137) -> (array with subset deleted=w1140:dbl[])  [unwired: 1 in, 1 out]
                    n746 = Delete From Array(array=w1136, index=w1137) -> (array with subset deleted=w1139:dbl[])  [unwired: 1 in, 1 out]
                    n747 = Bundle By Name(cluster=w1138, "R"=w1141, "T"=w1140, "Time"=w1139) -> (w1142:cluster{"R":dbl[], "T":dbl[], "Time":dbl[]})
                    n748 = Replace Array Subset(array=w1131, new element=w1142, index=w1132) -> (w1143:T28)
                    n749 = local write "Data Array"(w1143) -> ()
                  }
                }
              }
            }
            "_LMBDown" <- TRUE ("Mouse down")
          }
        }
      }
      event "R-Plot 0", "R-Plot 1", "R-Plot 2", "R-Plot 3", "R-Plot 4", "R-Plot 5", "R-Plot 6", "R-Plot 7", "R-Plot 8", "R-Plot 9": Mouse Move {
        # "Process mouse movement over plots in special modes (\"Cursor\", \"Erase\")"
        n750 = event-data() -> ("CtlRef"=w1148:refnum<vi>, "Coords"=w1149:T70)  [unwired: 1 in, 3 out]
        n751 = property on="Mode Buttons" class="RadioBtnsControl (strict)"() -> ("Value"=w1152:T7)  [unwired: 2 in, 2 out]
        n752 = local read "_LMBDown"() -> (w1153:bool)
        n753 = Equal?(x=w1152, y=Cursor_Controls."Erase range" ("Mode Buttons")) -> (x = y?=w1150:bool)
        n754 = And(x=w1153, y=w1150) -> (x .and. y?=w1151:bool)
        n755 = case shown="True" w1151 {
          tunnel: w1149 -> [_ w1155]
          tunnel: w1148 -> [_ w1154]
          frame False {
          }
          frame True {
            n756 = invoke class="XYGraph (strict)" method="Map Coords To XY"(reference=w1154, "Coords"=w1155) -> (reference out=w1158:refnum<vi>, "XY"=w1157:cluster{"X":dbl, "Y":dbl})  [unwired: 5 in, 5 out]
            n757 = property class="XYGraph (strict)"(reference=w1158, "Active Cursor"=u32 1, "Cursor.Cursor Position"=w1157) -> ()  [unwired: 1 in, 2 out]
          }
        }
      }
      event "R-Plot 0", "R-Plot 1", "R-Plot 2", "R-Plot 3", "R-Plot 4", "R-Plot 5", "R-Plot 6", "R-Plot 7", "R-Plot 8", "R-Plot 9": Mouse Up {
        n758 = event-data() -> ("CtlRef"=w1162:refnum<vi>, "Button"=w1160:u16)  [unwired: 1 in, 6 out]
        n759 = property on="Mode Buttons" class="RadioBtnsControl (strict)"() -> ("Value"=w1163:T7)  [unwired: 2 in, 2 out]
        n760 = property class="XYGraph (strict)"(reference=w1162) -> ("ActPaletteTool"=w1161:i32)  [unwired: 1 in, 2 out]
        n761 = case shown="1" w1160 {
          tunnel: w1163 -> [_ w1167]
          tunnel: w1162 -> [_ w1166]
          tunnel: w1161 -> [_ w1165]
          frame Default {
          }
          frame 1 {
            n762 = local read "_LMBDown"() -> (w1164:bool)
            n763 = case shown="0" w1165 {
              tunnel: w1167 -> [_ w1172]
              tunnel: w1166 -> [_ w1171]
              tunnel: w1164 -> [_ w1169]
              frame Default {
                n764 = property on="Mode Buttons" class="RadioBtnsControl (strict)"("Val(Sgnl)"=T56."No Selection" ("Value (Signaling)")) -> ()  [unwired: 2 in, 2 out]
              }
              frame 0 {
                n765 = Equal?(x=w1172, y=T56."Erase range") -> (x = y?=w1175:bool)
                n766 = And(x=w1169, y=w1175) -> (x .and. y?=w1174:bool)
                n767 = case shown="True" w1174 {
                  tunnel: w1171 -> [_ w1198]
                  frame False {
                  }
                  frame True {
                    n768 = local read "Channels Panel"() -> (w1197:T8)
                    n769 = property class="XYGraph (strict)"(reference=w1198, "Active Cursor"=u32 0, "Active Cursor"=u32 1) -> ("Cursor.Cursor X"=w1195:dbl, "Cursor.Cursor X"=w1176:dbl)  [unwired: 1 in, 2 out]
                    n770 = local read "Data Array"() -> (w1192:T28)
                    n771 = Max & Min(x=w1195, y=w1176) -> (max(x,y)=w1185:dbl, min(x,y)=w1178:dbl)
                    n772 = Index Array(array=w1192, index=w1197) -> (element=w1188:cluster{"R":dbl[], "T":dbl[], "Time":dbl[]})
                    n773 = Unbundle By Name(w1188) -> ("R"=w1186:dbl[], "T"=w1187:dbl[], "Time"=w1184:dbl[])
                    n774 = Threshold 1D Array(2:w1185, 3:w1184) -> (0:w1182:dbl)  [unwired: 1 in]
                    n775 = Threshold 1D Array(2:w1178, 3:w1184) -> (0:w1183:dbl)  [unwired: 1 in]
                    n776 = Subtract(x=w1182, y=w1183) -> (x-y=w1181:dbl)
                    n777 = Delete From Array(array=w1186, length=w1181, index=w1183) -> (array with subset deleted=w1191:dbl[])  [unwired: 1 out]
                    n778 = Delete From Array(array=w1187, length=w1181, index=w1183) -> (array with subset deleted=w1190:dbl[])  [unwired: 1 out]
                    n779 = Delete From Array(array=w1184, length=w1181, index=w1183) -> (array with subset deleted=w1189:dbl[])  [unwired: 1 out]
                    n780 = Bundle By Name(cluster=w1188, "R"=w1191, "T"=w1190, "Time"=w1189) -> (w1193:cluster{"R":dbl[], "T":dbl[], "Time":dbl[]})
                    n781 = Replace Array Subset(array=w1192, new element=w1193, index=w1197) -> (w1194:T28)
                    n782 = local write "Data Array"(w1194) -> ()
                    n783 = property class="XYGraph (strict)"(reference=w1198, "Active Cursor"=u32 0, "Cursor.Cursor X"=w1178, "Active Cursor"=u32 1, "Cursor.Cursor X"=w1178) -> ()  [unwired: 1 in, 2 out]
                  }
                }
                n784 = local write "_LMBDown"(FALSE ("Mouse down")) -> ()
              }
            }
          }
        }
      }
      event "R-Plot 0", "R-Plot 1", "R-Plot 2", "R-Plot 3", "R-Plot 4", "R-Plot 5", "R-Plot 6", "R-Plot 7", "R-Plot 8", "R-Plot 9": Mouse Leave {
        n785 = event-data() -> ()  [unwired: 1 in, 4 out]
        n786 = local write "_LMBDown"(FALSE ("Mouse down")) -> ()
      }
      event "R-Plot 0", "R-Plot 1", "R-Plot 2", "R-Plot 3", "R-Plot 4", "R-Plot 5", "R-Plot 6", "R-Plot 7", "R-Plot 8", "R-Plot 9": Scale Range Change {
        w1203 = u8 0 ("X Scale.Scale Fit")
        # "Disable plot autoscaling if the user has changed the scale of the plot manualy"
        n787 = event-data() -> ("CtlRef"=w1202:refnum<vi>)  [unwired: 1 in, 7 out]
        n788 = property class="XYGraph (strict)"(reference=w1202, "XScale.ScaleFit"=w1203, "YScale.ScaleFit"=w1203) -> ()  [unwired: 1 in, 2 out]
      }
      event "R-Plot 0", "R-Plot 1", "R-Plot 2", "R-Plot 3", "R-Plot 4", "R-Plot 5", "R-Plot 6", "R-Plot 7", "R-Plot 8", "R-Plot 9": Shortcut Menu Activation? {
        w1212 = string[] ["Log Y"] ("item names")
        w1214 = string[] ["Zoom In to Last Data", "Autoscale XY"] ("item names")
        # "Add extra options to the plots context menu"
        n789 = event-data() -> ("MenuRef"=w1216:refnum<k9>, "CtlRef"=w1208:refnum<vi>)  [unwired: 1 in]
        n790 = Insert Menu Items(4:10, 7:w1214, 8:w1214, 9:w1216) -> (3:w1210:refnum<k9>)  [unwired: 2 in, 2 out]
        n791 = property class="XYGraph (strict)"(reference=w1208) -> ("YScale.Mapping Mode"=w1207:u8)  [unwired: 1 in, 2 out]
        n792 = Insert Menu Items(4:14, 7:w1212, 8:w1212, 9:w1210) -> (3:w1209:refnum<k9>)  [unwired: 2 in, 2 out]
        n793 = Not Equal To 0?(x=w1207) -> (x != 0?=w1206:bool)
        n794 = Set Menu Item Info(6:w1206, 7:"Log Y", 11:w1209) -> ()  [unwired: 4 in, 2 out]
        n795 = local read "_LMBDown"() -> (w1213:bool)
        n796 = event-data("Discard?"=w1213) -> ()  [unwired: 1 in, 1 out]
      }
      event "R-Plot 0", "R-Plot 1", "R-Plot 2", "R-Plot 3", "R-Plot 4", "R-Plot 5", "R-Plot 6", "R-Plot 7", "R-Plot 8", "R-Plot 9": Shortcut Menu Selection (User) {
        # "Zoom in to last \"Miniplot points\". Zoom out a bit to have some space around the points"
        n797 = event-data() -> ("CtlRef"=w1222:refnum<vi>, "ItemTag"=w1220:string)  [unwired: 1 in]
        n798 = Type Cast(type=refnum<vi> refnum ("R-Plot 0"), x=w1222) -> (*(type *) &x=w1221:refnum<vi>)
        n799 = property on="Runtime Settings" class="Clust (strict)"() -> ("Value"=w1218:T27)  [unwired: 2 in, 2 out]
        n800 = case shown="\"Zoom In to Last Data\"" w1220 {
          tunnel: w1221 -> [_ w1224 w1253 w1259]
          tunnel: w1218 -> [_ _ w1225 _]
          frame Default {
          }
          frame "Autoscale XY" {
            w1223 = u8 2 ("X Scale.Scale Fit")
            n801 = property class="XYGraph (strict)"(reference=w1224, "XScale.ScaleFit"=w1223, "YScale.ScaleFit"=w1223) -> ()  [unwired: 1 in, 2 out]
          }
          frame "Zoom In to Last Data" {
            w1249 = u8 0 ("Y Scale.Scale Fit")
            n802 = property class="XYGraph (strict)"(reference=w1253) -> (reference out=w1250:refnum<vi>, "Value"=w1252:cluster{dbl[], dbl[]})  [unwired: 1 in, 1 out]
            n803 = Unbundle By Name(w1225) -> ("Miniplot Time"=w1248:dbl)
            n804 = Unbundle(w1252) -> (w1227:dbl[], w1251:dbl[])
            n805 = Multiply(x=w1248, y=60.0) -> (x*y=w1244:dbl)
            n806 = Reverse 1D Array(array=w1227) -> (reversed array=w1232:dbl[])
            n807 = Reverse 1D Array(array=w1251) -> (reversed array=w1240:dbl[])
            n808 = Index Array(array=w1232) -> (element=w1246:dbl)  [unwired: 1 in]
            n809 = Multiply(x=0.5, y=w1244) -> (x*y=w1245:dbl)
            n810 = Add(x=w1245, y=w1246) -> (x+y=w1243:dbl)
            n811 = Subtract(x=w1246, y=w1244) -> (x-y=w1241:dbl)
            n812 = call "Improved Threshold Detector.71.vi"("Threshold"=w1241, "Array"=w1227) -> ("Positive transition indices"=w1228:i32[])  [unwired: 8 in, 1 out]
            n813 = Index Array(array=w1228) -> (element=w1254:i32)  [unwired: 1 in]
            n814 = Array Size(array=w1227) -> (size(s)=w1230:i32)
            n815 = Index Array(array=w1227, index=w1254) -> (element=w1226:dbl)
            n816 = Subtract(x=w1230, y=w1254) -> (x-y=w1229:i32)
            n817 = Array Subset(array=w1240, length=w1229) -> (w1239:dbl[])  [unwired: 1 in]
            n818 = Array Max & Min(array=w1239) -> (max value=w1236:dbl, min value=w1235:dbl)  [unwired: 2 out]
            n819 = Subtract(x=w1236, y=w1235) -> (x-y=w1238:dbl)
            n820 = Divide(x=w1238, y=2.0) -> (x/y=w1234:dbl)
            n821 = Add(x=w1236, y=w1234) -> (x+y=w1231:dbl)
            n822 = Subtract(x=w1235, y=w1234) -> (x-y=w1233:dbl)
            n823 = property class="XYGraph (strict)"(reference=w1250, "XScale.ScaleFit"=w1249, "YScale.ScaleFit"=w1249, "XScale.Maximum"=w1243, "XScale.Minimum"=w1226, "YScale.Maximum"=w1231, "YScale.Minimum"=w1233) -> ()  [unwired: 1 in, 2 out]
          }
          frame "Log Y" {
            n824 = property class="XYGraph (strict)"(reference=w1259) -> (reference out=w1258:refnum<vi>, "YScale.Mapping Mode"=w1257:u8)  [unwired: 1 in, 1 out]
            n825 = Equal To 0?(x=w1257) -> (x = 0?=w1256:bool)
            n826 = Boolean To (0,1)(Boolean=w1256) -> (0, 1=w1255:i16)
            n827 = property class="XYGraph (strict)"(reference=w1258, "YScale.Mapping Mode"=w1255) -> ()  [unwired: 1 in, 2 out]
          }
        }
      }
      event "uPlots.uPlot 0", "uPlots.uPlot 1", "uPlots.uPlot 2", "uPlots.uPlot 3", "uPlots.uPlot 4", "uPlots.uPlot 5", "uPlots.uPlot 6", "uPlots.uPlot 7", "uPlots.uPlot 8", "uPlots.uPlot 9": Mouse Down {
        # "Switch to big plot on double click on small plot"
        n828 = event-data() -> ("Mods.Double Click"=w1262:bool, "CtlRef"=w1261:refnum<vi>)  [unwired: 1 in]
        n829 = case shown="True" w1262 {
          tunnel: w1261 -> [_ w1265]
          frame False {
          }
          frame True {
            n830 = property class="XYGraph (strict)"(reference=w1265) -> ("Label.Text"=w1266:string)  [unwired: 1 in, 2 out]
            n831 = Reverse String(1:w1266) -> (0:w1267:string)
            n832 = Decimal String To Number(string=w1267, default (0L)=8 ("default (0 I32)")) -> (number=w1264:i32)  [unwired: 1 in, 1 out]
            n833 = property on="Channels Panel" class="TabCtl (strict)"("Val(Sgnl)"=w1264) -> ()  [unwired: 2 in, 2 out]
          }
        }
      }
      event "Erase all": Value Change {
        # "Clear data array.\nReset PID."
        n834 = event-data() -> ()  [unwired: 1 in, 6 out]
        n835 = local read "Channels Panel"() -> (w1271:T8)
        n836 = local read "Data Array"() -> (w1272:T28)
        n837 = Replace Array Subset(array=w1272, new element=cluster{"R":dbl[], "T":dbl[], "Time":dbl[]} {"R"=[], "T"=[], "Time"=[]} ("new element/subarray"), index=w1271) -> (w1270:T28)
        n838 = local write "Data Array"(w1270) -> ()
        n839 = disable-structure shown="Disabled" {
          frame Disabled {
            n840 = Initialize Array(cluster{"R":dbl[], "T":dbl[], "Time":dbl[]} {"R"=[], "T"=[], "Time"=[]}, 10 ("dimension size")) -> ()  [unwired: 1 out]
          }
          frame Enabled {
          }
        }
      }
      event "Clear all plots": Value Change {
        n841 = event-data() -> ()  [unwired: 1 in, 6 out]
        n842 = Initialize Array(cluster{"R":dbl[], "T":dbl[], "Time":dbl[]} {"R"=[], "T"=[], "Time"=[]}, 10 ("dimension size")) -> (w1277:cluster{"R":dbl[], "T":dbl[], "Time":dbl[]}[])
        n843 = local write "Data Array"(w1277) -> ()
      }
      event "Bridge settings.Bridge Type": Value Change {
        # "Select bridge type (AVS/zBridge). Show/hide corresponding controls."
        n844 = event-data() -> ("NewVal"=w1281:T61)  [unwired: 1 in, 5 out]
        n845 = flat-sequence {
          tunnel: w1281 -> [w1290]
          frame #0 {
            w1286 = u8 0 ("Disabled")
            w1289 = u8 0 ("Disabled")
            w1288 = FALSE ("Visible")
            w1287 = u8 2 ("Disabled")
            n846 = property on="AVS RS232 Port" class="VISAName"("Visible"=w1288, "Disabled"=w1287) -> ()  [unwired: 2 in, 2 out]
            n847 = property on="zBridge settings" class="Bool"("Visible"=w1288, "Disabled"=w1287) -> ()  [unwired: 2 in, 2 out]
            n848 = property on="Lower Panel" class="TabCtl (strict)"("Disabled"=w1286) -> ()  [unwired: 2 in, 2 out]
            n849 = property on="AVS GPIB Address" class="VISAName"("Visible"=w1288, "Disabled"=w1287) -> ()  [unwired: 2 in, 2 out]
            n850 = property on="Main Panel" class="TabCtl (strict)"("Disabled"=w1286) -> ()  [unwired: 2 in, 2 out]
            n851 = property on="Read AVS channels from" class="DigNum (strict)"("Disabled"=w1289) -> ()  [unwired: 2 in, 2 out]
            n852 = property on="Last Channel" class="DigNum (strict)"("Disabled"=w1289) -> ()  [unwired: 2 in, 2 out]
            n853 = property on="Stabilisation Delay" class="DigNum (strict)"("Disabled"=w1289) -> ()  [unwired: 2 in, 2 out]
            n854 = property on="Averages" class="DigNum (strict)"("Disabled"=w1289) -> ()  [unwired: 2 in, 2 out]
            n855 = property on="Delay Between Scans" class="DigNum (strict)"("Disabled"=w1289) -> ()  [unwired: 2 in, 2 out]
            n856 = call "Build ranges list.vi"("Values"="-1\r\n0\r\n1\r\n2\r\n3\r\n4\r\n5\r\n6\r\n7", "Strings"="n.a.\r\nopen\r\n2 Ohm\r\n20 Ohm\r\n200 Ohm\r\n2k Ohm\r\n20k Ohm\r\n200k Ohm\r\n2M Ohm") -> ("Strings and Values"=w1285:cluster{"String":string, "Value":i32}[])  [unwired: 4 in]
            n857 = property on="Range 0" class="Ring (strict)"("StringsAndValues[]"=w1285) -> ()  [unwired: 2 in, 2 out]
            n858 = property on="Range 1" class="Ring (strict)"("StringsAndValues[]"=w1285) -> ()  [unwired: 2 in, 2 out]
            n859 = property on="Range 2" class="Ring (strict)"("StringsAndValues[]"=w1285) -> ()  [unwired: 2 in, 2 out]
            n860 = property on="Range 3" class="Ring (strict)"("StringsAndValues[]"=w1285) -> ()  [unwired: 2 in, 2 out]
            n861 = property on="Range 4" class="Ring (strict)"("StringsAndValues[]"=w1285) -> ()  [unwired: 2 in, 2 out]
            n862 = property on="Range 5" class="Ring (strict)"("StringsAndValues[]"=w1285) -> ()  [unwired: 2 in, 2 out]
            n863 = property on="Range 6" class="Ring (strict)"("StringsAndValues[]"=w1285) -> ()  [unwired: 2 in, 2 out]
            n864 = property on="Range 7" class="Ring (strict)"("StringsAndValues[]"=w1285) -> ()  [unwired: 2 in, 2 out]
          }
          frame #1 {
            n865 = case shown="\"AVS48SI (RS232 interface)\"" w1290 {
              frame "AVS47A (GPIB interface)" {
                n866 = local write "AVS Scan Parameters"(enum32{"Page 1", "Page 2"}."Page 1" ("Scan Parameters")) -> ()
                n867 = property on="AVS GPIB Address" class="VISAName"("Visible"=TRUE, "Disabled"=u8 0) -> ()  [unwired: 2 in, 2 out]
              }
              frame "AVS47B (RS232 interface)" {
                w1294 = u8 2 ("Disabled")
                n868 = local write "AVS Scan Parameters"(enum32{"Page 1", "Page 2"}."Page 1" ("Scan Parameters")) -> ()
                n869 = property on="AVS RS232 Port" class="VISAName"("Visible"=TRUE, "Disabled"=u8 0) -> ()  [unwired: 2 in, 2 out]
                n870 = property on="Read AVS channels from" class="DigNum (strict)"("Disabled"=w1294) -> ()  [unwired: 2 in, 2 out]
                n871 = property on="Last Channel" class="DigNum (strict)"("Disabled"=w1294) -> ()  [unwired: 2 in, 2 out]
              }
              frame "AVS48SI (RS232 interface)" {
                w1301 = u8 2 ("Disabled")
                n872 = property on="Read AVS channels from" class="DigNum (strict)"("Disabled"=w1301) -> ()  [unwired: 2 in, 2 out]
                n873 = property on="Last Channel" class="DigNum (strict)"("Disabled"=w1301) -> ()  [unwired: 2 in, 2 out]
                n874 = property on="AVS RS232 Port" class="VISAName"("Visible"=TRUE, "Disabled"=u8 0) -> ()  [unwired: 2 in, 2 out]
                n875 = local write "AVS Scan Parameters"(enum32{"Page 1", "Page 2"}."Page 1" ("Scan Parameters")) -> ()
                n876 = call "Build ranges list.vi"("Values"="-1\r\n0\r\n1\r\n2\r\n3\r\n4\r\n5\r\n6\r\n7", "Strings"="n.a.\r\n3 Ohm\r\n30 Ohm\r\n300 Ohm\r\n3k Ohm\r\n30k Ohm\r\n300k Ohm\r\n3M Ohm\r\n30m Ohm") -> ("Strings and Values"=w1299:cluster{"String":string, "Value":i32}[])  [unwired: 4 in]
                n877 = property on="Range 0" class="Ring (strict)"("StringsAndValues[]"=w1299) -> ()  [unwired: 2 in, 2 out]
                n878 = property on="Range 1" class="Ring (strict)"("StringsAndValues[]"=w1299) -> ()  [unwired: 2 in, 2 out]
                n879 = property on="Range 2" class="Ring (strict)"("StringsAndValues[]"=w1299) -> ()  [unwired: 2 in, 2 out]
                n880 = property on="Range 3" class="Ring (strict)"("StringsAndValues[]"=w1299) -> ()  [unwired: 2 in, 2 out]
                n881 = property on="Range 4" class="Ring (strict)"("StringsAndValues[]"=w1299) -> ()  [unwired: 2 in, 2 out]
                n882 = property on="Range 5" class="Ring (strict)"("StringsAndValues[]"=w1299) -> ()  [unwired: 2 in, 2 out]
                n883 = property on="Range 6" class="Ring (strict)"("StringsAndValues[]"=w1299) -> ()  [unwired: 2 in, 2 out]
                n884 = property on="Range 7" class="Ring (strict)"("StringsAndValues[]"=w1299) -> ()  [unwired: 2 in, 2 out]
              }
              frame "AVS Emulation" {
                n885 = local write "AVS Scan Parameters"(enum32{"Page 1", "Page 2"}."Page 1" ("Scan Parameters")) -> ()
              }
              frame "Impedance Bridge" {
                w1308 = u8 2 ("Disabled")
                n886 = local write "AVS Scan Parameters"(enum32{"Page 1", "Page 2"}."Page 2" ("Scan Parameters")) -> ()
                n887 = property on="zBridge settings" class="Bool"("Visible"=TRUE, "Disabled"=u8 0) -> ()  [unwired: 2 in, 2 out]
                n888 = property on="Read AVS channels from" class="DigNum (strict)"("Disabled"=w1308) -> ()  [unwired: 2 in, 2 out]
                n889 = property on="Last Channel" class="DigNum (strict)"("Disabled"=w1308) -> ()  [unwired: 2 in, 2 out]
                n890 = property on="Stabilisation Delay" class="DigNum (strict)"("Disabled"=w1308) -> ()  [unwired: 2 in, 2 out]
                n891 = property on="Averages" class="DigNum (strict)"("Disabled"=w1308) -> ()  [unwired: 2 in, 2 out]
                n892 = property on="Delay Between Scans" class="DigNum (strict)"("Disabled"=w1308) -> ()  [unwired: 2 in, 2 out]
              }
              frame "Disabled", Default {
                w1310 = u8 2 ("Disabled")
                n893 = property on="Lower Panel" class="TabCtl (strict)"("Disabled"=w1310) -> ()  [unwired: 2 in, 2 out]
                n894 = property on="Main Panel" class="TabCtl (strict)"("Disabled"=w1310) -> ()  [unwired: 2 in, 2 out]
              }
            }
          }
        }
      }
      event "Runtime Settings.Plot type": Value Change {
        # "Iterate through first 10 pages (plots only)"
        # "Switch between RxTime and TxTime plots"
        n895 = event-data() -> ("NewVal"=w1321:enum16{"R vs Time", "T vs Time"})  [unwired: 1 in, 5 out]
        n896 = Unbundle By Name(w1313) -> ("Reset PID loop"=w1312:refnum<user-event>)
        n897 = Equal To 0?(x=w1321) -> (x = 0?=w1320:bool)
        n898 = Select(t=u32 10532351, s=w1320, f=u32 16711680) -> (s? t:f=w1317:u32)
        n899 = property on="uPlots" class="Clust (strict)"() -> ("Controls[]"=w1315:refnum<vi>[])  [unwired: 2 in, 2 out]
        n900 = property on="Channels Panel" class="TabCtl (strict)"() -> ("Pages"=w1322:refnum<vi>[])  [unwired: 2 in, 2 out]
        n901 = for {
          N: 10 -> [_]
          tunnel: w1322 -> [w1332] mode=indexing
          tunnel: w1317 -> [w1325]
          tunnel: w1315 -> [w1323] mode=indexing
          # "!!NOTE:This routine assumes that graph is control #0 on page!!"
          n902 = property class="Page"(reference=w1332) -> ("ControlsOnPage"=w1330:refnum<vi>[])  [unwired: 1 in, 2 out]
          n903 = Type Cast(type=refnum<vi> refnum ("R-Plot 0"), x=w1323) -> (*(type *) &x=w1324:refnum<vi>)
          n904 = Index Array(array=w1330, index=0) -> (element=w1328:refnum<vi>)
          n905 = Type Cast(type=refnum<vi> refnum ("R-Plot 0"), x=w1328) -> (*(type *) &x=w1327:refnum<vi>)
          n906 = property class="XYGraph (strict)"(reference=w1327, "Plot.Plot Color"=w1325, "Plot.Fill/Pt. Color"=w1325) -> ()  [unwired: 1 in, 2 out]
          n907 = property class="XYGraph (strict)"(reference=w1324, "Plot.Plot Color"=w1325, "Plot.Fill/Pt. Color"=w1325) -> ()  [unwired: 1 in, 2 out]
        }
        n908 = Generate User Event(user event=w1312, event data cluster="" ("event data")) -> ()  [unwired: 2 in, 2 out]
      }
      event "Runtime Settings.Read AVS channels from", "Runtime Settings.Last Channel": Value Change {
        # "Change enabled channels for the AVS bridge"
        n909 = event-data() -> ()  [unwired: 1 in, 6 out]
        n910 = Unbundle By Name(w1335) -> ("UpdateChannelInfo"=w1334:refnum<user-event>)
        n911 = Generate User Event(user event=w1334, event data cluster=bool[] [] ("event data")) -> ()  [unwired: 2 in, 2 out]
      }
      event "Runtime Settings.Filter Graphs": Value Change {
        # "Graph filtering controls"
        n912 = event-data() -> ("NewVal"=w1338:bool)  [unwired: 1 in, 5 out]
        n913 = call "IsDisabled.vi"("Enabled?"=w1338) -> ("Numeric"=w1339:i16)
        n914 = property on="Y_min" class="DigNum (strict)"("Disabled"=w1339) -> ()  [unwired: 2 in, 2 out]
        n915 = property on="Y_max" class="DigNum (strict)"("Disabled"=w1339) -> ()  [unwired: 2 in, 2 out]
      }
      event "Channels Panel": Value Change {
        # "Show hide bottom Impedance/Temperature panel depending on the current tab page"
        n916 = event-data() -> ("NewVal"=w1342:T8)  [unwired: 1 in, 5 out]
        n917 = case shown="Default" w1342 {
          tunnel: [TRUE ("Visible") FALSE ("Visible")] -> w1341
          frame Default {
            n918 = property on="Mode Buttons" class="RadioBtnsControl (strict)"() -> ("Value"=w1344:T7)  [unwired: 2 in, 2 out]
            n919 = property on="Data History/RT Settings" class="TabCtl (strict)"("Value"=enum32{"History", "Settings"}."History" ("Data History")) -> ()  [unwired: 2 in, 2 out]
            n920 = property on="Mode Buttons" class="RadioBtnsControl (strict)"("Val(Sgnl)"=w1344) -> ()  [unwired: 2 in, 2 out]
          }
          frame "All", "PID loop" {
            n921 = property on="Data History/RT Settings" class="TabCtl (strict)"("Value"=enum32{"History", "Settings"}."Settings" ("Data History")) -> ()  [unwired: 2 in, 2 out]
          }
        }
        n922 = property on="Graph Controls Bar" class="TabCtl (strict)"("Visible"=w1341) -> ()  [unwired: 2 in, 2 out]
      }
      event Value Change {
        # "Calibration changed - update calibrations list"
        n923 = event-data() -> ()  [unwired: 1 in, 6 out]
        n924 = property on="Sensor Calibrations" class="Clust (strict)"() -> ("Controls[]"=w1351:refnum<vi>[])  [unwired: 2 in, 2 out]
        n925 = Array Size(array=w1351) -> (size(s)=w1352:i32)
        n926 = for {
          N: w1352 -> [_]
          tunnel: w1351 -> [w1356] mode=indexing
          tunnel: [w1353] -> w1350 mode=indexing
          w1355 = refnum<vi> refnum  # Ring
          n927 = Type Cast(type=w1355, x=w1356) -> (*(type *) &x=w1354:refnum<vi>)
          n928 = property class="Ring"(reference=w1354) -> ("RingText.Text"=w1353:string)  [unwired: 1 in, 2 out]
        }
        n929 = Array To Cluster(array=w1350) -> (cluster=→"_CurCalibrations":T33)
      }
      event "Data Logging Settings": Value Change {
        # "Log file settings changed. Generate new log file name"
        n930 = event-data() -> ()  [unwired: 1 in, 3 out]
        n931 = local read "Data Logging Settings"() -> (w1365:T37)
        n932 = Unbundle By Name(w1365) -> ("Run Description"=w1359:string, "Filenames Suffix"=w1360:string, "Log Files Folder"=w1366:path, "Log Files Name"=w1364:string, "Automode Files Name"=w1363:string)
        n933 = call "MGI Make String Filesafe.vi"("String In"=w1359) -> ("Filesafe String Out"=w1358:string)
        n934 = call "GeneratePaths.vi"("Filename Suffix"=w1360, "Run description"=w1358, "AVS_Path"=w1366, "AVS_FName"=w1364, "CAL_Path"=w1366, "CAL_FName"=w1363) -> ("Generated Log path"=w1362:path, "Generated Calib path"=w1361:path)  [unwired: 8 in]
        n935 = local write "_LogFilesPath"(w1362) -> ()
        n936 = local write "_CalibFilesPath"(w1361) -> ()
      }
      event "Convert R-T": Mouse Down; "QuickR": Value Change {
        # "Quick convert R->T"
        n937 = event-data() -> ()  [unwired: 1 in, 4 out]
        n938 = Unbundle By Name(w1367) -> ("Calibrations Folder"=w1368:path)
        n939 = property on="_QuickConvertCal" class="Ring (strict)"() -> ("Strings []"=w1371:string[], "Value"=w1372:u16)  [unwired: 2 in, 2 out]
        n940 = Index Array(array=w1371, index=w1372) -> (element=w1370:string)
        n941 = call "SelectSensor-txt no ext.vi"("Path"=w1368, "Resistance"="QuickR", "Select sensor"=w1370) -> ("error out"=w1369:errorcluster, "Temperature"=→"T7":dbl)
      }
      event "T Sweep.Current": Value Change {
        # "Current/ Setpoint value is changed"
        n942 = event-data() -> ("NewVal"=→"_I3SetPnt":dbl)  [unwired: 1 in, 5 out]
        n943 = Unbundle By Name(w1377) -> ("Reset PID loop"=w1376:refnum<user-event>)
        n944 = Generate User Event(user event=w1376, event data cluster="" ("event data")) -> ()  [unwired: 2 in, 2 out]
      }
      event Value Change {
        w1381 = FALSE ("Value (Signaling)")
        # "Changed Channel1 automatic mode"
        n945 = event-data() -> ("NewVal"=w1383:T39)  [unwired: 1 in, 5 out]
        n946 = Unbundle By Name(w1385) -> ("TempStabilized"=w1384:refnum<user-event>)
        n947 = property on="CS.Mode1.Start" class="Bool (strict)"("Val(Sgnl)"=w1381) -> ()  [unwired: 2 in, 2 out]
        n948 = property on="CS.Mode2.Start" class="Bool (strict)"("Val(Sgnl)"=w1381) -> ()  [unwired: 2 in, 2 out]
        n949 = case shown="\"Mode 1\"" w1383 {
          tunnel: [FALSE ("Automatic mode ON") TRUE ("Automatic mode ON") TRUE ("Automatic mode ON")] -> w1386
          tunnel: w1384 -> [_ w1396 _]
          tunnel: [0 1 2] -> w1382
          frame "Manual" {
            # "Set manual mode currents \nequal to last automode \nvalues."
            n950 = local read "CS.Automode Current"() -> (w1389:T23[])
            n951 = Index Array(array=w1389) -> (element #1=w1393:T23, element #2=w1392:T23, element #3=w1391:T23, element #4=w1390:T23)  [unwired: 4 in]
            n952 = property on="I" class="DigNum (strict)"("Val(Sgnl)"=w1393) -> ()  [unwired: 2 in, 2 out]
            n953 = property on="I" class="DigNum (strict)"("Val(Sgnl)"=w1392) -> ()  [unwired: 2 in, 2 out]
            n954 = property on="I" class="DigNum (strict)"("Val(Sgnl)"=w1391) -> ()  [unwired: 2 in, 2 out]
            n955 = property on="I" class="DigNum (strict)"("Val(Sgnl)"=w1390) -> ()  [unwired: 2 in, 2 out]
          }
          frame "Mode 1" {
            # "Set automatic mode currents equal to last manual values."
            n956 = local read "CS.Current Value"() -> (w1399:dbl[])
            n957 = Multiply(x=1000.0, y=w1399) -> (x*y=w1397:dbl[])
            n958 = local write "CS.Automode Current"(w1397) -> ()
            n959 = Generate User Event(user event=w1396, event data cluster=FALSE ("event data")) -> ()  [unwired: 2 in, 2 out]
          }
          frame "Mode2" {
            # "Set automatic mode currents equal to last manual values."
            n960 = local read "CS.Current Value"() -> (w1404:dbl[])
            n961 = Multiply(x=1000.0, y=w1404) -> (x*y=w1402:dbl[])
            n962 = local write "CS.Automode Current"(w1402) -> ()
          }
        }
        "CS.Automode 1" <- w1386
        "CS.Automode 2" <- w1386
        "CS.Automode 3" <- w1386
        "CS.Automode 0" <- w1386
        n963 = property on="CS Modes Panel" class="TabCtl (strict)"("Value"=w1382) -> ()  [unwired: 2 in, 2 out]
      }
      event "Data Logging Settings.External VI Path": Value Change {
        # "Set path for the external VI to call on TempStabilised event"
        n964 = event-data() -> ("NewVal"=w1409:path)  [unwired: 1 in, 5 out]
        n965 = vi-ref "OnTempStabilizedRef.vi"() -> (w1410:refnum<vi>)
        n966 = Open VI Reference(type specifier VI Refnum (for type only)=w1410, vi path=w1409) -> (vi reference=w1408:refnum<vi>)  [unwired: 4 in, 1 out]
        n967 = local write "_ExtVIReference"(w1408) -> ()
      }
      event "CS Settings.CS type": Value Change {
        # "Set CS type"
        n968 = event-data() -> ("NewVal"=w1412:T57)  [unwired: 1 in, 5 out]
        n969 = flat-sequence {
          tunnel: w1412 -> [w1439]
          frame #0 {
            w1424 = u8 2 ("Disabled")
            w1419 = u8 0 ("Disabled")
            w1434 = TRUE ("Visible")
            n970 = control-ref of="CS Indicators Panel"() -> (w1420:refnum<vi>)
            n971 = control-ref of="I0"() -> (w1431:refnum<vi>)
            n972 = control-ref of="I1"() -> (w1423:refnum<vi>)
            n973 = control-ref of="CS.I0"() -> (w1430:refnum<vi>)
            n974 = control-ref of="CS.I1"() -> (w1422:refnum<vi>)
            n975 = control-ref of="I2"() -> (w1418:refnum<vi>)
            n976 = control-ref of="I3"() -> (w1417:refnum<vi>)
            n977 = control-ref of="CS Mode"() -> (w1421:refnum<vi>)
            n978 = control-ref of="QCS. I0 Mapping"() -> (w1429:refnum<vi>)
            n979 = property class="TabCtl (strict)"(reference=w1420, "Disabled"=w1419) -> ()  [unwired: 1 in, 2 out]
            n980 = property class="Clust (strict)"(reference=w1431, "Disabled"=w1419) -> ()  [unwired: 1 in, 2 out]
            n981 = property class="Clust (strict)"(reference=w1423, "Disabled"=w1419) -> ()  [unwired: 1 in, 2 out]
            n982 = property class="Clust (strict)"(reference=w1418, "Disabled"=w1419) -> ()  [unwired: 1 in, 2 out]
            n983 = property class="Clust (strict)"(reference=w1417, "Disabled"=w1419) -> ()  [unwired: 1 in, 2 out]
            n984 = property class="Clust (strict)"(reference=w1430, "Disabled"=w1419) -> ()  [unwired: 1 in, 2 out]
            n985 = property class="Clust (strict)"(reference=w1422, "Disabled"=w1419) -> ()  [unwired: 1 in, 2 out]
            n986 = property class="Enum (strict)"(reference=w1429, "Disabled"=w1419) -> ()  [unwired: 1 in, 2 out]
            n987 = property class="Enum (strict)"(reference=w1421, "Disabled"=w1419) -> ()  [unwired: 1 in, 2 out]
            n988 = property on="Side Panel" class="TabCtl (strict)"() -> ("Pages"=w1413:refnum<vi>[])  [unwired: 2 in, 2 out]
            n989 = control-ref of="TCS RS232 Port"() -> (w1433:refnum<vi>)
            n990 = Index Array(array=w1413, index=1) -> (element=w1414:refnum<vi>)
            n991 = control-ref of="Toggle Gated"() -> (w1425:refnum<vi>)
            n992 = control-ref of="Toggle Gated"() -> (w1426:refnum<vi>)
            n993 = control-ref of="Toggle Gated"() -> (w1427:refnum<vi>)
            n994 = control-ref of="Toggle Gated"() -> (w1428:refnum<vi>)
            n995 = control-ref of="CS.QCS Device Nr"() -> (w1436:refnum<vi>)
            n996 = control-ref of="CS.QCS I0 Output"() -> (w1435:refnum<vi>)
            n997 = property class="Page"(reference=w1414, "PageVis"=TRUE ("Page Visible")) -> ()  [unwired: 1 in, 2 out]
            n998 = property class="Bool (strict)"(reference=w1425, "Disabled"=w1424) -> ()  [unwired: 1 in, 2 out]
            n999 = property class="Bool (strict)"(reference=w1426, "Disabled"=w1424) -> ()  [unwired: 1 in, 2 out]
            n1000 = property class="Bool (strict)"(reference=w1427, "Disabled"=w1424) -> ()  [unwired: 1 in, 2 out]
            n1001 = property class="Bool (strict)"(reference=w1428, "Disabled"=w1424) -> ()  [unwired: 1 in, 2 out]
            n1002 = property class="DigNum (strict)"(reference=w1436, "Visible"=w1434) -> ()  [unwired: 1 in, 2 out]
            n1003 = property class="Enum (strict)"(reference=w1435, "Visible"=w1434) -> ()  [unwired: 1 in, 2 out]
            n1004 = property class="VISAName"(reference=w1433, "Visible"=FALSE) -> ()  [unwired: 1 in, 2 out]
          }
          frame #1 {
            n1005 = case shown="\"PCS (n.a.)\"" w1439 {
              tunnel: [refnum<class "TCS.lvclass"> refnum ("TCS.lvclass") refnum<class "QCS.lvclass"> refnum ("QCS.lvclass") w1459 w1473 refnum<class "PCS.lvclass"> refnum ("PCS.lvclass")] -> w1438
              tunnel: [w1440 w1458 u16 255 ("Value") u16 255 ("Value") w1478] -> w1437
              frame "TCS" {
                w1443 = u8 2 ("Disabled")
                w1456 = u8 0 ("Disabled")
                n1006 = control-ref of="TCS RS232 Port"() -> (w1446:refnum<vi>)
                n1007 = control-ref of="Toggle Gated"() -> (w1455:refnum<vi>)
                n1008 = control-ref of="Toggle Gated"() -> (w1454:refnum<vi>)
                n1009 = control-ref of="Toggle Gated"() -> (w1453:refnum<vi>)
                n1010 = control-ref of="Toggle Gated"() -> (w1452:refnum<vi>)
                n1011 = control-ref of="CS.QCS Device Nr"() -> (w1448:refnum<vi>)
                n1012 = control-ref of="I0"() -> (w1451:refnum<vi>)
                n1013 = control-ref of="CS.I0"() -> (w1444:refnum<vi>)
                n1014 = control-ref of="QCS. I0 Mapping"() -> (w1445:refnum<vi>)
                n1015 = property class="Bool (strict)"(reference=w1455, "Disabled"=w1456) -> ()  [unwired: 1 in, 2 out]
                n1016 = property class="Bool (strict)"(reference=w1454, "Disabled"=w1456) -> ()  [unwired: 1 in, 2 out]
                n1017 = property class="Bool (strict)"(reference=w1453, "Disabled"=w1456) -> ()  [unwired: 1 in, 2 out]
                n1018 = property class="Bool (strict)"(reference=w1452, "Disabled"=w1456) -> ()  [unwired: 1 in, 2 out]
                n1019 = property class="Clust (strict)"(reference=w1444, "Disabled"=w1443) -> ()  [unwired: 1 in, 2 out]
                n1020 = property class="Clust (strict)"(reference=w1451, "Disabled"=u8 2) -> ()  [unwired: 1 in, 2 out]
                n1021 = property class="DigNum (strict)"(reference=w1448, "Visible"=FALSE) -> ()  [unwired: 1 in, 2 out]
                n1022 = property class="VISAName"(reference=w1446, "Visible"=TRUE) -> ()  [unwired: 1 in, 2 out]
                n1023 = property class="Enum (strict)"(reference=w1445, "Disabled"=w1443) -> ()  [unwired: 1 in, 2 out]
                n1024 = property on="TCS RS232 Port" class="VISAName"() -> ("Value"=w1441:refnum<visa-resource-name>)  [unwired: 2 in, 2 out]
                n1025 = call "VISA to RS232 Port Nr.vi"("VISA Resource Name"=w1441) -> ("Port Number"=w1440:u8)  [unwired: 1 in]
              }
              frame "QCS v1" {
                n1026 = property on="CS.QCS Device Nr" class="DigNum (strict)"() -> ("Value"=w1458:u16)  [unwired: 2 in, 2 out]
              }
              frame "CS Emulation" {
                w1459 = refnum<class "CS Emulation.lvclass"> refnum  # CS Emulation.lvclass
                n1027 = control-ref of="CS.QCS Device Nr"() -> (w1462:refnum<vi>)
                n1028 = property class="DigNum (strict)"(reference=w1462, "Visible"=FALSE) -> ()  [unwired: 1 in, 2 out]
              }
              frame "Disabled", Default {
                w1463 = u8 2 ("Disabled")
                w1473 = refnum<class "CS Emulation.lvclass"> refnum  # CS Emulation.lvclass
                n1029 = control-ref of="CS Indicators Panel"() -> (w1472:refnum<vi>)
                n1030 = control-ref of="I0"() -> (w1467:refnum<vi>)
                n1031 = control-ref of="I1"() -> (w1466:refnum<vi>)
                n1032 = control-ref of="I2"() -> (w1465:refnum<vi>)
                n1033 = control-ref of="I3"() -> (w1464:refnum<vi>)
                n1034 = control-ref of="CS.QCS Device Nr"() -> (w1476:refnum<vi>)
                n1035 = property class="DigNum (strict)"(reference=w1476, "Visible"=FALSE) -> ()  [unwired: 1 in, 2 out]
                n1036 = property class="Clust (strict)"(reference=w1467, "Disabled"=w1463) -> ()  [unwired: 1 in, 2 out]
                n1037 = property class="Clust (strict)"(reference=w1466, "Disabled"=w1463) -> ()  [unwired: 1 in, 2 out]
                n1038 = property class="Clust (strict)"(reference=w1465, "Disabled"=w1463) -> ()  [unwired: 1 in, 2 out]
                n1039 = property class="Clust (strict)"(reference=w1464, "Disabled"=w1463) -> ()  [unwired: 1 in, 2 out]
                n1040 = property class="TabCtl (strict)"(reference=w1472, "Disabled"=w1463) -> ()  [unwired: 1 in, 2 out]
                n1041 = property on="Side Panel" class="TabCtl (strict)"() -> ("Pages"=w1471:refnum<vi>[])  [unwired: 2 in, 2 out]
                n1042 = Index Array(array=w1471, index=1) -> (element=w1470:refnum<vi>)
                n1043 = property class="Page"(reference=w1470, "PageVis"=FALSE ("Page Visible")) -> ()  [unwired: 1 in, 2 out]
              }
              frame "PCS (n.a.)" {
                w1479 = u8 2 ("Disabled")
                n1044 = control-ref of="I0"() -> (w1485:refnum<vi>)
                n1045 = control-ref of="I1"() -> (w1484:refnum<vi>)
                n1046 = control-ref of="CS.I0"() -> (w1483:refnum<vi>)
                n1047 = control-ref of="CS.I1"() -> (w1482:refnum<vi>)
                n1048 = control-ref of="CS Mode"() -> (w1481:refnum<vi>)
                n1049 = control-ref of="QCS. I0 Mapping"() -> (w1480:refnum<vi>)
                n1050 = property class="Clust (strict)"(reference=w1483, "Disabled"=w1479) -> ()  [unwired: 1 in, 2 out]
                n1051 = property class="Clust (strict)"(reference=w1482, "Disabled"=w1479) -> ()  [unwired: 1 in, 2 out]
                n1052 = property class="Clust (strict)"(reference=w1485, "Disabled"=w1479) -> ()  [unwired: 1 in, 2 out]
                n1053 = property class="Clust (strict)"(reference=w1484, "Disabled"=w1479) -> ()  [unwired: 1 in, 2 out]
                n1054 = property class="Enum (strict)"(reference=w1481, "Disabled"=w1479) -> ()  [unwired: 1 in, 2 out]
                n1055 = property class="Enum (strict)"(reference=w1480, "Disabled"=w1479) -> ()  [unwired: 1 in, 2 out]
                n1056 = property on="CS.QCS Device Nr" class="DigNum (strict)"() -> ("Value"=w1478:u16)  [unwired: 2 in, 2 out]
              }
            }
            "_CSClassRef" <- w1438
            n1057 = property on="_CS_Address" class="DigNum (strict)"("Value"=w1437) -> ()  [unwired: 2 in, 2 out]
          }
        }
      }
      event "CS Settings.CS.QCS Device Nr": Value Change {
        # "Set CS port"
        n1058 = event-data() -> ("NewVal"=w1487:u16)  [unwired: 1 in, 5 out]
        n1059 = property on="CS type" class="Enum (strict)"() -> ("Value"=w1488:T57)  [unwired: 2 in, 2 out]
        n1060 = case shown="Default" w1488 {
          tunnel: w1487 -> [_ w1491 _]
          frame Default {
          }
          frame "QCS v1" {
            n1061 = Variant To Data(type=u32 255 ("HW Address"), Variant=w1491) -> (data=w1489:u32)  [unwired: 1 in, 1 out]
            n1062 = property on="_CS_Address" class="DigNum (strict)"("Value"=w1489) -> ()  [unwired: 2 in, 2 out]
          }
          frame "CS Emulation" {
            n1063 = property on="_CS_Address" class="DigNum (strict)"("Value"=u32 255 ("HW Address")) -> ()  [unwired: 2 in, 2 out]
          }
        }
      }
      event "CS Settings.TCS RS232 Port": Value Change {
        # "Set TCS port"
        n1064 = event-data() -> ("NewVal"=w1494:refnum<visa-resource-name>)  [unwired: 1 in, 5 out]
        n1065 = property on="CS type" class="Enum (strict)"() -> ("Value"=w1495:T57)  [unwired: 2 in, 2 out]
        n1066 = case shown="\"TCS\"" w1495 {
          tunnel: w1494 -> [w1498 _]
          frame "TCS" {
            n1067 = Type Cast(type=refnum<visa-resource-name> refnum ("Value"), x=w1498) -> (*(type *) &x=w1497:refnum<visa-resource-name>)
            n1068 = call "VISA to RS232 Port Nr.vi"("VISA Resource Name"=w1497) -> ("Port Number"=w1499:u8)  [unwired: 1 in]
            n1069 = property on="_CS_Address" class="DigNum (strict)"("Value"=w1499) -> ()  [unwired: 2 in, 2 out]
          }
          frame Default {
          }
        }
      }
      event "Load Data": Value Change {
        # "Load data from log files"
        n1070 = event-data() -> ()  [unwired: 1 in, 6 out]
        n1071 = property on="Log Files Folder" class="Path"() -> ("Value"=w1503:path)  [unwired: 2 in, 2 out]
        n1072 = call "File Dialog4"("start path"=w1503) -> ("selected paths"=w1502:path[], "cancelled"=w1501:bool)  [unwired: 11 in, 2 out]
        n1073 = case shown="False" w1501 {
          tunnel: w1502 -> [w1517 _]
          frame False {
            n1074 = property on="Bridge Type" class="Enum (strict)"() -> ("Value"=w1507:T61)  [unwired: 2 in, 2 out]
            n1075 = case shown="Default" w1507 {
              tunnel: [2 ("index")] -> w1506
              tunnel: [10 ("length")] -> w1504
              tunnel: [12 ("index")] -> w1505
              frame Default {
              }
            }
            n1076 = for {
              tunnel: w1517 -> [w1541] mode=indexing
              shift-right: [w1539] -> w1514
              shift-left: string[][] [] ("all rows") -> [w1540]
              # "skip header"
              n1077 = call <vilib>:"Read From Spreadsheet File (string).vi"("file path (dialog if empty)"=w1541) -> ("all rows"=w1537:string[][])  [unwired: 6 in, 4 out]
              n1078 = Array Subset(array=w1537, index (row)=5 ("index")) -> (w1536:string[][])  [unwired: 3 in]
              n1079 = Insert Into Array(array=w1540, new element=w1536) -> (w1539:string[][])  [unwired: 2 in]
            }
            n1080 = Index Array(array=w1514, index (col)=1 ("disabled index (col)")) -> (element=w1511:string[])  [unwired: 1 in]
            n1081 = Array Subset(array=w1514, index (col)=w1506, length (col)=w1504) -> (w1513:string[][])  [unwired: 2 in]
            n1082 = Array Subset(array=w1514, index (col)=w1505, length (col)=w1504) -> (w1512:string[][])  [unwired: 2 in]
            n1083 = Transpose 2D Array(2D array=w1513) -> (transposed array=w1509:string[][])
            n1084 = Transpose 2D Array(2D array=w1512) -> (transposed array=w1508:string[][])
            n1085 = for {
              tunnel: w1509 -> [w1533] mode=indexing
              tunnel: w1508 -> [w1532] mode=indexing
              tunnel: w1511 -> [w1534]
              tunnel: [w1531] -> w1510 mode=indexing
              # "Sort data by date and remove duplicate points"
              n1086 = Fract/Exp String To Number(string=w1533) -> (number=w1528:dbl[])  [unwired: 3 in, 1 out]
              n1087 = Fract/Exp String To Number(string=w1534) -> (number=w1530:dbl[])  [unwired: 3 in, 1 out]
              n1088 = Fract/Exp String To Number(string=w1532) -> (number=w1529:dbl[])  [unwired: 3 in, 1 out]
              n1089 = call "Sort 1D Array (DBL)__ogtk.vi"("Array in"=w1530) -> ("Sorted Pointers"=w1535:i32[], "Sorted Array out"=w1523:dbl[])  [unwired: 9 in]
              n1090 = call "Reorder 1D Array2 (DBL)__ogtk.vi"("indices"=w1535, "array"=w1528) -> ("reordered array"=w1527:dbl[])  [unwired: 9 in]
              n1091 = call "Reorder 1D Array2 (DBL)__ogtk.vi"("indices"=w1535, "array"=w1529) -> ("reordered array"=w1525:dbl[])  [unwired: 9 in]
              n1092 = call "Remove Duplicates from 1D Array (DBL)__ogtk.vi"("Input Array"=w1527) -> ("Output Array"=w1526:dbl[], "indices of removed elements"=w1521:i32[])
              n1093 = call "Delete Elements from 1D Array (DBL)__ogtk.vi"("indices"=w1521, "array"=w1525) -> ("array w/ subset deleted"=w1524:dbl[])  [unwired: 8 in, 1 out]
              n1094 = call "Delete Elements from 1D Array (DBL)__ogtk.vi"("indices"=w1521, "array"=w1523) -> ("array w/ subset deleted"=w1522:dbl[])  [unwired: 8 in, 1 out]
              n1095 = Bundle("Output Array"=w1526, "array w/ subset deleted"=w1524, "array w/ subset deleted"=w1522) -> (w1531:T72)  [unwired: 1 in]
            }
            n1096 = local write "Data Array"(w1510) -> ()
          }
          frame True {
          }
        }
      }
      event "Save Data 2": Value Change {
        # "Load data from log files"
        n1097 = event-data() -> ()  [unwired: 1 in, 6 out]
        n1098 = property on="Log Files Folder" class="Path"() -> ("Value"=w1547:path)  [unwired: 2 in, 2 out]
        n1099 = call "File Dialog"("start path"=w1547, "pattern (all files)"="*.dat", "pattern label"="Log files") -> ("selected path"=w1545:path, "cancelled"=w1546:bool)  [unwired: 9 in, 2 out]
        n1100 = case shown="False" w1546 {
          tunnel: w1545 -> [w1552 _]
          frame False {
            (unwired) 30 ("dimension size")
            n1101 = local read "Data Array"() -> (w1553:T28)
            n1102 = for {
              tunnel: w1553 -> [w1566] mode=indexing
              tunnel: [w1557] -> w1551 mode=indexing
              shift-right: [w1555] -> w1549
              shift-left: string[][] [] -> [w1556]
              n1103 = Unbundle By Name(w1566) -> ("Time"=w1563:dbl[], "R"=w1562:dbl[], "T"=w1558:dbl[])
              n1104 = property on="Data Logging Settings" class="Clust (strict)"() -> ("Value"=w1565:T37)  [unwired: 2 in, 2 out]
              n1105 = Unbundle By Name(w1565) -> ("Date Format"=w1564:string)
              n1106 = Array Size(array=w1558) -> (size(s)=w1557:i32)
              n1107 = for {
                tunnel: w1564 -> [w1569]
                tunnel: [w1568] -> w1561 mode=indexing
                tunnel: w1563 -> [w1567] mode=indexing
                n1108 = Format Date/Time String(time format string (%c)=w1569, seconds (now)=w1567) -> (date/time string=w1568:string)  [unwired: 1 in]
              }
              n1109 = Number To Fractional String(number=w1562) -> (F-format string=w1560:string[])  [unwired: 3 in]
              n1110 = Number To Fractional String(number=w1558) -> (F-format string=w1559:string[])  [unwired: 3 in]
              n1111 = Build Array(w1561, w1560, w1559) -> (w1554:string[][])
              n1112 = Build Array (concatenate)(w1556, w1554) -> (w1555:string[][])
            }
            n1113 = Array Max & Min(array=w1551) -> ()  [unwired: 4 out]
            n1114 = call "Write To Spreadsheet File (string) w Error.vi"("transpose? (no:F)"=TRUE, "2D data"=w1549, "file path (dialog if empty)"=w1552) -> ()  [unwired: 7 in, 2 out]
          }
          frame True {
          }
        }
      }
      event "Plot-save-screen": Value Change {
        n1115 = event-data() -> ()  [unwired: 1 in, 6 out]
        n1116 = property on="Log Files Folder" class="Path"() -> ("Value"=w1575:path)  [unwired: 2 in, 2 out]
        n1117 = call "File Dialog7"("start path"=w1575, "pattern (all files)"="*.dat", "pattern label"="Log files") -> ("selected path"=w1573:path, "cancelled"=w1574:bool)  [unwired: 9 in, 2 out]
        n1118 = case shown="False" w1574 {
          tunnel: w1573 -> [w1600 _]
          frame False {
            # "!!NOTE:This routine assumes that XY graph is \ncontrol #0 on tab page!!"
            n1119 = property on="Channels Panel" class="TabCtl (strict)"() -> ("Pages"=w1598:refnum<vi>[], "Value"=w1597:T8)  [unwired: 2 in, 2 out]
            n1120 = Index Array(array=w1598, index=w1597) -> (element=w1596:refnum<vi>)
            n1121 = property class="Page"(reference=w1596) -> ("ControlsOnPage"=w1593:refnum<vi>[])  [unwired: 1 in, 2 out]
            n1122 = Index Array(array=w1593, index=0) -> (element=w1595:refnum<vi>)
            n1123 = control-ref of="R-Plot 0"() -> (w1591:refnum<vi>)
            n1124 = Type Cast(type=w1591, x=w1595) -> (*(type *) &x=w1592:refnum<vi>)
            n1125 = property class="XYGraph (strict)"(reference=w1592) -> ("Value"=w1590:cluster{dbl[], dbl[]}, "XScale.Maximum"=w1589:dbl, "XScale.Minimum"=w1588:dbl)  [unwired: 1 in, 2 out]
            n1126 = Unbundle(w1590) -> (w1587:dbl[], w1586:dbl[])
            n1127 = call "MGI Threshold 1D Array Extended.vi"("Threshold Y"=w1589, "Y Value[]"=w1587) -> ("Extended Fractional Index"=w1577:dbl)  [unwired: 1 in]
            n1128 = call "MGI Threshold 1D Array Extended.vi"("Threshold Y"=w1588, "Y Value[]"=w1587) -> ("Extended Fractional Index"=w1576:dbl)  [unwired: 1 in]
            n1129 = Subtract(x=w1577, y=w1576) -> (x-y=w1599:dbl)
            n1130 = Array Subset(array=w1587, index=w1576, length=w1599) -> (w1581:dbl[])
            n1131 = Array Subset(array=w1586, index=w1576, length=w1599) -> (w1579:dbl[])
            n1132 = property on="Data Logging Settings" class="Clust (strict)"() -> ("Value"=w1583:T37)  [unwired: 2 in, 2 out]
            n1133 = Unbundle By Name(w1583) -> ("Date Format"=w1582:string)
            n1134 = Number To Fractional String(number=w1579) -> (F-format string=w1578:string[])  [unwired: 3 in]
            n1135 = for {
              tunnel: w1582 -> [w1603]
              tunnel: [w1602] -> w1580 mode=indexing
              tunnel: w1581 -> [w1601] mode=indexing
              n1136 = Format Date/Time String(time format string (%c)=w1603, seconds (now)=w1601) -> (date/time string=w1602:string)  [unwired: 1 in]
            }
            n1137 = Build Array(w1580, w1578) -> (w1585:string[][])
            n1138 = call <vilib>:"Write To Spreadsheet File (string).vi"("transpose? (no:F)"=TRUE, "2D data"=w1585, "file path (dialog if empty)"=w1600) -> ()  [unwired: 5 in, 1 out]
          }
          frame True {
          }
        }
      }
      event "Plot-Save All": Value Change {
        n1139 = event-data() -> ()  [unwired: 1 in, 6 out]
        n1140 = property on="Log Files Folder" class="Path"() -> ("Value"=w1609:path)  [unwired: 2 in, 2 out]
        n1141 = call "File Dialog8"("start path"=w1609, "pattern (all files)"="*.dat", "pattern label"="Log files") -> ("selected path"=w1607:path, "cancelled"=w1608:bool)  [unwired: 9 in, 2 out]
        n1142 = case shown="False" w1608 {
          tunnel: w1607 -> [w1627 _]
          frame False {
            # "!!NOTE:This routine assumes that XY graph is \ncontrol #0 on tab page!!"
            n1143 = property on="Channels Panel" class="TabCtl (strict)"() -> ("Pages"=w1626:refnum<vi>[], "Value"=w1625:T8)  [unwired: 2 in, 2 out]
            n1144 = Index Array(array=w1626, index=w1625) -> (element=w1624:refnum<vi>)
            n1145 = property class="Page"(reference=w1624) -> ("ControlsOnPage"=w1621:refnum<vi>[])  [unwired: 1 in, 2 out]
            n1146 = Index Array(array=w1621, index=0) -> (element=w1623:refnum<vi>)
            n1147 = control-ref of="R-Plot 0"() -> (w1619:refnum<vi>)
            n1148 = Type Cast(type=w1619, x=w1623) -> (*(type *) &x=w1620:refnum<vi>)
            n1149 = property class="XYGraph (strict)"(reference=w1620) -> ("Value"=w1618:cluster{dbl[], dbl[]})  [unwired: 1 in, 2 out]
            n1150 = Unbundle(w1618) -> (w1611:dbl[], w1610:dbl[])
            n1151 = property on="Data Logging Settings" class="Clust (strict)"() -> ("Value"=w1615:T37)  [unwired: 2 in, 2 out]
            n1152 = Unbundle By Name(w1615) -> ("Date Format"=w1614:string)
            n1153 = Number To Fractional String(number=w1610) -> (F-format string=w1612:string[])  [unwired: 3 in]
            n1154 = for {
              tunnel: w1614 -> [w1630]
              tunnel: [w1629] -> w1613 mode=indexing
              tunnel: w1611 -> [w1628] mode=indexing
              n1155 = Format Date/Time String(time format string (%c)=w1630, seconds (now)=w1628) -> (date/time string=w1629:string)  [unwired: 1 in]
            }
            n1156 = Build Array(w1613, w1612) -> (w1617:string[][])
            n1157 = call <vilib>:"Write To Spreadsheet File (string).vi"("transpose? (no:F)"=TRUE, "2D data"=w1617, "file path (dialog if empty)"=w1627) -> ()  [unwired: 5 in, 1 out]
          }
          frame True {
          }
        }
      }
      event "_CurrentsChanged": Value Change {
        # "New values for currents were entered by user/automode-> write new data to CS"
        n1158 = event-data() -> ()  [unwired: 1 in, 6 out]
        n1159 = local read "_CSClassRef"() -> (w1636:refnum<class "CS.lvclass">)
        n1160 = property on="CS status" class="Clust (strict)"() -> ("Value"=w1633:errorcluster)  [unwired: 2 in, 2 out]
        n1161 = call-dynamic "Read.vi"("CS in"=w1636, "error in (no error)"=w1633, "Optional"=TRUE ("Unused")) -> ("CS out"=w1635:refnum<class "CS.lvclass">, "error out"=w1632:errorcluster)  [unwired: 11 in, 4 out]
        n1162 = local write "_CSClassRef"(w1635) -> ()
        n1163 = property on="CS status" class="Clust (strict)"("Value"=w1632) -> ()  [unwired: 2 in, 2 out]
      }
      event "CS.QCS I0 Output": Value Change {
        # "Switch QCS channel 0 to aux output"
        n1164 = event-data() -> ("OldVal"=w1644:T38, "NewVal"=w1639:T38)  [unwired: 1 in, 4 out]
        n1165 = To Long Integer(number=w1639) -> (32bit integer=→"QCS. I0 Mapping":i32)
        n1166 = local read "_CSClassRef"() -> (w1642:refnum<class "CS.lvclass">)
        n1167 = property on="CS status" class="Clust (strict)"() -> ("Value"=w1643:errorcluster)  [unwired: 2 in, 2 out]
        n1168 = call-dynamic "Switch Output Channel.vi"("error in (no error)"=w1643, "New Channel"=w1639, "Old Channel"=w1644, "CS in"=w1642) -> ("error out"=w1640:errorcluster, "CS out"=w1641:refnum<class "CS.lvclass">)  [unwired: 6 in]
        n1169 = local write "_CSClassRef"(w1641) -> ()
        n1170 = property on="CS status" class="Clust (strict)"("Value"=w1640) -> ()  [unwired: 2 in, 2 out]
      }
      event "T Sweep.Start": Value Change {
        # "Setup and Start Current/Temperature sweep for CS channel 3"
        n1171 = event-data() -> ("CtlRef"=w1646:refnum<vi>, "NewVal"=w1647:bool)  [unwired: 1 in, 4 out]
        n1172 = case shown="False" w1647 {
          tunnel: w1646 -> [w1648 w1651]
          frame False {
            n1173 = property class="Bool (strict)"(reference=w1648, "Caption.Text"="Start") -> ()  [unwired: 1 in, 2 out]
          }
          frame True {
            n1174 = property on="Start value" class="DigNum (strict)"() -> ("Value"=w1652:dbl)  [unwired: 2 in, 2 out]
            n1175 = property class="Bool (strict)"(reference=w1651, "Caption.Text"="Stop") -> ()  [unwired: 1 in, 2 out]
            n1176 = property on="Current" class="DigNum (strict)"("Val(Sgnl)"=w1652) -> ()  [unwired: 2 in, 2 out]
          }
        }
      }
      event "T Sweep.I_next": Value Change {
        # "Go to next step in Current/Temperature sweep for CS channel 3"
        n1177 = event-data() -> ()  [unwired: 1 in, 6 out]
        n1178 = property on="I_next" class="Bool (strict)"("Value"=FALSE) -> ()  [unwired: 2 in, 2 out]
        n1179 = call "Current Time(double).vi"() -> ("Current Time (double)"=w1654:dbl)  [unwired: 6 in, 1 out]
        n1180 = local write "_TimeOld"(w1654) -> ()
        n1181 = property on="Current" class="DigNum (strict)"() -> ("Value"=w1655:dbl)  [unwired: 2 in, 2 out]
        n1182 = property on="Step" class="DigNum (strict)"() -> ("Value"=w1660:dbl)  [unwired: 2 in, 2 out]
        n1183 = Add(x=w1655, y=w1660) -> (x+y=w1659:dbl)
        n1184 = property on="End value" class="DigNum (strict)"() -> ("Value"=w1658:dbl)  [unwired: 2 in, 2 out]
        n1185 = property on="Start value" class="DigNum (strict)"() -> ("Value"=w1657:dbl)  [unwired: 2 in, 2 out]
        n1186 = In Range and Coerce(upper limit=w1658, x=w1659, lower limit=w1657) -> (coerced(x)=w1656:dbl)  [unwired: 1 out]
        n1187 = property on="Current" class="DigNum (strict)"("Val(Sgnl)"=w1656) -> ()  [unwired: 2 in, 2 out]
      }
      event "T Sweep.I_prev": Value Change {
        # "Go to previous step in Current/Temperature sweep for CS channel 3"
        n1188 = event-data() -> ()  [unwired: 1 in, 6 out]
        n1189 = call "Current Time(double).vi"() -> ("Current Time (double)"=w1663:dbl)  [unwired: 6 in, 1 out]
        n1190 = property on="I_prev" class="Bool (strict)"("Value"=FALSE) -> ()  [unwired: 2 in, 2 out]
        n1191 = local write "_TimeOld"(w1663) -> ()
        n1192 = property on="Current" class="DigNum (strict)"() -> ("Value"=w1665:dbl)  [unwired: 2 in, 2 out]
        n1193 = property on="Step" class="DigNum (strict)"() -> ("Value"=w1670:dbl)  [unwired: 2 in, 2 out]
        n1194 = Subtract(x=w1665, y=w1670) -> (x-y=w1669:dbl)
        n1195 = property on="End value" class="DigNum (strict)"() -> ("Value"=w1668:dbl)  [unwired: 2 in, 2 out]
        n1196 = property on="Start value" class="DigNum (strict)"() -> ("Value"=w1667:dbl)  [unwired: 2 in, 2 out]
        n1197 = In Range and Coerce(upper limit=w1668, x=w1669, lower limit=w1667) -> (coerced(x)=w1666:dbl)  [unwired: 1 out]
        n1198 = property on="Current" class="DigNum (strict)"("Val(Sgnl)"=w1666) -> ()  [unwired: 2 in, 2 out]
      }
      event User Event {
        # "Reset the PID loop"
        n1199 = event-data() -> ()  [unwired: 1 in, 5 out]
        n1200 = local write "CS.Mode1.PID Error"(0.0 ("T_error")) -> ()
      }
      event "Minimize UI 1", "Minimize UI 2": Value Change {
        (unwired) 29 ("Splitter Position")
        (unwired) 534 ("Numeric 2")
        # "Shrink/restore the program window"
        # "726"
        # "222"
        # "1243"
        # "816"
        n1201 = event-data() -> ()  [unwired: 1 in, 6 out]
        n1202 = case shown="True" "Minimize UI 1" {
          tunnel: "Minimize UI 2" -> [_ w1701]
          frame True {
            (unwired) T54."Disabled" ("Value")
            n1203 = property on="CS type" class="Enum (strict)"() -> ("Value"=w1687:T57)  [unwired: 2 in, 2 out]
            n1204 = property on="Bridge Type" class="Enum (strict)"() -> ("Value"=w1682:T61)  [unwired: 2 in, 2 out]
            n1205 = Equal?(x=w1682, y=T54."Disabled" ("Value")) -> (x = y?=w1680:bool)
            n1206 = Equal?(x=w1687, y=T57."Disabled" ("Value")) -> (x = y?=w1686:bool)
            n1207 = property on="Data History/RT Settings" class="TabCtl (strict)"("Value"=enum32{"History", "Settings"}."History" ("Data History")) -> ()  [unwired: 2 in, 2 out]
            n1208 = Exclusive Or(1:w1680, 2:w1686) -> (0:w1679:bool)
            n1209 = property on="Mode Buttons" class="RadioBtnsControl (strict)"("Disabled"=u8 2, "Val(Sgnl)"=T56."No Selection" ("Value (Signaling)")) -> ()  [unwired: 2 in, 2 out]
            n1210 = property class="VI"() -> ("Front Panel.PanelBounds"=w1689:T73)  [unwired: 2 in, 2 out]
            n1211 = Select(t=i16 105 ("y"), s=w1679, f=i16 169 ("y")) -> (s? t:f=w1683:i16)
            n1212 = Unbundle By Name(w1689) -> ("Left"=w1695:i16, "Top"=w1692:i16)
            n1213 = property on="Splitter 3" class="Splitter"("Position"=29 ("Splitter Position")) -> (error out=w1681:errorcluster)  [unwired: 2 in, 1 out]
            n1214 = Add(x=i16 806 ("right"), y=w1695) -> (x+y=w1694:i16)
            n1215 = Add(x=w1692, y=w1683) -> (x+y=w1691:i16)
            n1216 = Bundle By Name(cluster=w1689, "Right"=w1694, "Bottom"=w1691) -> (w1696:T73)
            n1217 = case shown="True" w1680 {
              tunnel: w1681 -> [_ w1699]
              frame False {
              }
              frame True {
                n1218 = property on="Splitter 4" class="Splitter"(error in=w1699, "Position"=32 ("Splitter Position")) -> ()  [unwired: 1 in, 2 out]
              }
            }
            n1219 = property class="VI"("Front Panel.PanelBounds"=w1696) -> ()  [unwired: 2 in, 2 out]
          }
          frame False {
            n1220 = property class="VI"() -> ("Front Panel.PanelBounds"=w1708:T73)  [unwired: 2 in, 2 out]
            n1221 = property on="Channels Panel" class="TabCtl (strict)"() -> ("Value"=w1716:T8)  [unwired: 2 in, 2 out]
            n1222 = Unbundle By Name(w1708) -> ("Left"=w1714:i16, "Top"=w1712:i16)
            n1223 = property on="Channels Panel" class="TabCtl (strict)"("Val(Sgnl)"=w1716) -> ()  [unwired: 2 in, 2 out]
            n1224 = Select(t=i16 806 ("right"), s=w1701, f=i16 1206 ("right")) -> (s? t:f=w1705:i16)
            n1225 = Add(x=w1705, y=w1714) -> (x+y=w1713:i16)
            n1226 = Add(x=w1712, y=i16 702) -> (x+y=w1710:i16)
            n1227 = Bundle By Name(cluster=w1708, "Right"=w1713, "Bottom"=w1710) -> (w1715:T73)
            n1228 = property on="Mode Buttons" class="RadioBtnsControl (strict)"("Disabled"=u8 0) -> ()  [unwired: 2 in, 2 out]
            n1229 = property class="VI"("Front Panel.PanelBounds"=w1715) -> (error out=w1702:errorcluster)  [unwired: 2 in, 1 out]
            n1230 = property on="Splitter 3" class="Splitter"(error in=w1702, "Position"=559 ("Splitter Position")) -> (error out=w1706:errorcluster)  [unwired: 1 in, 1 out]
            n1231 = property on="Splitter 4" class="Splitter"(error in=w1706, "Position"=635 ("Splitter Position")) -> ()  [unwired: 1 in, 2 out]
          }
        }
        n1232 = property on="Splitter 2" class="Splitter"("Position"=805 ("Splitter Position")) -> ()  [unwired: 2 in, 2 out]
      }
      event "Copy to Clipboard": Value Change {
        # "Copy current values to the clipboard"
        n1233 = event-data() -> ()  [unwired: 1 in, 6 out]
        n1234 = property on="_ScanData" class="Arr (strict)"() -> ("Value"=w1722:dbl[])  [unwired: 2 in, 2 out]
        n1235 = property on="T Array" class="Arr (strict)"() -> ("Value"=w1721:dbl[])  [unwired: 2 in, 2 out]
        n1236 = Build Array(w1722, w1721) -> (w1720:dbl[][])
        n1237 = Transpose 2D Array(2D array=w1720) -> (transposed array=w1719:dbl[][])
        n1238 = Array To Spreadsheet String(delimiter (Tab)="\t", array=w1719, 3:"%.4g" ("format string")) -> (spreadsheet string=w1725:string)
        n1239 = invoke class="App" method="Clipboard.Write"("Param 0"=w1725) -> ()  [unwired: 3 in, 4 out]
      }
      event "Show PID graph?": Value Change {
        # "Display plots with the PID parameters vs time for debugging"
        n1240 = event-data() -> ("NewVal"=w1727:bool)  [unwired: 1 in, 5 out]
        n1241 = property on="Channels Panel" class="TabCtl (strict)"() -> ("Pages"=w1730:refnum<vi>[])  [unwired: 2 in, 2 out]
        n1242 = Reverse 1D Array(array=w1730) -> (reversed array=w1729:refnum<vi>[])
        n1243 = Index Array(array=w1729) -> (element=w1728:refnum<vi>)  [unwired: 1 in]
        n1244 = property class="Page"(reference=w1728, "PageVis"=w1727) -> ()  [unwired: 1 in, 2 out]
      }
      event "I0.uA", "I1.uA", "I2.uA", "I3.uA": Mouse Up {
        # "Show curent edit filed on double clicking the current indicator. Set the field to the actual current value."
        n1245 = event-data() -> ("Mods.Double Click"=w1733:bool, "CtlRef"=w1732:refnum<vi>)  [unwired: 1 in, 5 out]
        n1246 = case shown="True" w1733 {
          tunnel: w1732 -> [_ w1744]
          frame False {
          }
          frame True {
            w1740 = TRUE ("Visible")
            n1247 = property class="Str"(reference=w1744) -> ("Owner"=w1743:refnum<vi>)  [unwired: 1 in, 2 out]
            n1248 = control-ref of="uA 0"() -> (w1750:refnum<vi>)
            n1249 = control-ref of="uA 1"() -> (w1753:refnum<vi>)
            n1250 = control-ref of="uA 2"() -> (w1752:refnum<vi>)
            n1251 = control-ref of="uA 3"() -> (w1751:refnum<vi>)
            n1252 = control-ref of="I0"() -> (w1741:refnum<vi>)
            n1253 = control-ref of="I1"() -> (w1747:refnum<vi>)
            n1254 = control-ref of="I2"() -> (w1746:refnum<vi>)
            n1255 = control-ref of="I3"() -> (w1739:refnum<vi>)
            n1256 = property on="CS.Current Value" class="Arr (strict)"() -> ("Value"=w1738:dbl[])  [unwired: 2 in, 2 out]
            n1257 = Type Cast(type=w1739, x=w1743) -> (*(type *) &x=w1742:refnum<vi>)
            n1258 = Build Array(w1750, w1753, w1752, w1751) -> (w1749:refnum<vi>[])
            n1259 = Build Array(w1741, w1747, w1746, w1739) -> (w1745:refnum<vi>[])
            n1260 = Search 1D Array(1D array=w1745, element=w1742) -> (index of element=w1737:i32)  [unwired: 1 in]
            n1261 = Index Array(array=w1738, index=w1737) -> (element=w1736:dbl)
            n1262 = Index Array(array=w1749, index=w1737) -> (element=w1748:refnum<vi>)
            n1263 = Multiply(x=1000.0, y=w1736) -> (x*y=w1735:dbl)
            n1264 = property on="Property Node" class="DigNum (strict)"(reference=w1748, "Value"=w1735, "Visible"=w1740, "Key Focus"=w1740) -> ()  [unwired: 1 in, 2 out]
          }
        }
      }
      event "I0.current flows", "I1.current flows", "I2.current flows", "I3.current flows": Mouse Up {
        # "Toggle the current channel by double clickin on the \"On\" led in the current indicator."
        n1265 = event-data() -> ("CtlRef"=w1755:refnum<vi>, "Mods.Double Click"=w1756:bool)  [unwired: 1 in, 5 out]
        n1266 = case shown="True" w1756 {
          tunnel: w1755 -> [_ w1765]
          frame False {
          }
          frame True {
            n1267 = control-ref of="current flows"() -> (w1770:refnum<vi>)
            n1268 = control-ref of="current flows"() -> (w1769:refnum<vi>)
            n1269 = control-ref of="current flows"() -> (w1768:refnum<vi>)
            n1270 = control-ref of="current flows"() -> (w1767:refnum<vi>)
            n1271 = control-ref of="Toggle ON/OFF"() -> (w1764:refnum<vi>)
            n1272 = control-ref of="Toggle ON/OFF"() -> (w1762:refnum<vi>)
            n1273 = control-ref of="Toggle ON/OFF"() -> (w1761:refnum<vi>)
            n1274 = control-ref of="Toggle ON/OFF"() -> (w1763:refnum<vi>)
            n1275 = Build Array(w1770, w1769, w1768, w1767) -> (w1766:refnum<vi>[])
            n1276 = Build Array(w1764, w1762, w1761, w1763) -> (w1760:refnum<vi>[])
            n1277 = Search 1D Array(1D array=w1766, element=w1765) -> (index of element=w1759:i32)  [unwired: 1 in]
            n1278 = Index Array(array=w1760, index=w1759) -> (element=w1758:refnum<vi>)
            n1279 = property class="Bool (strict)"(reference=w1758, "Val(Sgnl)"=TRUE ("Value (Signaling)")) -> ()  [unwired: 1 in, 2 out]
          }
        }
      }
      event "uA 0", "uA 1", "uA 2", "uA 3": Value Change {
        w1773 = refnum<vi> refnum  # Numeric
        w1777 = refnum<vi> refnum  # Enum
        # "User has entered the current by double clicking on the current indicators at the bottom. \nSet range to \"Auto\" and interpret the entered value as [uA]"
        # "!!NOTE:This routine assumes that Current and Range are controls #2 & #3 in current control cluster"
        n1280 = event-data() -> ("CtlRef"=w1785:refnum<vi>, "NewVal"=w1772:u32)  [unwired: 1 in, 4 out]
        n1281 = control-ref of="CS.I0"() -> (w1794:refnum<vi>)
        n1282 = control-ref of="CS.I1"() -> (w1792:refnum<vi>)
        n1283 = control-ref of="CS.I2"() -> (w1793:refnum<vi>)
        n1284 = control-ref of="CS.I3"() -> (w1795:refnum<vi>)
        n1285 = control-ref of="uA 0"() -> (w1787:refnum<vi>)
        n1286 = control-ref of="uA 1"() -> (w1790:refnum<vi>)
        n1287 = control-ref of="uA 2"() -> (w1789:refnum<vi>)
        n1288 = control-ref of="uA 3"() -> (w1788:refnum<vi>)
        n1289 = Build Array(w1794, w1792, w1793, w1795) -> (w1791:refnum<vi>[])
        n1290 = Build Array(w1787, w1790, w1789, w1788) -> (w1786:refnum<vi>[])
        n1291 = Search 1D Array(1D array=w1786, element=w1785) -> (index of element=w1784:i32)  [unwired: 1 in]
        n1292 = Index Array(array=w1791, index=w1784) -> (element=w1783:refnum<vi>)
        n1293 = property class="Clust (strict)"(reference=w1783) -> ("Controls[]"=w1782:refnum<vi>[])  [unwired: 1 in, 2 out]
        n1294 = Index Array(array=w1782, index #1=3 ("index"), index #2=2 ("index")) -> (element #1=w1779:refnum<vi>, element #2=w1775:refnum<vi>)
        n1295 = Type Cast(type=w1773, x=w1775) -> (*(type *) &x=w1774:refnum<vi>)
        n1296 = Type Cast(type=w1777, x=w1779) -> (*(type *) &x=w1778:refnum<vi>)
        n1297 = property on="Property Node" class="Num"(reference=w1774, "Value"=w1772) -> ()  [unwired: 1 in, 2 out]
        n1298 = property on="Property Node" class="Enum"(reference=w1778, "Value"=T58."Auto") -> ()  [unwired: 1 in, 2 out]
      }
      event "_AVSRanges": Value Change {
        # "If user has changed the exitation, update the AVS bridge settings."
        n1299 = event-data() -> ("NewVal"=w1798:T29)  [unwired: 1 in, 5 out]
        n1300 = property on="AVS Exc&Ranges" class="Clust (strict)"() -> ("Value"=w1797:T15)  [unwired: 2 in, 2 out]
        n1301 = call "Combine Excitation&Range.vi"("Ranges"=w1798, "Exc&Ranges In"=w1797) -> ("Exc&Ranges Out"=w1799:T74)
        n1302 = property on="AVS Exc&Ranges" class="Clust (strict)"("Value"=w1799) -> ()  [unwired: 2 in, 2 out]
      }
      event Panel Close? {
        # "Ask for confirmation is user is trying to close the program"
        n1303 = event-data() -> ()  [unwired: 1 in, 4 out]
        n1304 = Two Button Dialog(message="Are you sure you want to quit the program?") -> (T button?=w1802:bool)  [unwired: 2 in]
        n1305 = Not(x=w1802) -> (.not. x?=w1803:bool)
        n1306 = event-data("Discard?"=w1803) -> ()  [unwired: 1 in, 1 out]
      }
      event "Save config": Mouse Up {
        # "Save parameters to the configuration file"
        n1307 = event-data() -> ()  [unwired: 1 in, 8 out]
        n1308 = control-ref of="CS Cannel Names"() -> (w1815:refnum<vi>)
        n1309 = control-ref of="AVS names"() -> (w1814:refnum<vi>)
        n1310 = control-ref of="_CurCalibrations"() -> (w1809:refnum<vi>)
        n1311 = control-ref of="CS.Mode1.PID"() -> (w1807:refnum<vi>)
        n1312 = control-ref of="CS.Mode1.Settings"() -> (w1806:refnum<vi>)
        n1313 = control-ref of="zBridge.Active Channels"() -> (w1808:refnum<vi>)
        n1314 = control-ref of="Bridge settings"() -> (w1820:refnum<vi>)
        n1315 = control-ref of="Runtime Settings"() -> (w1821:refnum<vi>)
        n1316 = control-ref of="CS Settings"() -> (w1819:refnum<vi>)
        n1317 = control-ref of="Sensor Calibrations"() -> (w1822:refnum<vi>)
        n1318 = control-ref of="PID setup"() -> (w1823:refnum<vi>)
        n1319 = control-ref of="Data Logging Settings"() -> (w1818:refnum<vi>)
        n1320 = call "File Dialog3"("start path"=path "C:/LC Data/Configuration" ("Relative path (.)"), "pattern (all files)"="*.ini") -> ("selected path"=w1810:path)  [unwired: 10 in, 3 out]
        n1321 = Build Array(w1808, w1820, w1821, w1819, w1818, w1822, w1823, w1815, w1814, w1809, w1807, w1806) -> (w1816:refnum<vi>[])
        n1322 = call "Save Load Settings to File by Ref with path.vi"("Array of Cluster References"=w1816, "Action"=enum8{"Load", "Save"}."Save", "error in (no error)"=w1813, "Configuration file"=w1810) -> ("error out"=w1812:errorcluster)  [unwired: 5 in]
      }
      event "Load config": Mouse Up {
        # "Load parameters from the configuration file"
        n1323 = event-data() -> ()  [unwired: 1 in, 8 out]
        n1324 = Unbundle By Name(w1827) -> ("UpdateCalibrations"=w1826:refnum<user-event>)
        n1325 = flat-sequence {
          tunnel: [w1852] -> w1837
          tunnel: w1833 -> [w1847]
          tunnel: [w1839] -> w1828
          tunnel: w1824 -> [w1838]
          tunnel: w1837 -> [w1867]
          tunnel: [w1867] -> w1836
          tunnel: [w1865] -> w1829
          tunnel: w1828 -> [w1865]
          tunnel: [w1872] -> w1835
          tunnel: w1836 -> [w1871]
          tunnel: [w1869] -> w1830
          tunnel: w1829 -> [w1869]
          tunnel: w1835 -> [w1878]
          tunnel: [w1878] -> w1834
          tunnel: [w1876] -> w1831
          tunnel: w1830 -> [w1876]
          tunnel: w1834 -> [w1882]
          tunnel: [w1881] -> w1832
          tunnel: w1831 -> [w1880]
          tunnel: w1826 -> [w1879]
          frame #0 {
            n1326 = control-ref of="zBridge.Active Channels"() -> (w1842:refnum<vi>)
            n1327 = control-ref of="Bridge settings"() -> (w1853:refnum<vi>)
            n1328 = control-ref of="Runtime Settings"() -> (w1849:refnum<vi>)
            n1329 = control-ref of="CS Settings"() -> (w1850:refnum<vi>)
            n1330 = control-ref of="Data Logging Settings"() -> (w1851:refnum<vi>)
            n1331 = control-ref of="PID setup"() -> (w1848:refnum<vi>)
            n1332 = control-ref of="CS Cannel Names"() -> (w1846:refnum<vi>)
            n1333 = control-ref of="AVS names"() -> (w1845:refnum<vi>)
            n1334 = control-ref of="_CurCalibrations"() -> (w1843:refnum<vi>)
            n1335 = control-ref of="CS.Mode1.PID"() -> (w1841:refnum<vi>)
            n1336 = control-ref of="CS.Mode1.Settings"() -> (w1840:refnum<vi>)
            n1337 = Build Array(w1842, w1853, w1849, w1850, w1851, w1848, w1846, w1845, w1843, w1841, w1840) -> (w1855:refnum<vi>[])
            n1338 = call "File Dialog2"("start path"=w1838, "pattern (all files)"="*.ini") -> ("selected path"=w1839:path)  [unwired: 10 in, 3 out]
            n1339 = call "Save Load Settings to File by Ref with path.vi"("Array of Cluster References"=w1855, "Action"=enum8{"Load", "Save"}."Load", "error in (no error)"=w1847, "Configuration file"=w1839) -> ("error out"=w1856:errorcluster)  [unwired: 5 in]
            n1340 = disable-structure shown="Disabled" {
              disable-tunnel: w1856 -> [w1859 w1864]
              disable-tunnel: [w1857 w1864] -> w1852
              frame Disabled {
                n1341 = property on="Bridge Type" class="Enum (strict)"(error in=w1859) -> (error out=w1860:errorcluster, "Value"=w1862:T61)  [unwired: 1 in, 1 out]
                n1342 = Equal To 0?(x=w1862) -> (x = 0?=w1863:bool)
                n1343 = property on="AVS GPIB Address" class="VISAName"(error in=w1860, "Visible"=w1863) -> (error out=w1861:errorcluster)  [unwired: 1 in, 1 out]
                n1344 = Not(x=w1863) -> (.not. x?=w1858:bool)
                n1345 = property on="AVS RS232 Port" class="VISAName"(error in=w1861, "Visible"=w1858) -> (error out=w1857:errorcluster)  [unwired: 1 in, 1 out]
              }
              frame Enabled {
              }
            }
          }
          frame #1 {
            n1346 = Wait (ms)(milliseconds to wait=250) -> ()  [unwired: 1 out]
          }
          frame #2 {
            n1347 = control-ref of="Sensor Calibrations"() -> (w1870:refnum<vi>)
            n1348 = control-ref of="_CurCalibrations"() -> (w1868:refnum<vi>)
            n1349 = control-ref of="Calibrations Folder"() -> (w1874:refnum<vi>)
            n1350 = control-ref of="Sensor 1"() -> (w1875:refnum<vi>)
            n1351 = control-ref of="_QuickConvertCal"() -> (w1873:refnum<vi>)
            n1352 = call "ReloadCalibrations.vi"("error in (no error)"=w1871, "Quick convert sensors"=w1873, "CurCalibrations"=w1868, "Calibration files path"=w1874, "Channel1 sensors"=w1875, "Channels list"=w1870) -> ("error out"=w1872:errorcluster)  [unwired: 1 in]
          }
          frame #3 {
            n1353 = Wait (ms)(milliseconds to wait=250) -> ()  [unwired: 1 out]
          }
          frame #4 {
            n1354 = disable-structure shown="Enabled" {
              disable-tunnel: w1882 -> [w1885 w1891]
              disable-tunnel: [w1884 w1893] -> w1881
              disable-tunnel: w1880 -> [w1883 _]
              disable-tunnel: w1879 -> [_ w1890]
              frame Enabled {
                (unwired) T75."HKEY_CURRENT_USER" ("root key (HKEY_LOCAL_MACHINE) 2")
                n1355 = control-ref of="Sensor Calibrations"() -> (w1888:refnum<vi>)
                n1356 = Build Array(w1888) -> (w1887:refnum<vi>[])
                n1357 = call "Save Load Settings to File by Ref with path.vi"("Array of Cluster References"=w1887, "subkey"="SOFTWARE\\Leiden Cryogenics\\TC" ("subkey 2"), "Action"=enum8{"Load", "Save"}."Load", "error in (no error)"=w1885, "Configuration file"=w1883) -> ("error out"=w1884:errorcluster)  [unwired: 4 in]
              }
              frame Disabled {
                n1358 = Generate User Event(user event=w1890, event data cluster="" ("event data"), error in=w1891) -> (error out=w1893:errorcluster)  [unwired: 1 in, 1 out]
              }
            }
          }
        }
        n1359 = Unbundle By Name(w1825) -> ("Config folder"=w1824:path)
      }
      event "zBridge settings": Value Change {
        # "Show parameters menu. (only for zBridge)"
        n1360 = event-data() -> ()  [unwired: 1 in, 6 out]
        n1361 = Unbundle By Name(w1896) -> ("zBridge dll"=w1894:path, "Config folder"=w1895:path)
        n1362 = disable-structure shown="Disabled" {
          disable-tunnel: w1895 -> [w1898 w1903]
          disable-tunnel: w1894 -> [w1897 w1902]
          frame Enabled {
            w1901 = 0 ("Page")
            n1363 = call "SetParFilePath.vi"("path"=w1898, "zDll"=w1897) -> ("error out"=w1899:errorcluster, "zDll out"=w1900:path)  [unwired: 8 in]
            n1364 = call "ParamMenu.vi"("error in (no error)"=w1899, "Subpage"=w1901, "Page"=w1901, "path in"=w1900) -> ()  [unwired: 6 in, 2 out]
          }
          frame Disabled {
            n1365 = call "SetParFilePath.vi"("path"=w1903, "zDll"=w1902) -> ("zDll out"=w1904:path)  [unwired: 8 in, 1 out]
            n1366 = call "zBridgeSettings_1page.vi"("zDll"=w1904) -> ()  [unwired: 10 in, 1 out]
          }
        }
      }
      event "Edit Calibrations": Value Change {
        # "Show calibration files editor. Works with .cal and .cal2 files only"
        n1367 = event-data() -> ("NewVal"=w1916:T11)  [unwired: 1 in, 5 out]
        n1368 = Unbundle By Name(w1908) -> ("UpdateCalibrations"=w1907:refnum<user-event>)
        n1369 = Cluster To Array(cluster=w1916) -> (array=w1915:bool[])
        n1370 = Unbundle By Name(w1906) -> ("Calibrations Folder"=w1905:path)
        n1371 = local read "_CurCalibrations"() -> (w1911:T33)
        n1372 = Search 1D Array(1D array=w1915, element=TRUE) -> (index of element=w1913:i32)  [unwired: 1 in]
        n1373 = Cluster To Array(cluster=w1911) -> (array=w1910:string[])
        n1374 = Index Array(array=w1910, index=w1913) -> (element=w1912:string)
        n1375 = call "Edit Calibration Coefficients.vi"("Calibration Name"=w1912, "Calibration folder"=w1905) -> ("Cancelled?"=w1909:bool)  [unwired: 1 out]
        n1376 = case shown="False" w1909 {
          tunnel: w1907 -> [w1917 _]
          frame False {
            n1377 = Generate User Event(user event=w1917, event data cluster="" ("event data")) -> ()  [unwired: 2 in, 2 out]
          }
          frame True {
          }
        }
      }
      event "Edit calibration": Value Change {
        # "Show calibration files editor for quick convert R->T. Works with .cal and .cal2 files only"
        n1378 = event-data() -> ()  [unwired: 1 in, 6 out]
        n1379 = Unbundle By Name(w1922) -> ("UpdateCalibrations"=w1921:refnum<user-event>)
        n1380 = Unbundle By Name(w1920) -> ("Calibrations Folder"=w1919:path)
        n1381 = property on="_QuickConvertCal" class="Ring (strict)"() -> ("Strings []"=w1925:string[], "Value"=w1926:u16)  [unwired: 2 in, 2 out]
        n1382 = Index Array(array=w1925, index=w1926) -> (element=w1924:string)
        n1383 = call "Edit Calibration Coefficients.vi"("Calibration Name"=w1924, "Calibration folder"=w1919) -> ("Cancelled?"=w1923:bool)  [unwired: 1 out]
        n1384 = case shown="False" w1923 {
          tunnel: w1921 -> [w1927 _]
          frame False {
            n1385 = Generate User Event(user event=w1927, event data cluster="" ("event data")) -> ()  [unwired: 2 in, 2 out]
          }
          frame True {
          }
        }
      }
      event "zBridge params.AVS Name 0", "zBridge params.AVS Name 1", "zBridge params.AVS Name 2", "zBridge params.AVS Name 3", "zBridge params.AVS Name 4", "zBridge params.AVS Name 5", "zBridge params.AVS Name 6", "zBridge params.AVS Name 7", "zBridge params.AVS Name 8", "zBridge params.AVS Name 9": Mouse Down {
        # "Show parameters menu for the channel by double clicking on \"Channel parameters\". (only for zBridge)"
        n1386 = event-data() -> ("CtlRef"=w1933:refnum<vi>, "Mods.Double Click"=w1932:bool, "PlatMods.Alt"=w1931:bool)  [unwired: 1 in, 5 out]
        n1387 = Unbundle By Name(w1930) -> ("zBridge dll"=w1929:path)
        n1388 = case shown="False" w1932 {
          tunnel: w1933 -> [w1937 w1942]
          tunnel: w1931 -> [_ w1941]
          tunnel: w1929 -> [w1934 w1940]
          frame True {
            n1389 = control-ref of="zBridge params"() -> (w1939:refnum<vi>)
            n1390 = property class="Clust (strict)"(reference=w1939) -> ("Controls[]"=w1938:refnum<vi>[])  [unwired: 1 in, 2 out]
            n1391 = Search 1D Array(1D array=w1938, element=w1937) -> (index of element=w1935:i32)  [unwired: 1 in]
            n1392 = call "ParamMenu.vi"("Subpage"=w1935, "Page"=0, "path in"=w1934) -> ()  [unwired: 7 in, 2 out]
          }
          frame False {
            n1393 = case shown="True" w1941 {
              tunnel: w1942 -> [_ w1944]
              tunnel: w1940 -> [_ w1943]
              frame False {
              }
              frame True {
                n1394 = disable-structure shown="Disabled" {
                  disable-tunnel: w1944 -> [w1947 w1951]
                  disable-tunnel: w1943 -> [w1945 _]
                  frame Disabled {
                    # "Show information window.\nTends to crash the acquisition!"
                    n1395 = control-ref of="zBridge params"() -> (w1949:refnum<vi>)
                    n1396 = property class="Clust (strict)"(reference=w1949) -> ("Controls[]"=w1948:refnum<vi>[])  [unwired: 1 in, 2 out]
                    n1397 = Search 1D Array(1D array=w1948, element=w1947) -> (index of element=w1946:i32)  [unwired: 1 in]
                    n1398 = call "Show Info Window.vi"("Data set number"=w1946, "zDll"=w1945) -> ()  [unwired: 8 in, 2 out]
                  }
                  frame Enabled {
                    # "Show information window."
                    n1399 = control-ref of="zBridge params"() -> (w1953:refnum<vi>)
                    n1400 = property class="Clust (strict)"(reference=w1953) -> ("Controls[]"=w1952:refnum<vi>[])  [unwired: 1 in, 2 out]
                    n1401 = Search 1D Array(1D array=w1952, element=w1951) -> (index of element=w1950:i32)  [unwired: 1 in]
                    n1402 = call "Scan Parameters Window.vi"("index"=w1950) -> ()  [unwired: 11 in]
                  }
                }
              }
            }
          }
        }
      }
      event "zBridge.Active Channels.active Channel 0", "zBridge.Active Channels.active Channel 1", "zBridge.Active Channels.active Channel 2", "zBridge.Active Channels.active Channel 3", "zBridge.Active Channels.active Channel 4", "zBridge.Active Channels.active Channel 5", "zBridge.Active Channels.active Channel 6", "zBridge.Active Channels.active Channel 7", "zBridge.Active Channels.active Channel 8", "zBridge.Active Channels.active Channel 9": Mouse Down {
        # "Switch channels On/Off by double clicking on \"Active\" LED. (only for zBridge and AVS47B)"
        n1403 = event-data() -> ("CtlRef"=w1958:refnum<vi>, "Mods.Double Click"=w1956:bool)  [unwired: 1 in, 6 out]
        n1404 = Unbundle By Name(w1955) -> ("zBridge dll"=w1954:path)
        n1405 = property on="Bridge Type" class="Enum (strict)"() -> ("Value"=w1957:T61)  [unwired: 2 in, 2 out]
        n1406 = case shown="True" w1956 {
          tunnel: w1958 -> [_ w1961]
          tunnel: w1957 -> [_ w1965]
          tunnel: w1954 -> [_ w1959]
          frame False {
          }
          frame True {
            n1407 = control-ref of="zBridge.Active Channels"() -> (w1964:refnum<vi>)
            n1408 = property class="Clust (strict)"(reference=w1964) -> ("Controls[]"=w1962:refnum<vi>[])  [unwired: 1 in, 2 out]
            n1409 = property class="Bool (strict)"(reference=w1961) -> ("Value"=w1960:bool)  [unwired: 1 in, 2 out]
            n1410 = Search 1D Array(1D array=w1962, element=w1961) -> (index of element=w1963:i32)  [unwired: 1 in]
            n1411 = case shown="\"Impedance Bridge\"" w1965 {
              tunnel: w1963 -> [_ w1970 w1972]
              tunnel: w1962 -> [_ w1969 _]
              tunnel: w1960 -> [_ w1966 _]
              tunnel: w1959 -> [_ _ w1971]
              frame Default {
              }
              frame "AVS47B (RS232 interface)" {
                n1412 = Index Array(array=w1969, index=w1970) -> (element=w1968:refnum<vi>)
                n1413 = Not(x=w1966) -> (.not. x?=w1967:bool)
                n1414 = property class="Ctl"(reference=w1968, "Value"=w1967) -> ()  [unwired: 1 in, 2 out]
              }
              frame "Impedance Bridge" {
                w1974 = Byte_Params."Active" ("Enum")
                # "Invert Active flag"
                n1415 = call "GetByteParam.vi"("ParNo"=w1974, "SetNo"=w1972, "zDll"=w1971) -> ("return type"=w1976:u8)  [unwired: 6 in, 2 out]
                n1416 = Decrement(x=w1976) -> (x-1=w1975:i8)
                n1417 = Absolute Value(x=w1975) -> (abs(x)=w1973:i8)
                n1418 = call "SetByteParam.vi"("SetNo"=w1972, "ParNo"=w1974, "Data"=w1973, "zDll"=w1971) -> ()  [unwired: 6 in, 2 out]
              }
            }
          }
        }
      }
      event "Small R Cluster.R0", "Small R Cluster.R1", "Small R Cluster.R2", "Small R Cluster.R3", "Small R Cluster.R4", "Small R Cluster.R5", "Small R Cluster.R6", "Small R Cluster.R7", "Small R Cluster.R8", "Small R Cluster.R9", "Small T Cluster.T0", "Small T Cluster.T1", "Small T Cluster.T2", "Small T Cluster.T3", "Small T Cluster.T4", "Small T Cluster.T5", "Small T Cluster.T6", "Small T Cluster.T7", "Small T Cluster.T8", "Small T Cluster.T9": Mouse Down {
        n1419 = event-data() -> ()  [unwired: 1 in, 8 out]
      }
      event Mouse Down {
        n1420 = event-data() -> ()  [unwired: 1 in, 8 out]
      }
      event Value Change {
        # "Update channel names on the small bottom panel when the names are changed."
        n1421 = event-data() -> ("NewVal"=→"AVS names small":T10)  [unwired: 1 in, 5 out]
      }
      event "CS.Mode1.Next": Value Change {
        # "Go to next step in CS auto mode."
        n1422 = event-data() -> ()  [unwired: 1 in, 6 out]
        n1423 = Unbundle By Name(w1984) -> ("TempStabilized"=w1983:refnum<user-event>)
        n1424 = flat-sequence {
          tunnel: w1983 -> [w1986]
          frame #0 {
            n1425 = call "Current Time(double).vi"() -> ("Current Time (double)"=w1985:dbl)  [unwired: 6 in, 1 out]
            n1426 = local write "_TimeOld"(w1985) -> ()
          }
          frame #1 {
            n1427 = Generate User Event(user event=w1986, event data cluster=TRUE ("event data")) -> ()  [unwired: 2 in, 2 out]
          }
        }
      }
      event "CS.Mode1.Auto Advance": Value Change {
        n1428 = event-data() -> ("NewVal"=w1989:bool)  [unwired: 1 in, 5 out]
        n1429 = case shown="True" w1989 {
          frame False {
          }
          frame True {
            # "Set timer to zero (01-01-1904) so the first point is set immediately, w/o wainting for time delay."
            # "If automatic mode is enabled- fire TempStabilized event to record current R,T,I values and start sweeping through TCS channels arrays"
            n1430 = disable-structure shown="Disabled" {
              frame Disabled {
                n1431 = Generate User Event(event data cluster="" ("event data")) -> ()  [unwired: 3 in, 2 out]
                "_TimeOld" <- 0.0 ("Timer")
              }
              frame Enabled {
              }
            }
          }
        }
      }
      event "CS.Mode1.Start", "CS.Mode2.Start": Value Change {
        n1432 = event-data() -> ("NewVal"=w1993:bool)  [unwired: 1 in, 5 out]
        n1433 = case shown="True" w1993 {
          frame False {
          }
          frame True {
            w1994 = TRUE
            # "Switch on the current sources."
            n1434 = property on="ON" class="Bool (strict)"() -> ("Value"=w1998:bool)  [unwired: 2 in, 2 out]
            n1435 = property on="ON" class="Bool (strict)"() -> ("Value"=w1997:bool)  [unwired: 2 in, 2 out]
            n1436 = property on="ON" class="Bool (strict)"() -> ("Value"=w1996:bool)  [unwired: 2 in, 2 out]
            n1437 = property on="ON" class="Bool (strict)"() -> ("Value"=w1995:bool)  [unwired: 2 in, 2 out]
            n1438 = Exclusive Or(1:w1998, 2:w1994) -> (0:w2002:bool)
            n1439 = Exclusive Or(1:w1997, 2:w1994) -> (0:w2000:bool)
            n1440 = Exclusive Or(1:w1996, 2:w1994) -> (0:w1999:bool)
            n1441 = Exclusive Or(1:w1995, 2:w1994) -> (0:w2001:bool)
            n1442 = property on="Toggle ON/OFF" class="Bool (strict)"("Value"=w2002) -> ()  [unwired: 2 in, 2 out]
            n1443 = property on="Toggle ON/OFF" class="Bool (strict)"("Value"=w2000) -> ()  [unwired: 2 in, 2 out]
            n1444 = property on="Toggle ON/OFF" class="Bool (strict)"("Value"=w1999) -> ()  [unwired: 2 in, 2 out]
            n1445 = property on="Toggle ON/OFF" class="Bool (strict)"("Value"=w2001) -> ()  [unwired: 2 in, 2 out]
          }
        }
      }
      event "CS.Mode1.PID.Enabled": Value Change {
        # "Enable/disable the PID loop"
        n1446 = event-data() -> ("NewVal"=w2017:bool)  [unwired: 1 in, 5 out]
        n1447 = Unbundle By Name(w2006) -> ("Reset PID loop"=w2005:refnum<user-event>)
        n1448 = call "IsDisabled.vi"("Enabled?"=w2017) -> ("Numeric"=w2020:i16)
        n1449 = Generate User Event(user event=w2005, event data cluster="" ("event data")) -> ()  [unwired: 2 in, 2 out]
        n1450 = property on="PID setup" class="Clust (strict)"("Disabled"=w2020) -> ()  [unwired: 2 in, 2 out]
        n1451 = property on="FB on" class="Enum (strict)"() -> ("Value"=w2014:enum16{"Resistance", "Temperature"})  [unwired: 2 in, 2 out]
        n1452 = property on="CS.Mode1.PID Channel" class="Enum (strict)"() -> ("Value"=w2004:enum16{"0", "1", "2", "3"})  [unwired: 2 in, 2 out]
        n1453 = property on="Enabled" class="Bool (strict)"() -> ("Value"=w2008:bool)  [unwired: 2 in, 2 out]
        n1454 = Initialize Array(FALSE, 4 ("dimension size")) -> (w2010:bool[])
        n1455 = And(x=TRUE ("new element/subarray"), y=w2008) -> (x .and. y?=w2007:bool)
        n1456 = Index Array(array=string[] ["%#_g uA", "%#_g mK"], index=w2014) -> (element=w2016:string)
        n1457 = Replace Array Subset(array=w2010, new element=w2007, index=w2004) -> (w2013:bool[])
        n1458 = local write "CS.Mode1.PID Column"(w2013) -> ()
        n1459 = Select(t=w2016, s=w2017, f="%#_g uA") -> ()  [unwired: 1 out]
      }
      event "CS.Mode1.Reset PID": Value Change {
        # "Reset the PID loop"
        n1460 = event-data() -> ()  [unwired: 1 in, 6 out]
        n1461 = Unbundle By Name(w2023) -> ("Reset PID loop"=w2022:refnum<user-event>)
        n1462 = Generate User Event(user event=w2022, event data cluster="" ("event data")) -> ()  [unwired: 2 in, 2 out]
      }
      event Value Change {
        n1463 = event-data() -> ("NewVal"=w2029:dbl)  [unwired: 1 in, 5 out]
        n1464 = Unbundle By Name(w2027) -> ("Reset PID loop"=w2026:refnum<user-event>)
        n1465 = Generate User Event(user event=w2026, event data cluster="" ("event data")) -> ()  [unwired: 2 in, 2 out]
        n1466 = property on="Enabled" class="Bool (strict)"() -> ("Value"=w2031:bool)  [unwired: 2 in, 2 out]
        n1467 = Initialize Array(FALSE, 4 ("dimension size")) -> (w2033:bool[])
        n1468 = And(x=TRUE ("new element/subarray"), y=w2031) -> (x .and. y?=w2030:bool)
        n1469 = Replace Array Subset(array=w2033, new element=w2030, index=w2029) -> (→"CS.Mode1.PID Column":bool[])
        n1470 = Index Array(array=string[] ["%#_g uA", "%#_g mK"], index=w2029) -> ()  [unwired: 1 out]
      }
      event "CS.Mode1.List": Value Change {
        n1471 = event-data() -> ("NewVal"=w2042:T23[][])  [unwired: 1 in, 5 out]
        n1472 = local read "CS.Mode1.List:Index"() -> (w2041:i32)
        n1473 = Decrement(x=w2041) -> (x-1=w2040:i32)
        n1474 = Array Size(array=w2042) -> (size(s)=w2044:i32[])
        n1475 = Index Array(array=w2044) -> (element=→"CS.Mode1.List:Count":i32)  [unwired: 1 in]
        n1476 = Index Array(array=w2042, index (row)=w2040) -> (element=→"_CSMode1List[i]":T23[])  [unwired: 1 in]
      }
      event "CS.Mode1.List": Shortcut Menu Activation? {
        n1477 = event-data() -> ()  [unwired: 1 in, 7 out]
        n1478 = event-data() -> ()  [unwired: 2 in, 1 out]
      }
      event "CS.Mode1.List": Shortcut Menu Selection (App) {
        n1479 = event-data() -> ("ItemTag"=w2047:string)  [unwired: 1 in, 7 out]
        n1480 = case shown="\"APP_SC_COPY_DATA\"" w2047 {
          frame Default {
          }
          frame "APP_SC_PASTE_DATA" {
            n1481 = invoke class="App" method="Clipboard.Read"() -> ("Read Clipbrd"=w2050:string)  [unwired: 3 in, 2 out]
            n1482 = Spreadsheet String To Array(format string="%d", spreadsheet string=w2050) -> (array=w2048:dbl[][])  [unwired: 2 in]
            n1483 = local write "CS.Mode1.List"(w2048) -> ()
          }
          frame "APP_SC_COPY_DATA" {
            n1484 = local read "CS.Mode1.List"() -> (w2053:T23[][])
            n1485 = Array To Spreadsheet String(array=w2053, 3:"%d" ("format string")) -> (spreadsheet string=w2051:string)  [unwired: 1 in]
            n1486 = invoke class="App" method="Clipboard.Write"("Param 0"=w2051) -> ()  [unwired: 3 in, 4 out]
          }
        }
      }
      event "CS.Mode1.List:To First": Value Change {
        n1487 = event-data() -> ("OldVal"=w2055:bool)  [unwired: 1 in, 5 out]
        n1488 = local write "CS.Mode1.List:To First"(w2055) -> ()
        n1489 = property on="CS.Mode1.List:Index" class="DigNum (strict)"("Val(Sgnl)"=1 ("Value (Signaling)")) -> ()  [unwired: 2 in, 2 out]
      }
      event "CS.Mode1.List:Next": Value Change {
        n1490 = event-data() -> ("OldVal"=w2058:bool)  [unwired: 1 in, 5 out]
        n1491 = local write "CS.Mode1.List:Next"(w2058) -> ()
        n1492 = local read "CS.Mode1.List:Index"() -> (w2060:i32)
        n1493 = Increment(x=w2060) -> (x+1=w2059:i32)
        n1494 = property on="CS.Mode1.List:Index" class="DigNum (strict)"("Val(Sgnl)"=w2059) -> ()  [unwired: 2 in, 2 out]
      }
      event "CS.Mode1.List:Prev": Value Change {
        n1495 = event-data() -> ("OldVal"=w2062:bool)  [unwired: 1 in, 5 out]
        n1496 = local write "CS.Mode1.List:Prev"(w2062) -> ()
        n1497 = local read "CS.Mode1.List:Index"() -> (w2064:i32)
        n1498 = Decrement(x=w2064) -> (x-1=w2063:i32)
        n1499 = property on="CS.Mode1.List:Index" class="DigNum (strict)"("Val(Sgnl)"=w2063) -> ()  [unwired: 2 in, 2 out]
      }
      event "CS.Mode1.List:Clear": Value Change {
        n1500 = event-data() -> ()  [unwired: 1 in, 6 out]
        n1501 = flat-sequence {
          frame #0 {
            n1502 = local write "CS.Mode1.List"(T23[][] [] ("I_list")) -> ()
          }
          frame #1 {
            n1503 = property on="CS.Mode1.List:To First" class="Bool (strict)"("Val(Sgnl)"=TRUE ("Value (Signaling)")) -> ()  [unwired: 2 in, 2 out]
          }
        }
      }
      event "CS.Mode1.List:Index": Value Change {
        w2089 = 10  # Lines to scroll
        n1504 = event-data() -> ("NewVal"=w2072:i32)  [unwired: 1 in, 5 out]
        n1505 = Array Size(array="CS.Mode1.List") -> (size(s)=w2075:i32[])
        n1506 = Index Array(array=w2075) -> (element=w2073:i32)  [unwired: 1 in]
        n1507 = call "Current Time(double).vi"() -> ("Current Time (double)"=w2069:dbl)  [unwired: 6 in, 1 out]
        n1508 = local write "CS.Mode1.List:Count"(w2073) -> ()
        n1509 = local write "_TimeOld"(w2069) -> ()
        n1510 = In Range and Coerce(upper limit=w2073, x=w2072, lower limit=1) -> (coerced(x)=w2070:i32)  [unwired: 1 out]
        "CS.Mode1.List:Index" <- w2070
        n1511 = Decrement(x=w2070) -> (x-1=w2071:i32)
        n1512 = Initialize Array(FALSE, w2089) -> (w2090:bool[])
        n1513 = Index Array(array="CS.Mode1.List", index (row)=w2071) -> (element=w2092:T23[])  [unwired: 1 in]
        n1514 = local write "_CSMode1List[i]"(w2092) -> ()
        n1515 = Subtract(x=w2071, y=w2089) -> (x-y=w2079:i32)
        n1516 = Increment(x=w2079) -> (x+1=w2078:i32)
        n1517 = Decrement(x=w2089) -> (x-1=w2087:i32)
        n1518 = In Range and Coerce(upper limit=inf, x=w2078, lower limit=0) -> (coerced(x)=w2077:dbl)  [unwired: 1 out]
        n1519 = In Range and Coerce(upper limit=w2087, x=w2071, lower limit=0) -> (coerced(x)=w2084:i32)  [unwired: 1 out]
        n1520 = control-ref of="CS.Mode1.List"() -> (w2082:refnum<vi>)
        n1521 = Build Array(w2077, 0 ("element")) -> (w2083:dbl[])
        n1522 = Replace Array Subset(array=w2090, new element=TRUE ("new element/subarray"), index=w2084) -> (→"CS.Mode1.Row":bool[])
        n1523 = property class="Arr (strict)"(reference=w2082, "Index Values"=w2083) -> ()  [unwired: 1 in, 2 out]
      }
      event "CS.Mode1.List:Save": Value Change {
        n1524 = event-data() -> ()  [unwired: 1 in, 6 out]
        n1525 = call "File Dialog6"() -> ("selected path"=w2096:path, "cancelled"=w2095:bool)  [unwired: 12 in, 2 out]
        n1526 = case shown="False" w2095 {
          tunnel: w2096 -> [w2097 _]
          frame False {
            n1527 = local read "CS.Mode1.List"() -> (w2099:T23[][])
            n1528 = call <vilib>:"Write To Spreadsheet File (DBL).vi"("format (%.3f)"="%.1f", "2D data"=w2099, "file path (dialog if empty)"=w2097) -> ()  [unwired: 5 in, 1 out]
          }
          frame True {
          }
        }
      }
      event "CS.Mode1.List:Load": Value Change {
        n1529 = event-data() -> ()  [unwired: 1 in, 6 out]
        n1530 = call "File Dialog5"() -> ("selected path"=w2101:path, "cancelled"=w2102:bool)  [unwired: 12 in, 2 out]
        n1531 = case shown="False" w2102 {
          tunnel: w2101 -> [w2103 _]
          frame False {
            n1532 = call <vilib>:"Read From Spreadsheet File (DBL).vi"("file path (dialog if empty)"=w2103) -> ("all rows"=w2104:dbl[][])  [unwired: 6 in, 4 out]
            n1533 = local write "CS.Mode1.List"(w2104) -> ()
          }
          frame True {
          }
        }
      }
      event "CS.Mode1.Write To Log": Value Change {
        n1534 = event-data() -> ()  [unwired: 1 in, 6 out]
        n1535 = Unbundle By Name(w2107) -> ("TempStabilized"=w2106:refnum<user-event>)
        n1536 = Generate User Event(user event=w2106, event data cluster=FALSE ("event data")) -> ()  [unwired: 2 in, 2 out]
      }
      event "CS.Mode2.Add Row": Value Change {
        n1537 = event-data() -> ()  [unwired: 1 in, 6 out]
        n1538 = call "Currents-Temp list  - add new range.vi"("List in"="CS.Mode2.List", "Array"="CS.Mode2.New Row") -> ("Sorted list out"=w2111:dbl[][])  [unwired: 3 in, 1 out]
        n1539 = local write "CS.Mode2.List"(w2111) -> ()
      }
      event "CS.Mode2.List": Shortcut Menu Selection (User) {
        n1540 = event-data() -> ("CtlRef"=w2116:refnum<vi>, "Coords"=w2115:T70, "ItemPath"=w2114:string)  [unwired: 1 in]
        n1541 = case shown="\"Erase Range\"" w2114 {
          tunnel: w2116 -> [_ w2122 _ w2128 w2129]
          tunnel: w2115 -> [_ w2121 _ _ _]
          frame Default {
          }
          frame "Erase Range" {
            (unwired) TRUE
            n1542 = call "Get Clicked Array Index.vi"("Coords"=w2121, "Array 2"=w2122) -> ("Clicked Index"=w2118:i32[])  [unwired: 9 in]
            n1543 = local read "CS.Mode2.List"() -> (w2120:dbl[][])
            n1544 = Index Array(array=w2118) -> (element=w2117:i32)  [unwired: 1 in]
            n1545 = call "Currents-Temp list - delete range.vi"("Numeric"=w2117, "I_list 2"=w2120) -> ("I_list"=w2119:dbl[][])  [unwired: 2 in]
            n1546 = local write "CS.Mode2.List"(w2119) -> ()
          }
          frame "Clear List" {
            n1547 = call "Currents-Temp list - check ranges.vi"() -> ("I_list out"=w2123:dbl[][])  [unwired: 5 in]
            n1548 = local write "CS.Mode2.List"(w2123) -> ()
          }
          frame "Copy Data" {
            n1549 = property class="Arr (strict)"(reference=w2128) -> ("Value"=w2124:dbl[][])  [unwired: 1 in, 2 out]
            n1550 = Array To Spreadsheet String(delimiter (Tab)="\t", array=w2124, 3:"%.4g" ("format string")) -> (spreadsheet string=w2127:string)
            n1551 = invoke class="App" method="Clipboard.Write"("Param 0"=w2127) -> ()  [unwired: 3 in, 4 out]
          }
          frame "Paste Data" {
            n1552 = invoke class="App" method="Clipboard.Read"() -> ("Read Clipbrd"=w2130:string)  [unwired: 3 in, 2 out]
            n1553 = Spreadsheet String To Array(delimiter (Tab)="\t", format string="%.4g", spreadsheet string=w2130) -> (array=w2133:dbl[][])  [unwired: 1 in]
            n1554 = property class="Arr (strict)"(reference=w2129, "Value"=w2133) -> ()  [unwired: 1 in, 2 out]
          }
        }
      }
      event "Graph-open popup": Value Change {
        w2145 = 128  # call and forget
        n1555 = event-data() -> ()  [unwired: 1 in, 6 out]
        n1556 = vi-ref "Graph popup.vi"() -> (w2141:refnum<vi>)
        n1557 = property class="VI"(reference=w2141) -> (error out=w2143:errorcluster, "Name"=w2144:string)  [unwired: 1 in, 1 out]
        n1558 = Open VI Reference(type specifier VI Refnum (for type only)=refnum<vi> refnum, vi path=w2144, options=w2145, error in (no error)=w2143) -> (vi reference=w2142:refnum<vi>, error out=w2136:errorcluster)  [unwired: 2 in]
        n1559 = control-ref of="Data"() -> (w2139:refnum<vi>)
        n1560 = local read "Sensor Names"() -> (w2138:T10)
        n1561 = call-by-ref "Start Asynchronous Call"(reference=w2142, error in=w2136, "Data"=w2139, "AVS names"=w2138) -> (reference out=w2137:refnum<vi>, error out=w2135:errorcluster)  [unwired: 18 in]
        n1562 = Close Reference(reference=w2137, error in (no error)=w2135) -> ()  [unwired: 1 out]
      }
      event "ColorBox": Mouse Move {
        n1563 = event-data() -> ("Coords"=w2149:T70)  [unwired: 1 in]
        n1564 = call <vilib>:"Picture to Pixmap.vi"("picture"="Colors") -> ("image data"=w2155:T69)  [unwired: 9 in, 1 out]
        n1565 = property on="Colors" class="Pict"() -> ("Position"=w2148:T77)  [unwired: 2 in, 2 out]
        n1566 = call <vilib>:"Unflatten Pixmap.vi"("image data"=w2155) -> ("24-bit pixmap"=w2150:u32[][])  [unwired: 4 in, 6 out]
        n1567 = Subtract(x=w2149, y=w2148) -> (x-y=w2153:T70)
        n1568 = Unbundle(w2153) -> ("Horizontal"=w2152:i32, "Vertical"=w2151:i32)
        n1569 = Index Array(array=w2150, index (row)=w2151, index (col)=w2152) -> (element=→"Color":u32)
      }
      event "ColorBox": Mouse Down {
        n1570 = event-data() -> ()  [unwired: 1 in, 8 out]
        n1571 = property on="ColorBox" class="TabCtl (strict)"("Visible"=FALSE) -> ()  [unwired: 2 in, 2 out]
      }
      event "Set Color": Value Change {
        n1572 = event-data() -> ()  [unwired: 1 in, 6 out]
        n1573 = property on="ColorBox" class="TabCtl (strict)"("Visible"=TRUE) -> ()  [unwired: 2 in, 2 out]
      }
    }
    "General Error" <- w70
  }
  n1574 = flat-sequence {
    tunnel: w36 -> [w2160]
    frame #0 {
      n1575 = Wait on Occurrence(2:w2160) -> ()  [unwired: 2 in, 1 out]
    }
    frame #1 {
      n1576 = while {
        i -> [w2171]
        stop <- "Stop" stop-if-true
        # "AVS/zBridge read-out"
        n1577 = case shown="False" "Pause" {
          tunnel: w2171 -> [w2174 _]
          frame False {
            # "For the first measurement set Stab.Time=12 s to do autoranging"
            n1578 = property on="Runtime Settings" class="Clust (strict)"() -> ("Value"=w2196:T27)  [unwired: 2 in, 2 out]
            n1579 = local read "zBridge.Active Channels"() -> (w2179:T21)
            n1580 = Unbundle By Name(w2196) -> ("Stabilisation Delay"=w2188:dbl, "Averages"=w2181:u16, "Last Channel"=w2195:i8, "Read AVS channels from"=w2194:i8)
            n1581 = property on="Bridge Type" class="Enum (strict)"() -> ("Value"=w2192:T61)  [unwired: 2 in, 2 out]
            n1582 = call "Split Exc&Range.vi"("Excitations 2"="AVS Exc&Ranges") -> ("Excitations"=w2185:T29, "Ranges"=w2180:T78)  [unwired: 4 in]
            n1583 = property on="_AVS_VISA" class="VISAName"() -> ("Value"=w2193:refnum<visa-resource-name>)  [unwired: 2 in, 2 out]
            n1584 = Cluster To Array(cluster=w2179) -> (array=w2178:bool[])
            n1585 = call "If First Iteration.vi"("Iteration"=w2174, "Value In"=w2188, "Default"=12.0) -> ("Value Out"=w2187:dbl)
            n1586 = case shown="\"AVS47A (GPIB interface)\"" w2192 {
              tunnel: w2193 -> [w2206 w2217 _ _ _]
              tunnel: w2187 -> [w2202 w2220 w2227 _ _]
              tunnel: w2181 -> [w2203 w2219 _ _ _]
              tunnel: w2195 -> [w2204 w2215 _ _ _]
              tunnel: w2194 -> [w2205 w2216 _ _ _]
              tunnel: w2185 -> [w2207 w2211 _ _ _]
              tunnel: [w2199 w2210 errorcluster {"status"=FALSE, "code"=0, "source"=""} ("error out") w2243 errorcluster {"status"=FALSE, "code"=0, "source"=""} ("error out")] -> w2184
              tunnel: w2180 -> [w2201 w2213 w2228 w2244 w2248]
              tunnel: TRUE ("Autorange") -> [w2197 w2214 _ _ _]
              tunnel: [w2200 w2212 w2228 w2244 w2248] -> w2177
              tunnel: [w2198 w2209 w2226 w2237 dbl[] [] ("Data array")] -> w2182
              tunnel: w2178 -> [_ w2208 _ _ _]
              tunnel: "_ScanData" -> [_ _ _ w2233 _]
              frame "AVS47A (GPIB interface)" {
                # "AVS 47 (GPIB)"
                n1587 = call "AVS47IB_do_single_scan.vi"("AVS Port"=w2206, "Stabilization Delay"=w2202, "Autorange"=w2197, "Number of Averages"=w2203, "Last Channel"=w2204, "First Channel"=w2205, "Excitations"=w2207, "Ranges"=w2201) -> ("error out"=w2199:errorcluster, "R"=w2198:dbl[], "Ranges"=w2200:T79)  [unwired: 3 in, 2 out]
              }
              frame "AVS47B (RS232 interface)" {
                # "AVS 47B (RS232)"
                n1588 = Type Cast(type=refnum<visa-resource-name> refnum ("dup VISA session"), x=w2217) -> (*(type *) &x=w2221:refnum<visa-resource-name>)
                n1589 = call "Scanner.vi"("STABILIZATION  DELAY"=w2220, "FIRST CH TO SCAN"=w2216, "LAST CH TO SCAN"=w2215, "Autorange"=w2214, "AVERAGE COUNT"=w2219, "Excitation"=w2211, "Range"=w2213, "VISA resource"=w2221, "array"=w2208) -> ("RI"=w2209:dbl[], "Range out"=w2212:T80, "error out 2"=w2210:errorcluster)  [unwired: 1 in, 3 out]
              }
              frame "AVS Emulation" {
                (unwired) dbl[] [0.0, 0.0, 0.0, 0.0] ("I")
                n1590 = local read "CS.Automode Current"() -> (w2224:T23[])
                n1591 = Multiply(x=w2227, y=u32 1000 ("milliseconds to wait")) -> (x*y=w2231:dbl)
                n1592 = Wait (ms)(milliseconds to wait=w2231) -> ()  [unwired: 1 out]
                n1593 = Index Array(array=w2224, index=3) -> ()  [unwired: 1 out]
                n1594 = property on="CS.Current Value" class="Arr (strict)"() -> ("Value"=w2230:dbl[])  [unwired: 2 in, 2 out]
                n1595 = Multiply(x=1000.0, y=w2230) -> (x*y=w2222:dbl[])
                n1596 = call "AVS Emulate.vi"("Currents"=w2222, "Sampling time"=w2227) -> ("R"=w2226:dbl[])  [unwired: 1 in, 1 out]
              }
              frame "Impedance Bridge" {
                n1597 = local read "Bridge status"() -> (w2238:errorcluster)
                n1598 = local read "_zBridgeDll"() -> (w2245:path)
                n1599 = call "Read Data from Single Channel.vi"("error in (no error)"=w2238, "zDll"=w2245) -> ("error out"=w2243:errorcluster, "Value"=w2242:dbl, "Scan parameters/Error string"=→"_zBridgeParText":string, "Set number"=w2235:u8, "Error code"=→"Error code":u8, "Unit"=→"_ZBridgeUnit":string, "ScanParameters out"=w2236:T81)  [unwired: 3 in]
                "_zBridgeSetNr" <- w2235
                n1600 = call "ScanParameters FGV.vi"("Action"=Action."Write", "index"=w2235, "ScanParameters in"=w2236) -> ()  [unwired: 8 in, 1 out]
                n1601 = Replace Array Subset(array=w2233, new element=w2242, index=w2235) -> (w2237:dbl[])
              }
              frame "Disabled", Default {
              }
            }
            "Bridge status" <- w2184
            n1602 = property on="_AVSRanges" class="Clust (strict)"("Val(Sgnl)"=w2177) -> ()  [unwired: 2 in, 2 out]
            n1603 = property on="_ScanData" class="Arr (strict)"("Val(Sgnl)"=w2182) -> ()  [unwired: 2 in, 2 out]
            n1604 = property on="Delay" class="DigNum (strict)"() -> ("Value"=w2176:u32)  [unwired: 2 in, 2 out]
            n1605 = Multiply(x=u32 1000, y=w2176) -> (x*y=w2191:u32)
            n1606 = Wait (ms)(milliseconds to wait=w2191) -> ()  [unwired: 1 out]
          }
          frame True {
          }
        }
      }
      n1607 = while {
        stop <- w2250 stop-if-true
        (unwired) errorcluster {"status"=FALSE, "code"=0, "source"=""} ("Value")
        # "Current source control"
        n1608 = property on="CS status" class="Clust (strict)"() -> ("Value"=w2249:errorcluster)  [unwired: 2 in, 2 out]
        n1609 = stacked-sequence {
          seq-local: [w2278 _ _ _] -> [_ w2287 _ _]
          seq-local: [w2277 _ _ _] -> [_ w2286 _ _]
          seq-local: [_ w2287 _ _] -> [_ _ w2297 _]
          seq-local: [_ w2285 _ _] -> [_ _ w2296 _]
          tunnel: w2249 -> [w2276 _ _ _]
          frame #0 {
            # "Write 0 instead of the actual \ncurrent value to log if there \nis no current flowing."
            # "Read current CS status"
            n1610 = local read "_CSClassRef"() -> (w2266:refnum<class "CS.lvclass">)
            n1611 = call-dynamic "Read.vi"("CS in"=w2266, "error in (no error)"=w2276, "Optional"=FALSE) -> ("CS out"=w2278:refnum<class "CS.lvclass">, "I0"=w2269:T82, "I1"=w2270:T82, "I2"=w2271:T82, "I3"=w2272:T82, "error out"=w2277:errorcluster)  [unwired: 11 in]
            n1612 = Unbundle By Name(w2269) -> ("Current (string)"=w2264:string, "I?"=w2263:bool)
            n1613 = Unbundle By Name(w2270) -> ("Current (string)"=w2279:string, "I?"=w2262:bool)
            n1614 = Unbundle By Name(w2271) -> ("Current (string)"=w2267:string, "I?"=w2261:bool)
            n1615 = Unbundle By Name(w2272) -> ("Current (string)"=w2280:string, "I?"=w2260:bool)
            n1616 = call "CS Data Converter.vi"("CS Data"=w2269) -> ("CS Indicator"=→"I0":T83)
            n1617 = call "CS Data Converter.vi"("CS Data"=w2270) -> ("CS Indicator"=→"I1":T83)
            n1618 = call "CS Data Converter.vi"("CS Data"=w2271) -> ("CS Indicator"=→"I2":T83)
            n1619 = call "CS Data Converter.vi"("CS Data"=w2272) -> ("CS Indicator"=→"I3":T83)
            n1620 = Fract/Exp String To Number(string=w2264) -> (number=w2268:dbl)  [unwired: 3 in, 1 out]
            n1621 = Fract/Exp String To Number(string=w2279) -> (number=w2275:dbl)  [unwired: 3 in, 1 out]
            n1622 = Fract/Exp String To Number(string=w2267) -> (number=w2274:dbl)  [unwired: 3 in, 1 out]
            n1623 = Fract/Exp String To Number(string=w2280) -> (number=w2273:dbl)  [unwired: 3 in, 1 out]
            n1624 = Build Array(w2263, w2262, w2261, w2260) -> (w2259:bool[])
            n1625 = Not(x=w2259) -> (.not. x?=w2255:bool[])
            n1626 = Build Array(w2268, w2275, w2274, w2273) -> (w2258:dbl[])
            "CS.Current Value" <- w2258
            n1627 = for {
              tunnel: w2255 -> [w2284] mode=indexing
              tunnel: w2258 -> [w2283] mode=indexing
              tunnel: dbl[] [0.0, 0.0, 0.0, 0.0] ("t") -> [w2282] mode=indexing
              tunnel: [w2281] -> w2256 mode=indexing
              n1628 = Select(t=w2282, s=w2284, f=w2283) -> (s? t:f=w2281:dbl)
            }
            "CS.Actual Current" <- w2256
          }
          frame #1 {
            n1629 = Wait (ms)(milliseconds to wait=100) -> ()  [unwired: 1 out]
            n1630 = call <vilib>:"Clear Errors.vi"("error in (no error)"=w2286) -> ("error out"=w2285:errorcluster)  [unwired: 6 in]
          }
          frame #2 {
            # "Only send data to CS if\nnew value was entered"
            # "Set CS status"
            n1631 = call "CS OnOff & Gated and Current & Range.vi"("I in"="CS.I0") -> ("OnOff & Gated"=w2308:T84, "Current & Range"=w2293:T85, "I out"=w2301:T86)  [unwired: 2 in]
            n1632 = call "CS OnOff & Gated and Current & Range.vi"("I in"="CS.I1") -> ("OnOff & Gated"=w2307:T84, "Current & Range"=w2292:T85, "I out"=w2298:T86)  [unwired: 2 in]
            n1633 = call "CS OnOff & Gated and Current & Range.vi"("I in"="CS.I2") -> ("OnOff & Gated"=w2304:T84, "Current & Range"=w2291:T85, "I out"=w2299:T86)  [unwired: 2 in]
            n1634 = call "CS OnOff & Gated and Current & Range.vi"("I in"="CS.I3") -> ("OnOff & Gated"=w2303:T84, "Current & Range"=w2290:T85, "I out"=w2300:T86)  [unwired: 2 in]
            n1635 = local write "CS.I0"(w2301) -> ()
            n1636 = local write "CS.I1"(w2298) -> ()
            n1637 = local write "CS.I2"(w2299) -> ()
            n1638 = local write "CS.I3"(w2300) -> ()
            n1639 = local read "CS.Automode Current"() -> (w2289:T23[])
            n1640 = Equal To 0?(x="CS.Mode") -> (x = 0?=w2294:bool)
            n1641 = call "CS_set_channels.vi"("CS in"=w2297, "Current & Range0"=w2293, "Current & Range1"=w2292, "Current & Range 2"=w2291, "Current & Range3"=w2290, "error out"=w2296, "I_automode"=w2289, "Auto?"=w2294) -> ("CS.lvclass out"=w2313:refnum<class "CS.lvclass">, "Current Changed?"=w2310:bool, "error out 2"=w2314:errorcluster)  [unwired: 9 in]
            n1642 = call-dynamic "Set Mode.vi"("CS.lvclass in"=w2313, "On&G 0"=w2308, "On&G 1"=w2307, "On&G 2"=w2304, "On&G 3"=w2303, "error in (no error)"=w2314) -> ("CS.lvclass out"=w2311:refnum<class "CS.lvclass">, "error out"=w2312:errorcluster)  [unwired: 12 in]
            n1643 = case shown="True" w2310 {
              selector: w2310 -> [_ w2315]
              frame False {
              }
              frame True {
                n1644 = property on="_CurrentsChanged" class="Bool (strict)"("Val(Sgnl)"=w2315) -> ()  [unwired: 2 in, 2 out]
              }
            }
            n1645 = local write "_CSClassRef"(w2311) -> ()
            n1646 = property on="CS status" class="Clust (strict)"("Value"=w2312) -> ()  [unwired: 2 in, 2 out]
          }
          frame #3 {
            n1647 = Wait (ms)(milliseconds to wait=100) -> ()  [unwired: 1 out]
          }
        }
        n1648 = local read "Stop"() -> (w2250:bool)
      }
      n1649 = while {
        stop <- w2163 stop-if-true
        # "zBridge status read-out"
        n1650 = property on="Bridge Type" class="Enum (strict)"() -> ("Value"=w2161:T61)  [unwired: 2 in, 2 out]
        n1651 = case shown="\"Impedance Bridge\"" w2161 {
          frame Default {
          }
          frame "Impedance Bridge" {
            n1652 = local read "_zBridgeDll"() -> (w2169:path)
            n1653 = local read "Bridge status"() -> (w2168:errorcluster)
            n1654 = call "ScanStatus.vi"("error in (no error)"=w2168, "zDll"=w2169) -> ("error out"=w2167:errorcluster, "Status"=w2165:i32, "Channel"=w2166:i32)  [unwired: 7 in]
            n1655 = local write "Bridge status"(w2167) -> ()
            n1656 = call "zBridge Format Status.vi"("Status"=w2165, "Channel"=w2166) -> ("Status"=→"zBridge.Scan Phase":T87, "Active channel"=→"zBridge.Active channel":T88)  [unwired: 2 in]
          }
        }
        n1657 = Wait (ms)(milliseconds to wait=u32 200) -> ()  [unwired: 1 out]
        n1658 = local read "Stop"() -> (w2163:bool)
      }
    }
  }
  n1659 = disable-structure shown="Disabled" {
    frame Disabled {
      w2330 = string[] ["Paste Data from Clipboard"] ("item names")
      (unwired) enum32{"Page 1"}."Page 1" ("Tab Control 4")
      n1660 = local read "CS.Automode Current"() -> (w2325:T23[])
      n1661 = local read "zBridge.Active Channels"() -> ()  [unwired: 1 in]
      n1662 = property on="Bridge Channel" class="DigNum (strict)"() -> ("Value"=w2318:i32)  [unwired: 2 in, 2 out]
      n1663 = local read item#-1() -> ()  [unwired: 1 out]
      n1664 = Index Array(array=w2325) -> (element #1=w2321:T23, element #2=w2322:T23, element #3=w2323:T23, element #4=w2324:T23)  [unwired: 4 in]
      n1665 = property class="XYGraph (strict)" props=["YScale", "Mapping Mode"]() -> ()  [unwired: 2 in, 3 out]
      n1666 = property on="I" class="DigNum (strict)"("Val(Sgnl)"=w2321) -> ()  [unwired: 2 in, 2 out]
      n1667 = property on="I" class="DigNum (strict)"("Val(Sgnl)"=w2322) -> ()  [unwired: 2 in, 2 out]
      n1668 = property on="I" class="DigNum (strict)"("Val(Sgnl)"=w2323) -> ()  [unwired: 2 in, 2 out]
      n1669 = property on="I" class="DigNum (strict)"("Val(Sgnl)"=w2324) -> ()  [unwired: 2 in, 2 out]
      n1670 = Insert Menu Items(4:4, 7:w2330, 8:w2330) -> ()  [unwired: 3 in, 3 out]
      n1671 = Equal?(y=w2318) -> (x = y?=w2317:bool)  [unwired: 1 in]
      n1672 = Equal?(x=w2318, y=-1) -> (x = y?=w2320:bool)
      n1673 = Or(x=w2317, y=w2320) -> ()  [unwired: 1 out]
      n1674 = property on="ON" class="Boolean (strict)"() -> ("Value"=w2337:bool)  [unwired: 2 in, 2 out]
      n1675 = control-ref of="zBridge.Active Channels"() -> ()  [unwired: 1 out]
      n1676 = Exclusive Or(1:w2337, 2:TRUE ("x")) -> (0:w2336:bool)
      n1677 = property on="Toggle ON/OFF" class="Bool (strict)"("Value"=w2336) -> ()  [unwired: 2 in, 2 out]
      n1678 = control-ref of="CS.Mode1.List"() -> (w2332:refnum<vi>)
      n1679 = property class="Arr (strict)"(reference=w2332) -> ("Index Values"=w2333:u32[])  [unwired: 1 in, 2 out]
      n1680 = Index Array(array=w2333) -> (element=w2334:u32)  [unwired: 1 in]
      n1681 = property on="Side Panel" class="TabCtl (strict)"() -> ("Pages"=w2338:refnum<vi>[])  [unwired: 2 in, 2 out]
      n1682 = property on="CS.Mode1.List:Index" class="DigNum (strict)"("Val(Sgnl)"=w2334) -> ()  [unwired: 2 in, 2 out]
      n1683 = Index Array(array=w2338, index=1) -> (element=w2339:refnum<vi>)
      n1684 = Generate User Event(event data cluster="" ("event data")) -> ()  [unwired: 3 in, 2 out]
      n1685 = property class="Page"(reference=w2339, "PageVis"=TRUE ("Page Visible")) -> ()  [unwired: 1 in, 2 out]
      n1686 = property on="FB on" class="Enum (strict)" props=["Value"]() -> ()  [unwired: 2 in, 3 out]
      n1687 = Initialize Array(0.0 ("element"), 4 ("dimension size")) -> (w2326:dbl[])
      n1688 = local write "CS.Automode Current"(w2326) -> ()
    }
    frame Enabled {
    }
  }
